vi "Copy of Sievert_auto_RLC-2.vi"() -> ()   [LabVIEW 2011]
uses:
  <vilib>/Utility/error.llb/DialogType.ctl
  <vilib>/DAQmx/write.llb/DAQmx Write (Digital Bool 1Line 1Point).vi
  <vilib>/DAQmx/create/channels.llb/DAQmx Create Channel (DO-Digital Output).vi
  <vilib>/DAQmx/miscellaneous.llb/DAQmx Fill In Error Info.vi
  <vilib>/Analysis/Matrix/Numeric/Conversions/Array To Matrix - RA.vi
  <vilib>/Analysis/Matrix/Numeric/Conversions/Matrix To Array - RM.vi
  <vilib>/Analysis/NI_AALPro.lvlib
  <vilib>/Analysis/Matrix/NI_Matrix.lvlib
  <vilib>/Analysis/NI_AALBase.lvlib
panel:
  out "Boolean 4":bool
  out "tempo carga":dbl[](array[numeric])
  out "PCh1":dbl[](array[numeric])
  out "output array 2":u32[](array[numeric])
  out "MEASURE C [F ]":dbl
  out "Automatico 2":dynamicdata(graph)
  out "termopar K 2":dbl format="%.3g"
  out "termopar K":string
  out "output NTC":dbl
  out "termopar K":dbl format="%.3g"
  out "path RLC_mean":path
  out "estagio 5":i32
  out "FIM":bool=TRUE
  out "limpo":i32
  in  "N fit":i32=5
  in  "ATM wait":u32
  in  "SET":i32
  in  "time subarray":dbl[](array[numeric])
  out "P cinetica mean 2":dbl format="%0.2f"
  out "T cinetica mean 3":dbl format="%0.2f"
  out "Time cinetica":dbl format="%0.2f"
  in  "T subarray 3":dbl[](array[numeric])
  in  "P T  index 2":i32
  in  "P subarray 2":dbl[](array[numeric])
  in  "Numeric":dbl=4.0
  in  "T subarray 2":dbl[](array[numeric])
  out "T cinetica mean 2":dbl format="%0.2f"
  out "P cinetica mean":dbl format="%0.2f"
  in  "P subarray":dbl[](array[numeric])
  in  "P T  index":i32
  out "T string":string
  out "P string":string
  out "path 2_cinetica":path
  out "Polynomial Coefficients 2":dbl[](array[numeric])
  out "Polynomial Coefficients":dbl[](array[numeric])
  in  "Count SET":i32=-1
  out "Set atual":i32
  out "mean pressure":dbl format="%.4p"
  out "Set number":i32
  in  "Tab Control":T1(tab)
  out "T":bool
  out "ZPf2":bool
  out "Pf2":bool
  out "Pit":bool
  out "ZPit":bool
  out "Camara":dbl(slide) scale=0.0..59.5 scale format="%#_3g"
  in  "Save manual":bool
  in  "Open Button":bool
  out "String 2":string
  in  "ATM":bool
  in  "Câmara":bool
  in  "Vácuo":bool
  in  "Entrada Gás":bool
  in  "Manual Ctrl":bool
  in  "stop":bool
  out "P-manual":dynamicdata(graph)
  in  "Clear":bool
  out "path":path
  in  "Nota":string
  in  "Sample name":string
  in  "File name":string
  out "Linear Model Graph":dbl[][](graph)
  out "Linear Model Graph 2":dbl[][](graph)
  in  "N to fit":i32=60
  out "N":i32
  out "Vácuo":bool
  out "Atm":bool
  out "Câmara":bool
  out "String_cinetica":string
  out "Vol Ref":dbl(slide) scale=0.0..60.0 scale format="%#_4f"
  out "Entrada gás":bool
  in  "Guardar\nCinetica":bool
  out "p fit":dbl format="%#_4g"
  out "T fit":dbl format="%#_4g"
  in  "Open Button 2":bool
  out "x >= y?":bool
  in  "seconds":dbl
  out "Elapsed Time (sec)":dbl format="%.1f"
  out "bar/N":dbl format="%#_4p"
  in  "correção NTC":dbl
  out "mean H2 sensor (V)":dbl format="%#_4p"
  out "Boolean 3":bool
  out "String 3":string
  out "T 2":bool
  out "ZPit 2":bool
  out "Pit 2":bool
  out "Pf2 2":bool
  out "ZPf2 2":bool
  out "Camara 2":dbl(slide) scale=0.0..20.0 scale format="%#_3g"
  out "Vácuo 2":bool
  out "Atm 2":bool
  out "Câmara 2":bool
  out "Vol Ref 3":dbl(slide) scale=0.0..25.0 scale format="%#_4f"
  out "Entrada gás 2":bool
  in  "Auto Ctrl":bool
  in  "Play Button":bool
  out "time stamp":timestamp format="%<%.2X>T"
  out "Time (sec)":dbl format="%.1f"
  in  "clear":bool
  out "Automatico":dynamicdata(graph)
  out "Linear P":T2(graph)
  out "Linear T":T2(graph)
  out "Contador":i32
  in  "STOP (bar/s)":dbl format="%#_5p"
  out "P (bar/s)":dbl format="%#_5p"
  out "bar/s":dbl format="%#_4p"
  out "P fit":dbl format="%#_4g"
  out "T fit":dbl format="%#_4g"
  out "x = y?":bool
  out "teste slope":i32
  in  "Set P auto":dbl
  in  "Step P":dbl=2.0
  in  "P_max":dbl=2.0
  in  "P_max camara":dbl=2.0
  out "Carga":bool=TRUE
  out "Descarga":bool
  out "String":string
  in  "P_min descarga":dbl
  in  "Boolean":bool
  in  "Array":dbl[](array[numeric])
  out "Boolean 2":bool
  out "Desc SET":i32
  in  "ZPf2 time":dbl=24.0
  in  "Ciclos":dbl
  out "Efetuados":dbl
  in  "patamar milliseconds to wait":u32=500
  in  "N fit patamar":i32=100
  in  "Step ZPit":dbl
  out "Read ZPit":bool
  in  "Estagio auto":i32
  out "mean H2 sensor":dbl format="%#_4p"
  in  "Ntest":i32=5
  in  "N fit 2":i32=100
  out "String 4":string
  in  "Combo Box":string(combo)
  in  "Refresh Button":bool
  in  "Close RLC 2":bool
  in  "RLC on/off":bool
  out "mean 16":dbl format="%.3p"
  out "mean 15":dbl format="%.3p"
  out "mean 14":dbl format="%.3p"
  out "mean 13":dbl format="%.3p"
  out "mean 12":dbl format="%.3p"
  out "mean 11":dbl format="%.3p"
  out "mean 10":dbl format="%.3p"
  out "mean 9":dbl format="%.3p"
  out "mean 8":dbl format="%.3p"
  out "mean 7":dbl format="%.3p"
  out "mean 6":dbl format="%.3p"
  out "mean 5":dbl format="%.3p"
  out "mean 4":dbl format="%.3p"
  out "mean 3":dbl format="%.3p"
  out "mean 2":dbl format="%.3p"
  out "mean":dbl format="%.3p"
  out "SET 2":dbl format="%#_3g"
  out "C-50-L":bool
  out "MEASURE B":dbl
  out "MEASURE A":dbl
  out "C-50-N":bool
  out "MEASURE B 2":dbl
  out "MEASURE A 2":dbl
  out "C-100-L":bool
  out "MEASURE B 3":dbl
  out "MEASURE A 3":dbl
  out "C-100-N":bool
  out "MEASURE B 4":dbl
  out "MEASURE A 4":dbl
  out "C-1K-L":bool
  out "MEASURE B 5":dbl
  out "MEASURE A 5":dbl
  out "C-1K-N":bool
  out "MEASURE B 6":dbl
  out "MEASURE A 6":dbl
  out "C-10K-L":bool
  out "MEASURE B 7":dbl
  out "MEASURE A 7":dbl
  out "C-10K-N":bool
  out "MEASURE B 8":dbl
  out "MEASURE A 8":dbl
  out "Z-50-L":bool
  out "MEASURE B 9":dbl
  out "MEASURE A 9":dbl
  out "Z-50-N":bool
  out "MEASURE B 10":dbl
  out "MEASURE A 10":dbl
  out "Z-100-L":bool
  out "MEASURE B 11":dbl
  out "MEASURE A 11":dbl
  out "Z-100-N":bool
  out "MEASURE B 12":dbl
  out "MEASURE A 12":dbl
  out "Z-1K-L":bool
  out "MEASURE B 13":dbl
  out "MEASURE A 13":dbl
  out "Z-1K-N":bool
  out "MEASURE B 14":dbl
  out "MEASURE A 14":dbl
  out "Z-10K-L":bool
  out "MEASURE B 15":dbl
  out "MEASURE A 15":dbl
  out "Z-10K-N":bool
  out "MEASURE B 16":dbl
  out "MEASURE A 16":dbl
  out "RLC300 - digimess":string
  in  "Time RLC":u32=5000
  in  "Ligar RLC":bool
  out "path RLC_completo":path
  out "Waveform Chart P 2":dbl[][](graph)
  out "Waveform Chart":dynamicdata(graph)
  in  "graph RLC":bool
  in  "Refresh Button 2":bool
  out "Waveform Chart 2":dynamicdata(graph)
  out "XY Graph 2":cluster{"Value":dbl[], "Value":dbl[]}[](graph)
  in  "t-sivert01(s)":dbl
  out "dP/dt (bar/s)":dbl format="%#_5p"
  in  "read - Sievert 01":bool
  # "P vol ref"
  # "P Câmara"
  # "P vol ref"
  # "P Câmara"
  # "C ( F )"
  # "R ( Ohm )"
  # "Z ( Ohm )"
  # "Phase ( deg)"
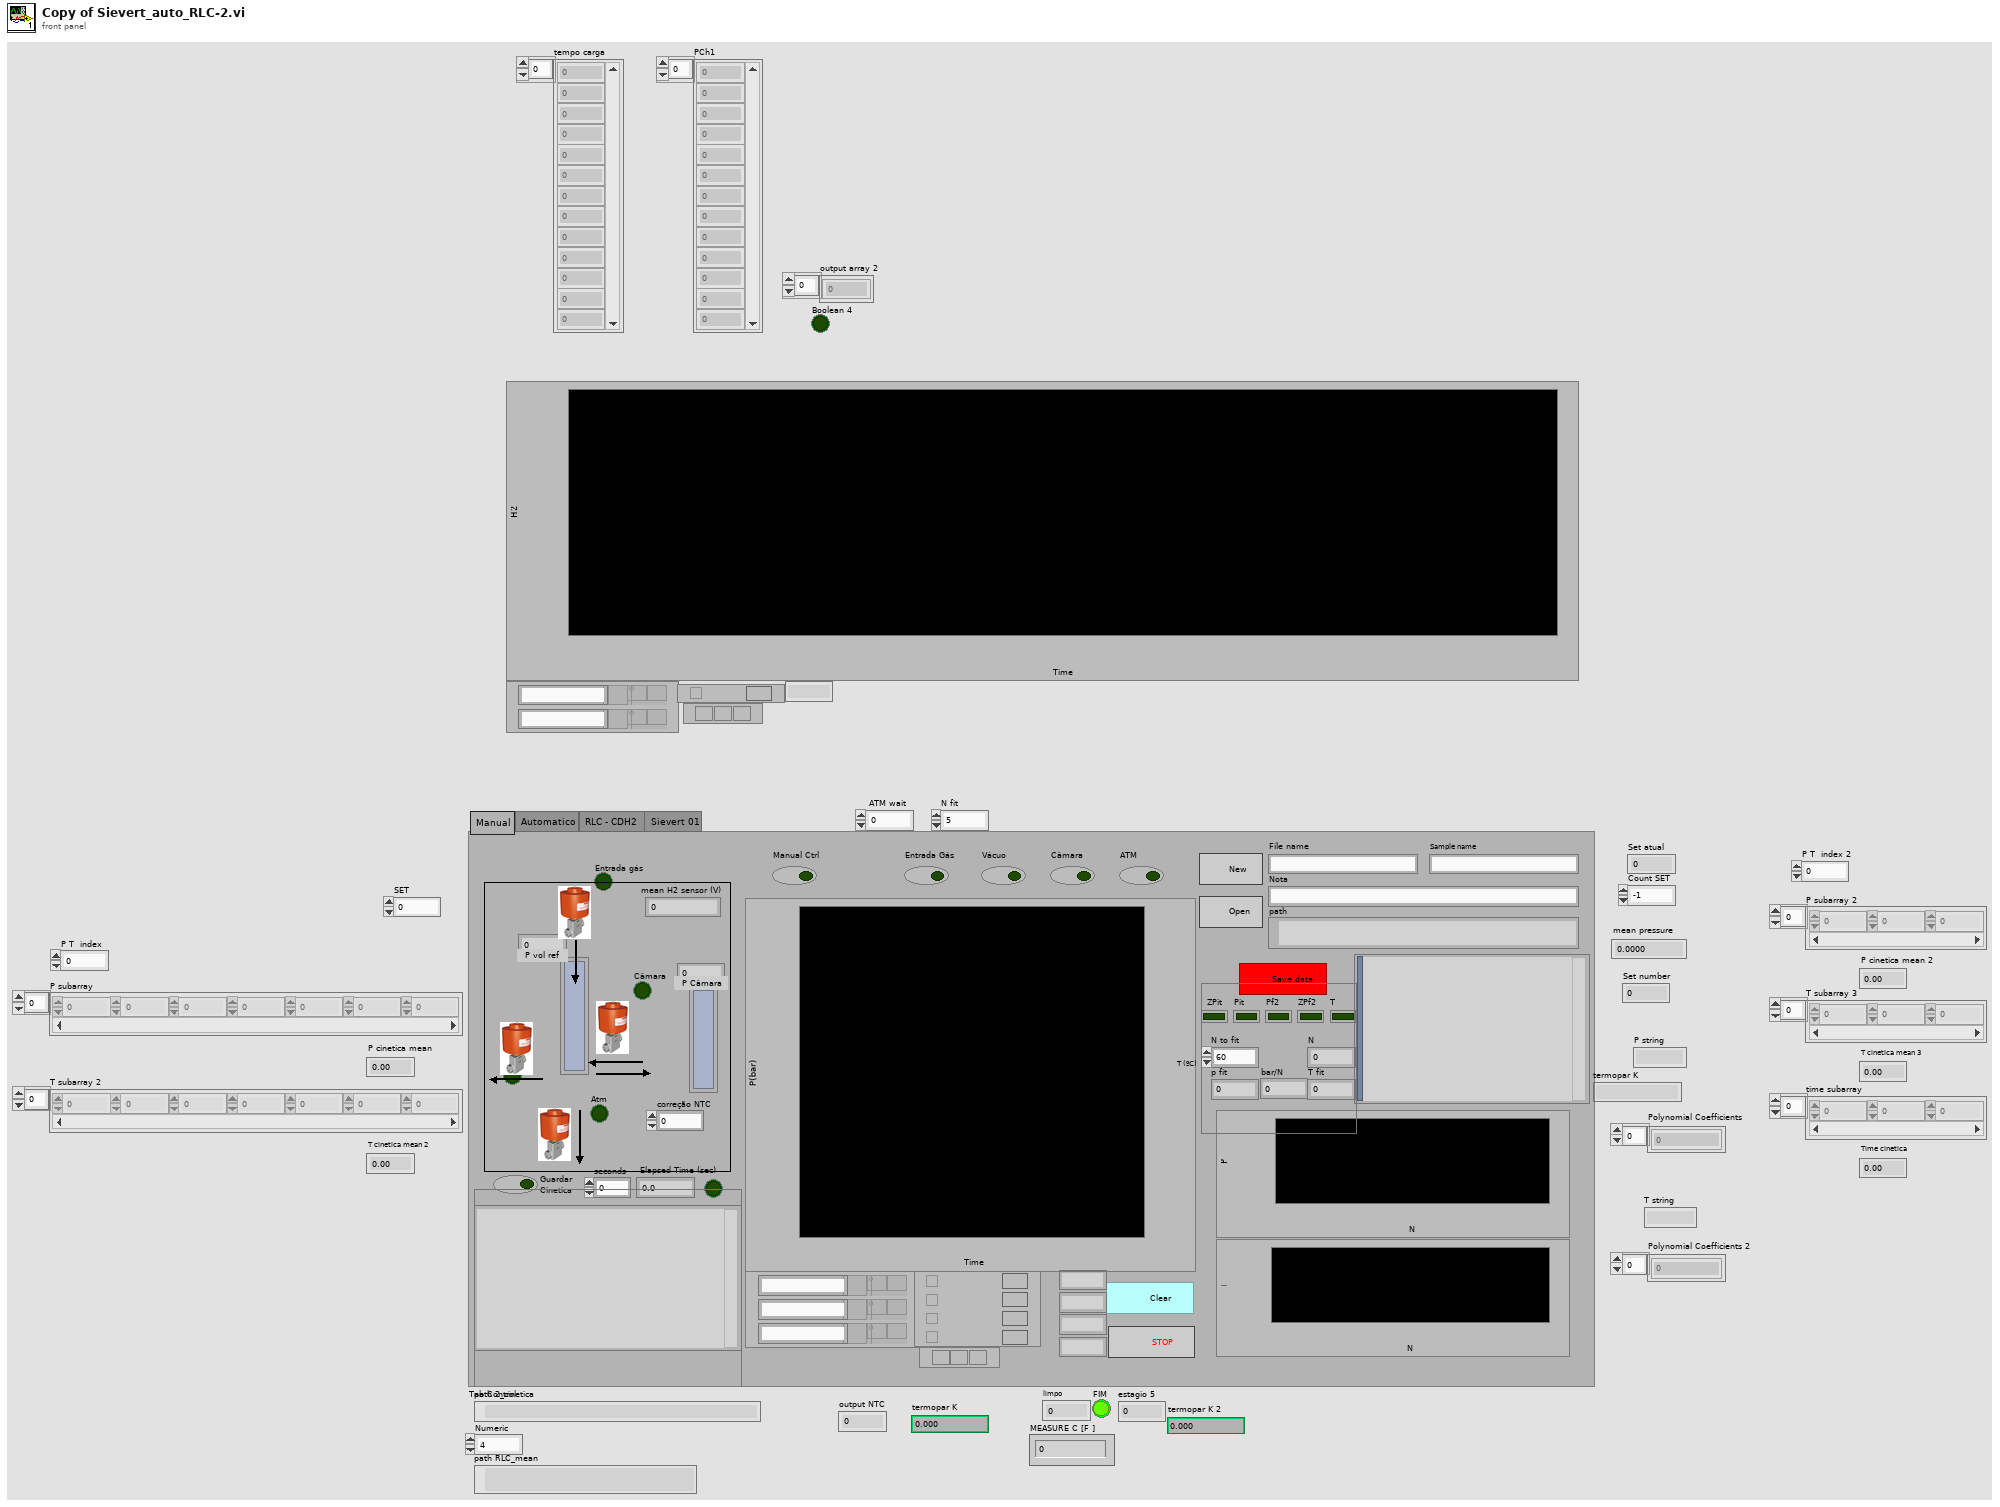
[diagram p1: front panel]
types:
  T1 = enum32{"Manual", "Automatico", "RLC - CDH2", "Sievert 01"}
  T2 = cluster{"Real 2D Array":dbl[], "Best Linear Fit":dbl[]}[]
  T3 = enum16{"open", "replace", "create", "open or create", "replace or create", "replace or create with confirmation"}
  T4 = cluster{"Value":dbl[], "Best Linear Fit":dbl[]}[]
  T5 = typedef "NI_Matrix.lvlib/RealMatrix.ctl" = dbl[][]
  T6 = cluster{"Real 2D Array":dbl[], "Real 2D Array":dbl[]}
  T7 = typedef "DialogType.ctl" = u16
  T8 = cluster{"Real 2D Array":dbl[], "Best Linear Fit":dbl[]}
  T9 = cluster{"Real 2D Array":dbl[], "Best Polynomial Fit":dbl[]}
  T10 = cluster{"Real 2D Array":dbl[], "Best Polynomial Fit":dbl[]}[]
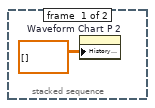
[diagram p5: hidden frame]
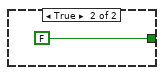
[diagram p10: hidden frame]
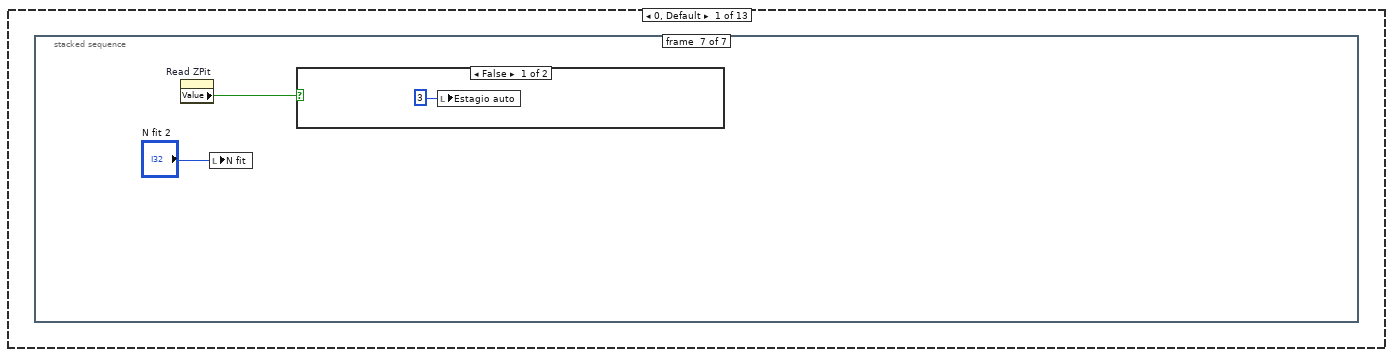
[diagram p15: hidden frame]
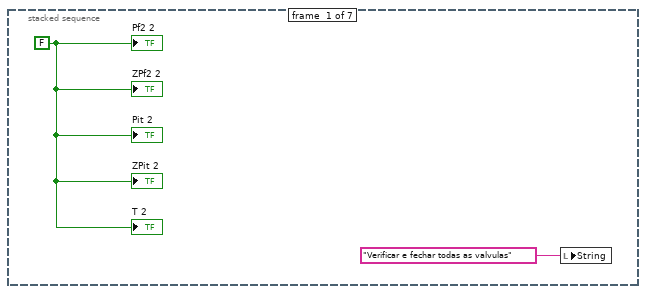
[diagram p16: hidden frame]
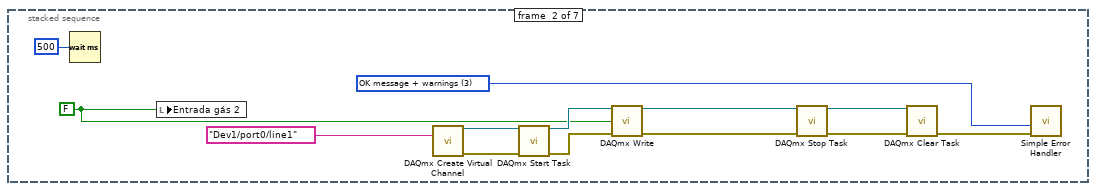
[diagram p17: hidden frame]
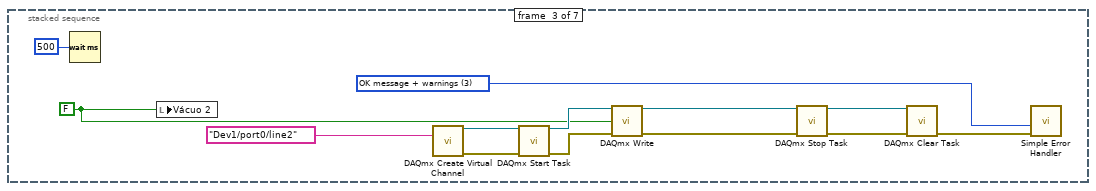
[diagram p18: hidden frame]
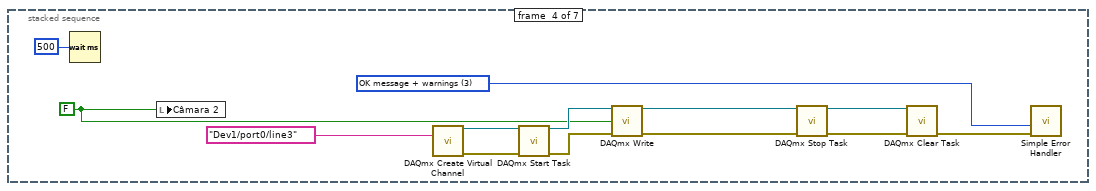
[diagram p19: hidden frame]
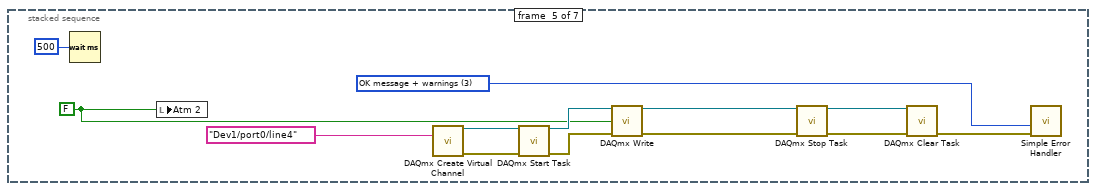
[diagram p20: hidden frame]
diagram:
  (unwired) dbl[] [0.5, 1.0, 2.0, 3.0, 4.0, 5.0, 6.0, 7.0, 8.0, 9.0, 10.0, 11.0, 12.0, 13.0, 14.0, 15.0, 16.0, 17.0, 18.0, 19.0, 20.0, 30.0, 40.0, 50.0, 60.0, 70.0] ("Array")
  n1 = local write "N to fit"(5 ("Numeric")) -> ()
  n2 = local write "correção NTC"(0.5 ("correção NTC")) -> ()
  n3 = local write "Step ZPit"(5.0 ("Step ZPit")) -> ()
  n4 = local write "Time RLC"(u32 5 ("Time RLC")) -> ()
  n5 = local write "Ciclos"(0.0 ("Ciclos")) -> ()
  n6 = local write "Desc SET"(0 ("Desc SET")) -> ()
  n7 = local write "Efetuados"(0.0 ("Efetuados")) -> ()
  n8 = local write "estagio 5"(0 ("estagio 5")) -> ()
  n9 = local write "teste slope"(0 ("teste slope")) -> ()
  n10 = local write "SET"(0 ("SET auto")) -> ()
  n11 = local write "limpo"(0 ("limpo")) -> ()
  n12 = local write "N fit"(5 ("N fit")) -> ()
  n13 = local write "ATM wait"(u32 4 ("ATM wait")) -> ()
  n14 = local write "Estagio auto"(0 ("Estagio auto")) -> ()
  n15 = local write "P T  index"(0 ("index")) -> ()
  n16 = local write "seconds"(2.0 ("seconds")) -> ()
  n17 = local write "Read ZPit"(TRUE ("Read ZPit")) -> ()
  n18 = local write "Descarga"(FALSE ("Descarga")) -> ()
  n19 = local write "Carga"(TRUE ("Carga")) -> ()
  n20 = local write "FIM"(FALSE ("FIM")) -> ()
  n21 = local write "P_max"(50.0 ("P_max")) -> ()
  n22 = local write "P_max camara"(25.0 ("P_max camara")) -> ()
  n23 = local write "Set P auto"(0.5 ("Set P auto")) -> ()
  n24 = local write "P_min descarga"(0.025 ("P_min descarga")) -> ()
  n25 = local write "P subarray"(dbl[] [0.0, 1.0] ("subarray")) -> ()
  n26 = local write "T subarray 2"(dbl[] [0.0, 1.0] ("subarray")) -> ()
  n27 = local write "Combo Box"("rlc_read_cCN.py" ("Combo Box")) -> ()
  n28 = local write "t-sivert01(s)"(10.0 ("t-sivert01(s)")) -> ()
  n29 = while {
    tunnel: path "C:/H2_Painel/painel_auto/RLC_CDH" ("Path") -> [w36]
    stop <- w48 stop-if-true
    n30 = property on="FIM" class="Bool (strict)"() -> ("Value"=w46:bool)  [unwired: 2 in, 2 out]
    n31 = property on="path" class="Path"() -> ("Value"=w43:path)  [unwired: 2 in, 2 out]
    n32 = case shown="True" "Ligar RLC" {
      tunnel: w36 -> [_ w223]
      frame False {
      }
      frame True {
        n33 = call "RLC_open.vi"("Path"=w223) -> ("String 2"=w224:string)  [unwired: 9 in, 1 out]
        n34 = local write "RLC300 - digimess"(w224) -> ()
      }
    }
    n35 = case shown="True" "Auto Ctrl" {
      tunnel: w36 -> [_ w229]
      tunnel: "RLC on/off" -> [_ w228]
      tunnel: [_ w227] -> w39
      frame False {
      }
      frame True {
        n36 = local write "P T  index 2"(0 ("P T  index")) -> ()
        n37 = for {
          N: "N fit" -> [w256]
          tunnel: w229 -> [w247]
          tunnel: w228 -> [w246]
          tunnel: [w245] -> w227
          i -> [w258]
          w262 = 0 ("polynomial order")
          w253 = 0 ("polynomial order")
          n38 = case shown="True" "clear" {
            frame False {
            }
            frame True {
              n39 = property on="Automatico 2" class="WFChart (strict)"("History Data"=dynamicdata[] []) -> ()  [unwired: 2 in, 2 out]
              n40 = property on="Linear P" class="XYGraph (strict)"("Value"=T2 [] ("Linear P")) -> ()  [unwired: 2 in, 2 out]
              n41 = property on="Linear T" class="XYGraph (strict)"("Value"=T2 [] ("Linear T")) -> ()  [unwired: 2 in, 2 out]
              n42 = property on="Automatico" class="WFChart (strict)"("History Data"=dynamicdata[] []) -> ()  [unwired: 2 in, 2 out]
            }
          }
          n43 = property on="path 2_cinetica" class="Path"() -> ("Value"=w250:path)  [unwired: 2 in, 2 out]
          n44 = call "Read P T.vi"("correção NTC"="correção NTC") -> ("Sievert01"=w237:dbl, "mean H2 sensor"=w242:dbl, "termopar K"=w239:dbl, "output NTC"=w240:dbl, "P Set 2 Output 2"=w241:dbl)  [unwired: 3 in, 7 out]
          "termopar K 2" <- w239
          "mean H2 sensor" <- w242
          n45 = Increment(x=w258) -> (x+1=w257:i32)
          n46 = Equal?(x=w257, y=w256) -> (x = y?=w259:bool)
          "x = y?" <- w259
          n47 = Merge Signals(w242) -> (→"Automatico 2":dynamicdata)
          n48 = Multiply(x=w241, y=10.0) -> (x*y=w252:dbl)
          n49 = Multiply(x=w237, y=10.0) -> (x*y=w236:dbl)
          n50 = case shown="True" "read - Sievert 01" {
            tunnel: w236 -> [_ w285]
            frame False {
            }
            frame True {
              n51 = Merge Signals(w285) -> (→"Waveform Chart 2":dynamicdata)
              n52 = flat-sequence {
                tunnel: w285 -> [w302]
                tunnel: [w300] -> w287
                frame #0 {
                  n53 = property on="Boolean 4" class="Bool (strict)"() -> ("Value"=w288:bool)  [unwired: 2 in, 2 out]
                  n54 = case shown="True" w288 {
                    frame False {
                    }
                    frame True {
                      n55 = local write "PCh1"(dbl[] [] ("PCh1")) -> ()
                      n56 = local write "tempo carga"(dbl[] [] ("tempo carga")) -> ()
                      n57 = local write "output array 2"(u32[] [] ("output array 2")) -> ()
                    }
                  }
                }
                frame #1 {
                  n58 = Tick Count (ms)() -> (millisecond timer value=w313:u32)
                  n59 = property on="output array 2" class="Arr (strict)"() -> ("Value"=w314:u32[])  [unwired: 2 in, 2 out]
                  n60 = Build Array(w313) -> (w307:u32[])
                  n61 = Insert Into Array(array=w314, new element=w307) -> (w308:u32[])  [unwired: 1 in]
                  "output array 2" <- w308
                  n62 = Array Max & Min(array=w308) -> (max value=w312:u32, min value=w311:u32)  [unwired: 2 out]
                  n63 = Subtract(x=w312, y=w311) -> (x-y=w309:u32)
                  n64 = Divide(x=w309, y=1000.0) -> (x/y=w299:dbl)
                  n65 = property on="PCh1" class="Arr (strict)"() -> ("Value"=w304:dbl[])  [unwired: 2 in, 2 out]
                  n66 = property on="tempo carga" class="Arr (strict)"() -> ("Value"=w305:dbl[])  [unwired: 2 in, 2 out]
                  n67 = Greater?(x=w299, y="t-sivert01(s)") -> (0:w300:bool)
                  n68 = Build Array(w299) -> (w306:dbl[])
                  n69 = Build Array(w302) -> (w303:dbl[])
                  n70 = Insert Into Array(array=w305, new element=w306) -> (w294:dbl[])  [unwired: 1 in]
                  "tempo carga" <- w294
                  n71 = Insert Into Array(array=w304, new element=w303) -> (w293:dbl[])  [unwired: 1 in]
                  "PCh1" <- w293
                  n72 = call <vilib>:"Linear Fit.vi"("Y"=w293, "X"=w294) -> ("Best Linear Fit"=w292:dbl[], "slope"=→"dP/dt (bar/s)":dbl)  [unwired: 9 in, 3 out]
                  n73 = Bundle("Value"=w294, "Value"=w293) -> (w297:cluster{"Value":dbl[], "Value":dbl[]})  [unwired: 1 in]
                  n74 = Bundle("Value"=w294, "Best Linear Fit"=w292) -> (w296:cluster{"Value":dbl[], "Best Linear Fit":dbl[]})  [unwired: 1 in]
                  n75 = Build Array(w297, w296) -> (→"XY Graph 2":T4)
                }
              }
              "Boolean 4" <- w287
            }
          }
          n76 = local write "Vol Ref 3"(w252) -> ()
          n77 = Merge Signals(w252, w240, w239, w236) -> (→"Automatico":dynamicdata)
          n78 = call "Elapsed Time2"("Reset"=w259) -> ("Elapsed Time (s)"=w273:dbl)  [unwired: 11 in, 7 out]
          "Time (sec)" <- w273
          n79 = stacked-sequence {
            tunnel: w252 -> [w1724 _]
            tunnel: w240 -> [w1710 _]
            tunnel: [w1691 _] -> w271
            tunnel: [w1707 _] -> w270
            tunnel: w273 -> [w1694 _]
            tunnel: [w1692 _] -> w267
            tunnel: [w1690 _] -> w249
            tunnel: [w1689 _] -> w248
            frame #0 {
              w1693 = 2 ("y")
              n80 = property on="P subarray 2" class="Arr (strict)"() -> ("Value"=w1726:dbl[])  [unwired: 2 in, 2 out]
              n81 = property on="T subarray 3" class="Arr (strict)"() -> ("Value"=w1716:dbl[])  [unwired: 2 in, 2 out]
              n82 = property on="time subarray" class="Arr (strict)"() -> ("Value"=w1703:dbl[])  [unwired: 2 in, 2 out]
              n83 = property on="P T  index 2" class="DigNum (strict)"() -> ("Value"=w1695:i32)  [unwired: 2 in, 2 out]
              n84 = Replace Array Subset(array=w1703, new element=w1694, index=w1695) -> (w1696:dbl[])
              n85 = Replace Array Subset(array=w1726, new element=w1724, index=w1695) -> (w1709:dbl[])
              n86 = Replace Array Subset(array=w1716, new element=w1710, index=w1695) -> (w1708:dbl[])
              n87 = call-poly <vilib>:"Array To Matrix.vi"("Real 1D Array"=w1696) -> ("Real Matrix (Column Vector)"=w1706:T5)
              n88 = call-poly <vilib>:"Array To Matrix.vi"("Real 1D Array"=w1709) -> ("Real Matrix (Column Vector)"=w1729:T5)
              n89 = call-poly <vilib>:"Array To Matrix.vi"("Real 1D Array"=w1708) -> ("Real Matrix (Column Vector)"=w1719:T5)
              n90 = Matrix Size(0:w1706) -> (1:w1705:i32, 2:w1704:i32)
              n91 = Matrix Size(0:w1729) -> (1:w1728:i32, 2:w1727:i32)
              n92 = Matrix Size(0:w1719) -> (1:w1718:i32, 2:w1717:i32)
              n93 = Increment(x=w1705) -> (x+1=w1697:i32)
              n94 = Increment(x=w1728) -> (x+1=w1720:i32)
              n95 = Increment(x=w1718) -> (x+1=w1711:i32)
              n96 = Subtract(x=w1697, y=w1693) -> (x-y=w1698:i32)
              n97 = Subtract(x=w1720, y=w1693) -> (x-y=w1721:i32)
              n98 = Subtract(x=w1711, y=w1693) -> (x-y=w1712:i32)
              n99 = Resize Matrix(1:w1704, 2:w1697, 4:w1706) -> (0:w1702:T5)
              n100 = Resize Matrix(1:w1727, 2:w1720, 4:w1729) -> (0:w1725:T5)
              n101 = Resize Matrix(1:w1717, 2:w1711, 4:w1719) -> (0:w1715:T5)
              n102 = call-poly <vilib>:"Matrix To Array.vi"("Real Matrix"=w1702) -> ("Real 2D Array"=w1700:dbl[][])
              n103 = call-poly <vilib>:"Matrix To Array.vi"("Real Matrix"=w1725) -> ("Real 2D Array"=w1723:dbl[][])
              n104 = call-poly <vilib>:"Matrix To Array.vi"("Real Matrix"=w1715) -> ("Real 2D Array"=w1714:dbl[][])
              n105 = Reshape Array(w1700, w1697) -> (w1699:dbl[])
              n106 = Reshape Array(w1723, w1720) -> (w1722:dbl[])
              n107 = Reshape Array(w1714, w1711) -> (w1713:dbl[])
              n108 = local write "time subarray"(w1699) -> ()
              n109 = local write "P subarray 2"(w1722) -> ()
              n110 = local write "T subarray 3"(w1713) -> ()
              n111 = Reshape Array(w1699, w1698) -> (w1692:dbl[])
              n112 = Reshape Array(w1722, w1721) -> (w1691:dbl[])
              n113 = Reshape Array(w1713, w1712) -> (w1707:dbl[])
              n114 = call <vilib>:"Mean.vi"("X"=w1692) -> ("mean"=→"Time cinetica":dbl)  [unwired: 1 out]
              n115 = call <vilib>:"Mean.vi"("X"=w1691) -> ("mean"=w1690:dbl)  [unwired: 1 out]
              "P cinetica mean 2" <- w1690
              n116 = call <vilib>:"Mean.vi"("X"=w1707) -> ("mean"=w1689:dbl)  [unwired: 1 out]
              "T cinetica mean 3" <- w1689
            }
            frame #1 {
              n117 = property on="P T  index 2" class="DigNum (strict)"() -> ("Value"=w1731:i32)  [unwired: 2 in, 2 out]
              n118 = Increment(x=w1731) -> (x+1=w1730:i32)
              n119 = local write "P T  index 2"(w1730) -> ()
            }
          }
          n120 = To Time Stamp(1:w273) -> (0:→"time stamp":timestamp)
          n121 = call <vilib>:"Linear Fit.vi"("Y"=w270, "X"=w267) -> ("Best Linear Fit"=w279:dbl[])  [unwired: 9 in, 4 out]
          n122 = Bundle("Real 2D Array"=w267, "Real 2D Array"=w270) -> (w277:T6)  [unwired: 1 in]
          n123 = Bundle("Real 2D Array"=w267, "Real 2D Array"=w271) -> (w276:T6)  [unwired: 1 in]
          n124 = call <vilib>:"General Polynomial Fit.vi"("Y"=w270, "polynomial order"=w253, "X"=w267) -> ("Best Polynomial Fit"=w268:dbl[], "Polynomial Coefficients"=w263:dbl[])  [unwired: 9 in, 2 out]
          n125 = call <vilib>:"General Polynomial Fit.vi"("Y"=w271, "polynomial order"=w253, "X"=w267) -> ("Best Polynomial Fit"=w269:dbl[], "Polynomial Coefficients"=w264:dbl[])  [unwired: 9 in, 2 out]
          n126 = call <vilib>:"Linear Fit.vi"("Y"=w271, "X"=w267) -> ("Best Linear Fit"=w274:dbl[], "slope"=w254:dbl)  [unwired: 9 in, 3 out]
          "bar/s" <- w254
          n127 = property on="path" class="Path"() -> ("Value"=w251:path)  [unwired: 2 in, 2 out]
          n128 = case shown="True" "Play Button" {
            tunnel: w251 -> [_ w323]
            tunnel: w252 -> [_ w322]
            tunnel: w250 -> [_ w321]
            tunnel: w249 -> [_ w320]
            tunnel: w248 -> [_ w319]
            tunnel: w247 -> [_ w318]
            tunnel: w246 -> [_ w317]
            tunnel: [_ w316] -> w245
            tunnel: w239 -> [_ w315]
            frame False {
            }
            frame True {
              n129 = case shown="7" "Estagio auto" {
                tunnel: w323 -> [_ _ _ w415 _ _ w568 _ w818 _ _ w1530 w1599]
                tunnel: w322 -> [_ w389 _ _ w464 w515 _ _ _ w1448 _ _ _]
                tunnel: w321 -> [_ _ _ _ _ _ _ w610 _ _ _ _ _]
                tunnel: w320 -> [_ _ _ _ _ _ _ w609 _ _ _ _ _]
                tunnel: w319 -> [_ _ _ _ _ _ _ w608 _ _ _ _ _]
                tunnel: w318 -> [_ _ _ _ _ _ _ _ w797 _ _ _ _]
                tunnel: w317 -> [_ _ _ _ _ _ _ _ w814 _ _ _ _]
                tunnel: [_ _ _ _ _ _ _ _ w796 _ _ _ _] -> w316
                tunnel: w315 -> [_ _ _ _ _ _ _ _ _ _ _ w1526 _]
                frame 0, Default {
                  n130 = stacked-sequence {
                    frame #0 {
                      w325 = FALSE ("Pit")
                      n131 = local write "String"("Verificar e fechar todas as valvulas" ("String")) -> ()
                      "ZPf2 2" <- w325
                      "Pf2 2" <- w325
                      "Pit 2" <- w325
                      "ZPit 2" <- w325
                      "T 2" <- w325
                    }
                    frame #1 {
                      w328 = FALSE ("Boolean 4")
                      w333 = T7 3 items=["no dialog", "OK message", "continue or stop message", "OK message + warnings", "continue/stop + warnings"] ("type of dialog (OK msg:1)")
                      n132 = Wait (ms)(milliseconds to wait=u32 500) -> ()  [unwired: 1 out]
                      n133 = local write "Entrada gás 2"(w328) -> ()
                      n134 = call-poly <vilib>:"DAQmx Create Virtual Channel.vi"("lines"=tag "Dev1/port0/line1") -> ("task out"=w331:refnum<k21>, "error out"=w332:errorcluster)  [unwired: 13 in]
                      n135 = call <vilib>:"DAQmx Start Task.vi"("task/channels in"=w331, "error in"=w332) -> ("task out"=w334:refnum<k21>, "error out"=w335:errorcluster)  [unwired: 12 in]
                      n136 = call-poly <vilib>:"DAQmx Write.vi"("task/channels in"=w334, "data"=w328, "error in"=w335) -> ("task out"=w339:refnum<k21>, "error out"=w336:errorcluster)  [unwired: 10 in, 1 out]
                      n137 = call <vilib>:"DAQmx Stop Task.vi"("task/channels in"=w339, "error in"=w336) -> ("task out"=w338:refnum<k21>, "error out"=w337:errorcluster)  [unwired: 12 in]
                      n138 = call <vilib>:"DAQmx Clear Task.vi"("task in"=w338, "error in"=w337) -> ("error out"=w330:errorcluster)  [unwired: 13 in]
                      n139 = call <vilib>:"Simple Error Handler.vi"("type of dialog (OK msg:1)"=w333, "error in (no error)"=w330) -> ()  [unwired: 3 in, 5 out]
                    }
                    frame #2 {
                      w341 = FALSE ("Boolean 4")
                      w346 = T7 3 items=["no dialog", "OK message", "continue or stop message", "OK message + warnings", "continue/stop + warnings"] ("type of dialog (OK msg:1)")
                      n140 = Wait (ms)(milliseconds to wait=u32 500) -> ()  [unwired: 1 out]
                      n141 = local write "Vácuo 2"(w341) -> ()
                      n142 = call-poly <vilib>:"DAQmx Create Virtual Channel.vi"("lines"=tag "Dev1/port0/line2") -> ("task out"=w344:refnum<k21>, "error out"=w345:errorcluster)  [unwired: 13 in]
                      n143 = call <vilib>:"DAQmx Start Task.vi"("task/channels in"=w344, "error in"=w345) -> ("task out"=w347:refnum<k21>, "error out"=w348:errorcluster)  [unwired: 12 in]
                      n144 = call-poly <vilib>:"DAQmx Write.vi"("task/channels in"=w347, "data"=w341, "error in"=w348) -> ("task out"=w352:refnum<k21>, "error out"=w349:errorcluster)  [unwired: 10 in, 1 out]
                      n145 = call <vilib>:"DAQmx Stop Task.vi"("task/channels in"=w352, "error in"=w349) -> ("task out"=w351:refnum<k21>, "error out"=w350:errorcluster)  [unwired: 12 in]
                      n146 = call <vilib>:"DAQmx Clear Task.vi"("task in"=w351, "error in"=w350) -> ("error out"=w343:errorcluster)  [unwired: 13 in]
                      n147 = call <vilib>:"Simple Error Handler.vi"("type of dialog (OK msg:1)"=w346, "error in (no error)"=w343) -> ()  [unwired: 3 in, 5 out]
                    }
                    frame #3 {
                      w354 = FALSE ("Boolean 4")
                      w359 = T7 3 items=["no dialog", "OK message", "continue or stop message", "OK message + warnings", "continue/stop + warnings"] ("type of dialog (OK msg:1)")
                      n148 = Wait (ms)(milliseconds to wait=u32 500) -> ()  [unwired: 1 out]
                      n149 = local write "Câmara 2"(w354) -> ()
                      n150 = call-poly <vilib>:"DAQmx Create Virtual Channel.vi"("lines"=tag "Dev1/port0/line3") -> ("task out"=w357:refnum<k21>, "error out"=w358:errorcluster)  [unwired: 13 in]
                      n151 = call <vilib>:"DAQmx Start Task.vi"("task/channels in"=w357, "error in"=w358) -> ("task out"=w360:refnum<k21>, "error out"=w361:errorcluster)  [unwired: 12 in]
                      n152 = call-poly <vilib>:"DAQmx Write.vi"("task/channels in"=w360, "data"=w354, "error in"=w361) -> ("task out"=w365:refnum<k21>, "error out"=w362:errorcluster)  [unwired: 10 in, 1 out]
                      n153 = call <vilib>:"DAQmx Stop Task.vi"("task/channels in"=w365, "error in"=w362) -> ("task out"=w364:refnum<k21>, "error out"=w363:errorcluster)  [unwired: 12 in]
                      n154 = call <vilib>:"DAQmx Clear Task.vi"("task in"=w364, "error in"=w363) -> ("error out"=w356:errorcluster)  [unwired: 13 in]
                      n155 = call <vilib>:"Simple Error Handler.vi"("type of dialog (OK msg:1)"=w359, "error in (no error)"=w356) -> ()  [unwired: 3 in, 5 out]
                    }
                    frame #4 {
                      w367 = FALSE ("Boolean 4")
                      w372 = T7 3 items=["no dialog", "OK message", "continue or stop message", "OK message + warnings", "continue/stop + warnings"] ("type of dialog (OK msg:1)")
                      n156 = Wait (ms)(milliseconds to wait=u32 500) -> ()  [unwired: 1 out]
                      n157 = local write "Atm 2"(w367) -> ()
                      n158 = call-poly <vilib>:"DAQmx Create Virtual Channel.vi"("lines"=tag "Dev1/port0/line4") -> ("task out"=w370:refnum<k21>, "error out"=w371:errorcluster)  [unwired: 13 in]
                      n159 = call <vilib>:"DAQmx Start Task.vi"("task/channels in"=w370, "error in"=w371) -> ("task out"=w373:refnum<k21>, "error out"=w374:errorcluster)  [unwired: 12 in]
                      n160 = call-poly <vilib>:"DAQmx Write.vi"("task/channels in"=w373, "data"=w367, "error in"=w374) -> ("task out"=w378:refnum<k21>, "error out"=w375:errorcluster)  [unwired: 10 in, 1 out]
                      n161 = call <vilib>:"DAQmx Stop Task.vi"("task/channels in"=w378, "error in"=w375) -> ("task out"=w377:refnum<k21>, "error out"=w376:errorcluster)  [unwired: 12 in]
                      n162 = call <vilib>:"DAQmx Clear Task.vi"("task in"=w377, "error in"=w376) -> ("error out"=w369:errorcluster)  [unwired: 13 in]
                      n163 = call <vilib>:"Simple Error Handler.vi"("type of dialog (OK msg:1)"=w372, "error in (no error)"=w369) -> ()  [unwired: 3 in, 5 out]
                    }
                    frame #5 {
                      n164 = Wait (ms)(milliseconds to wait=u32 500) -> ()  [unwired: 1 out]
                    }
                    frame #6 {
                      n165 = property on="Read ZPit" class="Bool (strict)"() -> ("Value"=w381:bool)  [unwired: 2 in, 2 out]
                      n166 = local write "N fit"("N fit 2") -> ()
                      n167 = case shown="False" w381 {
                        frame False {
                          n168 = local write "Estagio auto"(3 ("Estagio auto")) -> ()
                        }
                        frame True {
                          n169 = local write "Estagio auto"(1 ("Estagio auto")) -> ()
                        }
                      }
                    }
                  }
                }
                frame 1 {
                  n170 = Greater?(x=w389, y=1.0) -> (0:w388:bool)
                  n171 = case shown="True" w388 {
                    tunnel: [FALSE ("Boolean") TRUE ("Boolean")] -> w385
                    frame False {
                      w401 = TRUE ("Boolean")
                      n172 = local write "Vácuo 2"(w401) -> ()
                      n173 = call "Controle_vacuo.vi"("time (s) to wait vacuo"=u32 5, "Boolean"=w401) -> ("Vacuo"=w402:bool)  [unwired: 9 in]
                      n174 = local write "Vácuo 2"(w402) -> ()
                      n175 = local write "String"("Limpar volume referencia" ("String")) -> ()
                    }
                    frame True {
                      n176 = call "Controle_ATM.vi"("seconds to wait"="ATM wait") -> ("String 2"=w406:string, "Atm"=w405:bool)  [unwired: 9 in]
                      n177 = local write "Atm 2"(w405) -> ()
                      n178 = local write "String"(w406) -> ()
                    }
                  }
                  n179 = for {
                    N: 1 -> [_]
                    tunnel: [w391] -> w386
                    tunnel: w385 -> [w391]
                    n180 = Wait (ms)(milliseconds to wait=u32 500 ("x")) -> ()  [unwired: 1 out]
                  }
                  n181 = case shown="True" w386 {
                    frame False {
                      n182 = local write "Estagio auto"(2 ("Estagio auto")) -> ()
                    }
                    frame True {
                      w396 = TRUE ("Boolean")
                      n183 = local write "Estagio auto"(2 ("Estagio auto")) -> ()
                      n184 = local write "Vácuo 2"(w396) -> ()
                      n185 = call "Controle_vacuo.vi"("time (s) to wait vacuo"=u32 5, "Boolean"=w396) -> ("Vacuo"=w397:bool)  [unwired: 9 in]
                      n186 = local write "Vácuo 2"(w397) -> ()
                      n187 = local write "String"("Limpar volume referencia" ("String")) -> ()
                    }
                  }
                }
                frame 2 {
                  n188 = property on="Contador" class="DigNum (strict)"() -> ("Value"=w410:i32)  [unwired: 2 in, 2 out]
                  n189 = local write "String"("Ler ZPit" ("String")) -> ()
                  n190 = Increment(x=w410) -> (x+1=w409:i32)
                  n191 = property on="N fit 2" class="DigNum (strict)"() -> ("Value"=w407:i32)  [unwired: 2 in, 2 out]
                  n192 = Equal?(x=w409, y=w407) -> (x = y?=w408:bool)
                  n193 = case shown="True" w408 {
                    frame False {
                    }
                    frame True {
                      n194 = local write "Estagio auto"(3 ("Estagio auto")) -> ()
                    }
                  }
                }
                frame 3 {
                  w418 = "\t"
                  n195 = property on="SET" class="DigNum (strict)"() -> ("Value"=w414:i32)  [unwired: 2 in, 2 out]
                  n196 = property on="Read ZPit" class="Bool (strict)"() -> ("Value"=w413:bool)  [unwired: 2 in, 2 out]
                  n197 = case shown="False" w413 {
                    tunnel: ["  ==>" w425] -> w419
                    frame False {
                    }
                    frame True {
                      n198 = property on="P fit" class="DigNum (strict)"() -> ("Value"=w424:dbl)  [unwired: 2 in, 2 out]
                      n199 = Number To Fractional String(number=w424, precision (6)=i16 3) -> (F-format string=w425:string)  [unwired: 2 in]
                    }
                  }
                  n200 = Number To Decimal String(number=w414) -> (decimal integer string=w417:string)  [unwired: 1 in]
                  n201 = Concatenate Strings(w417, w418, w419, w418) -> (w416:string)
                  n202 = flat-sequence {
                    tunnel: [w429] -> w421
                    tunnel: [w428] -> w420
                    tunnel: w416 -> [w427]
                    tunnel: w415 -> [w426]
                    tunnel: w421 -> [w445]
                    tunnel: w420 -> [w444]
                    frame #0 {
                      n203 = Open/Create/Replace File(file path (use dialog)=w426, operation (0:open)=T3."open") -> (refnum out=w435:refnum<file>, error out=w436:errorcluster)  [unwired: 2 in, 3 out]
                      n204 = Set File Position(refnum=w435, from (0:start)=enum16{"start", "end", "current"}."end", error in=w436) -> (refnum out=w433:refnum<file>, error out=w432:errorcluster)  [unwired: 1 in]
                      n205 = Write to Text File(file (use dialog)=w433, text=w427, error in=w432) -> (refnum out=w437:refnum<file>, error out=w438:errorcluster)  [unwired: 2 out]
                      n206 = Close File(refnum=w437, error in=w438) -> (path=w429:path, error out=w430:errorcluster)
                      n207 = call <vilib>:"Simple Error Handler.vi"("error in (no error)"=w430) -> ("error out"=w428:errorcluster)  [unwired: 1 in, 7 out]
                    }
                    frame #1 {
                      w439 = 0 ("limpo")
                      n208 = local write "Estagio auto"(4 ("Estagio auto")) -> ()
                      n209 = local write "ZPit 2"(TRUE ("ZPit")) -> ()
                      n210 = Wait (ms)(milliseconds to wait=u32 500) -> ()  [unwired: 1 out]
                      n211 = local write "limpo"(w439) -> ()
                      n212 = Read from Text File(file (use dialog)=w445, count=-1 ("Count  3"), error in=w444) -> (refnum out=w446:refnum<file>, text=w450:string, error out=w447:errorcluster)  [unwired: 1 in, 1 out]
                      n213 = local write "String 3"(w450) -> ()
                      n214 = local write "estagio 5"(w439) -> ()
                      n215 = Close File(refnum=w446, error in=w447) -> (error out=w448:errorcluster)  [unwired: 1 out]
                      n216 = call <vilib>:"Simple Error Handler.vi"("error in (no error)"=w448) -> ()  [unwired: 1 in, 8 out]
                      n217 = local write "String"("abrir valvula entrada gas" ("String")) -> ()
                    }
                    frame #2 {
                      w451 = T7 3 items=["no dialog", "OK message", "continue or stop message", "OK message + warnings", "continue/stop + warnings"] ("type of dialog (OK msg:1)")
                      w457 = TRUE ("Boolean 4")
                      n218 = local write "Entrada gás 2"(w457) -> ()
                      n219 = call-poly <vilib>:"DAQmx Create Virtual Channel.vi"("lines"=tag "Dev1/port0/line1") -> ("task out"=w459:refnum<k21>, "error out"=w460:errorcluster)  [unwired: 13 in]
                      n220 = call <vilib>:"DAQmx Start Task.vi"("task/channels in"=w459, "error in"=w460) -> ("task out"=w461:refnum<k21>, "error out"=w462:errorcluster)  [unwired: 12 in]
                      n221 = call-poly <vilib>:"DAQmx Write.vi"("task/channels in"=w461, "data"=w457, "error in"=w462) -> ("task out"=w454:refnum<k21>, "error out"=w453:errorcluster)  [unwired: 10 in, 1 out]
                      n222 = call <vilib>:"DAQmx Stop Task.vi"("task/channels in"=w454, "error in"=w453) -> ("task out"=w455:refnum<k21>, "error out"=w456:errorcluster)  [unwired: 12 in]
                      n223 = call <vilib>:"DAQmx Clear Task.vi"("task in"=w455, "error in"=w456) -> ("error out"=w452:errorcluster)  [unwired: 13 in]
                      n224 = call <vilib>:"Simple Error Handler.vi"("type of dialog (OK msg:1)"=w451, "error in (no error)"=w452) -> ()  [unwired: 3 in, 5 out]
                    }
                  }
                }
                frame 4 {
                  n225 = Greater Or Equal?(x=w464, y="Set P auto") -> (x >= y?=w465:bool)
                  n226 = case shown="True" w465 {
                    tunnel: "Set P auto" -> [_ w480]
                    frame False {
                      w473 = T7 3 items=["no dialog", "OK message", "continue or stop message", "OK message + warnings", "continue/stop + warnings"] ("type of dialog (OK msg:1)")
                      w479 = TRUE ("data")
                      n227 = local write "Estagio auto"(5 ("Estagio auto")) -> ()
                      n228 = Wait (ms)(milliseconds to wait=u32 500) -> ()  [unwired: 1 out]
                      n229 = local write "Entrada gás 2"(w479) -> ()
                      n230 = call-poly <vilib>:"DAQmx Create Virtual Channel.vi"("lines"=tag "Dev1/port0/line1") -> ("task out"=w470:refnum<k21>, "error out"=w469:errorcluster)  [unwired: 13 in]
                      n231 = call <vilib>:"DAQmx Start Task.vi"("task/channels in"=w470, "error in"=w469) -> ("task out"=w468:refnum<k21>, "error out"=w467:errorcluster)  [unwired: 12 in]
                      n232 = call-poly <vilib>:"DAQmx Write.vi"("task/channels in"=w468, "data"=w479, "error in"=w467) -> ("task out"=w476:refnum<k21>, "error out"=w475:errorcluster)  [unwired: 10 in, 1 out]
                      n233 = call <vilib>:"DAQmx Stop Task.vi"("task/channels in"=w476, "error in"=w475) -> ("task out"=w478:refnum<k21>, "error out"=w477:errorcluster)  [unwired: 12 in]
                      n234 = call <vilib>:"DAQmx Clear Task.vi"("task in"=w478, "error in"=w477) -> ("error out"=w474:errorcluster)  [unwired: 13 in]
                      n235 = call <vilib>:"Simple Error Handler.vi"("type of dialog (OK msg:1)"=w473, "error in (no error)"=w474) -> ()  [unwired: 3 in, 5 out]
                    }
                    frame True {
                      n236 = flat-sequence {
                        tunnel: [w483] -> w481
                        tunnel: w480 -> [w483]
                        tunnel: [w498] -> w482
                        tunnel: w481 -> [w497]
                        tunnel: w482 -> [w512]
                        frame #0 {
                          w489 = T7 3 items=["no dialog", "OK message", "continue or stop message", "OK message + warnings", "continue/stop + warnings"] ("type of dialog (OK msg:1)")
                          w496 = FALSE ("data")
                          n237 = Wait (ms)(milliseconds to wait=u32 500) -> ()  [unwired: 1 out]
                          n238 = local write "Entrada gás 2"(w496) -> ()
                          n239 = call-poly <vilib>:"DAQmx Create Virtual Channel.vi"("lines"=tag "Dev1/port0/line1") -> ("task out"=w487:refnum<k21>, "error out"=w488:errorcluster)  [unwired: 13 in]
                          n240 = call <vilib>:"DAQmx Start Task.vi"("task/channels in"=w487, "error in"=w488) -> ("task out"=w485:refnum<k21>, "error out"=w484:errorcluster)  [unwired: 12 in]
                          n241 = call-poly <vilib>:"DAQmx Write.vi"("task/channels in"=w485, "data"=w496, "error in"=w484) -> ("task out"=w493:refnum<k21>, "error out"=w492:errorcluster)  [unwired: 10 in, 1 out]
                          n242 = call <vilib>:"DAQmx Stop Task.vi"("task/channels in"=w493, "error in"=w492) -> ("task out"=w495:refnum<k21>, "error out"=w494:errorcluster)  [unwired: 12 in]
                          n243 = call <vilib>:"DAQmx Clear Task.vi"("task in"=w495, "error in"=w494) -> ("error out"=w490:errorcluster)  [unwired: 13 in]
                          n244 = call <vilib>:"Simple Error Handler.vi"("type of dialog (OK msg:1)"=w489, "error in (no error)"=w490) -> ()  [unwired: 3 in, 5 out]
                        }
                        frame #1 {
                          n245 = stacked-sequence {
                            tunnel: [_ _ _ w509] -> w498
                            tunnel: w497 -> [_ _ w502 _]
                            frame #0 {
                              n246 = call "Controle_ATM.vi"("seconds to wait"=2.0) -> ("Atm"=w500:bool)  [unwired: 9 in, 1 out]
                              n247 = local write "Atm 2"(w500) -> ()
                            }
                            frame #1 {
                              n248 = Wait (ms)(milliseconds to wait=u32 1000) -> ()  [unwired: 1 out]
                            }
                            frame #2 {
                              n249 = Less Or Equal?(x=w502, y=1.5) -> (x <= y?=w504:bool)
                              n250 = case shown="True" w504 {
                                frame False {
                                n251 = call "Controle_ATM.vi"("seconds to wait"=2.0) -> ()  [unwired: 9 in, 2 out]
                                }
                                frame True {
                                w507 = TRUE ("Vácuo")
                                n252 = local write "Vácuo 2"(w507) -> ()
                                n253 = call "Controle_vacuo.vi"("time (s) to wait vacuo"=3.0, "Boolean"=w507) -> ("Vacuo"=w508:bool)  [unwired: 9 in]
                                n254 = local write "Vácuo 2"(w508) -> ()
                                }
                              }
                            }
                            frame #3 {
                              n255 = property on="limpo" class="DigNum (strict)"() -> ("Value"=w510:i32)  [unwired: 2 in, 2 out]
                              n256 = Wait (ms)(milliseconds to wait=u32 1000) -> ()  [unwired: 1 out]
                              n257 = Increment(x=w510) -> (x+1=w509:i32)
                            }
                          }
                        }
                        frame #2 {
                          "limpo" <- w512
                        }
                      }
                    }
                  }
                }
                frame 5 {
                  n258 = property on="Set P auto" class="DigNum (strict)"() -> ("Value"=w514:dbl)  [unwired: 2 in, 2 out]
                  n259 = Greater Or Equal?(x=w515, y=w514) -> (x >= y?=w513:bool)
                  n260 = case shown="True" w513 {
                    selector: w513 -> [_ w537]
                    frame False {
                      n261 = flat-sequence {
                        tunnel: [w517] -> w516
                        tunnel: w516 -> [w533]
                        frame #0 {
                          w520 = T7 3 items=["no dialog", "OK message", "continue or stop message", "OK message + warnings", "continue/stop + warnings"] ("type of dialog (OK msg:1)")
                          w530 = TRUE ("Boolean 4")
                          n262 = property on="estagio 5" class="DigNum (strict)"() -> ("Value"=w518:i32)  [unwired: 2 in, 2 out]
                          n263 = local write "Entrada gás 2"(w530) -> ()
                          n264 = Increment(x=w518) -> (x+1=w517:i32)
                          n265 = call-poly <vilib>:"DAQmx Create Virtual Channel.vi"("lines"=tag "Dev1/port0/line1") -> ("task out"=w524:refnum<k21>, "error out"=w523:errorcluster)  [unwired: 13 in]
                          n266 = call <vilib>:"DAQmx Start Task.vi"("task/channels in"=w524, "error in"=w523) -> ("task out"=w522:refnum<k21>, "error out"=w521:errorcluster)  [unwired: 12 in]
                          n267 = call-poly <vilib>:"DAQmx Write.vi"("task/channels in"=w522, "data"=w530, "error in"=w521) -> ("task out"=w527:refnum<k21>, "error out"=w526:errorcluster)  [unwired: 10 in, 1 out]
                          n268 = call <vilib>:"DAQmx Stop Task.vi"("task/channels in"=w527, "error in"=w526) -> ("task out"=w528:refnum<k21>, "error out"=w529:errorcluster)  [unwired: 12 in]
                          n269 = call <vilib>:"DAQmx Clear Task.vi"("task in"=w528, "error in"=w529) -> ("error out"=w519:errorcluster)  [unwired: 13 in]
                          n270 = call <vilib>:"Simple Error Handler.vi"("type of dialog (OK msg:1)"=w520, "error in (no error)"=w519) -> ()  [unwired: 3 in, 5 out]
                        }
                        frame #1 {
                          n271 = Less?(x=w533, y=6) -> (x < y?=w531:bool)
                          n272 = case shown="False" w531 {
                            frame False {
                              n273 = local write "Estagio auto"(5 ("Estagio auto")) -> ()
                            }
                            frame True {
                              n274 = local write "Estagio auto"(4 ("Estagio auto")) -> ()
                            }
                          }
                          "estagio 5" <- w533
                        }
                      }
                    }
                    frame True {
                      n275 = flat-sequence {
                        tunnel: w537 -> [w538]
                        tunnel: [w538] -> w536
                        tunnel: w536 -> [w554]
                        frame #0 {
                          w539 = FALSE ("Boolean 4")
                          w544 = T7 3 items=["no dialog", "OK message", "continue or stop message", "OK message + warnings", "continue/stop + warnings"] ("type of dialog (OK msg:1)")
                          n276 = local write "Entrada gás 2"(w539) -> ()
                          n277 = call-poly <vilib>:"DAQmx Create Virtual Channel.vi"("lines"=tag "Dev1/port0/line1") -> ("task out"=w542:refnum<k21>, "error out"=w543:errorcluster)  [unwired: 13 in]
                          n278 = call <vilib>:"DAQmx Start Task.vi"("task/channels in"=w542, "error in"=w543) -> ("task out"=w545:refnum<k21>, "error out"=w546:errorcluster)  [unwired: 12 in]
                          n279 = call-poly <vilib>:"DAQmx Write.vi"("task/channels in"=w545, "data"=w539, "error in"=w546) -> ("task out"=w550:refnum<k21>, "error out"=w547:errorcluster)  [unwired: 10 in, 1 out]
                          n280 = call <vilib>:"DAQmx Stop Task.vi"("task/channels in"=w550, "error in"=w547) -> ("task out"=w549:refnum<k21>, "error out"=w548:errorcluster)  [unwired: 12 in]
                          n281 = call <vilib>:"DAQmx Clear Task.vi"("task in"=w549, "error in"=w548) -> ("error out"=w541:errorcluster)  [unwired: 13 in]
                          n282 = call <vilib>:"Simple Error Handler.vi"("type of dialog (OK msg:1)"=w544, "error in (no error)"=w541) -> ()  [unwired: 3 in, 5 out]
                        }
                        frame #1 {
                          n283 = property on="estagio 5" class="DigNum (strict)"() -> ("Value"=w552:i32)  [unwired: 2 in, 2 out]
                          n284 = Greater?(x=w552, y=5) -> (0:w555:bool)
                          n285 = And(x=w554, y=w555) -> (x .and. y?=w553:bool)
                          n286 = case shown="True" w553 {
                            frame False {
                              n287 = local write "Estagio auto"(4 ("Estagio auto")) -> ()
                              n288 = Wait (ms)(milliseconds to wait=u32 500) -> ()  [unwired: 1 out]
                            }
                            frame True {
                              n289 = property on="Contador" class="DigNum (strict)"() -> ("Value"=w559:i32)  [unwired: 2 in, 2 out]
                              n290 = local write "String"("Ler Pit" ("String")) -> ()
                              n291 = Increment(x=w559) -> (x+1=w561:i32)
                              n292 = property on="N fit 2" class="DigNum (strict)"() -> ("Value"=w558:i32)  [unwired: 2 in, 2 out]
                              n293 = Equal?(x=w561, y=w558) -> (x = y?=w560:bool)
                              n294 = case shown="True" w560 {
                                frame False {
                                }
                                frame True {
                                n295 = local write "Estagio auto"(6 ("Estagio auto")) -> ()
                                }
                              }
                            }
                          }
                        }
                      }
                    }
                  }
                }
                frame 6 {
                  n296 = property on="Contador" class="DigNum (strict)"() -> ("Value"=w565:i32)  [unwired: 2 in, 2 out]
                  n297 = Increment(x=w565) -> (x+1=w567:i32)
                  n298 = property on="N fit 2" class="DigNum (strict)"() -> ("Value"=w564:i32)  [unwired: 2 in, 2 out]
                  n299 = Equal?(x=w567, y=w564) -> (x = y?=w566:bool)
                  n300 = case shown="True" w566 {
                    tunnel: w568 -> [_ w569]
                    frame False {
                    }
                    frame True {
                      n301 = property on="P fit" class="DigNum (strict)"() -> ("Value"=w570:dbl)  [unwired: 2 in, 2 out]
                      n302 = Number To Fractional String(number=w570, precision (6)=i16 3) -> (F-format string=w574:string)  [unwired: 2 in]
                      n303 = Concatenate Strings(w574, "\t") -> (w572:string)
                      n304 = flat-sequence {
                        tunnel: [w580] -> w576
                        tunnel: [w579] -> w575
                        tunnel: w572 -> [w578]
                        tunnel: w569 -> [w577]
                        tunnel: w576 -> [w596]
                        tunnel: w575 -> [w595]
                        frame #0 {
                          n305 = Open/Create/Replace File(file path (use dialog)=w577, operation (0:open)=T3."open") -> (refnum out=w586:refnum<file>, error out=w587:errorcluster)  [unwired: 2 in, 3 out]
                          n306 = Set File Position(refnum=w586, from (0:start)=enum16{"start", "end", "current"}."end", error in=w587) -> (refnum out=w584:refnum<file>, error out=w583:errorcluster)  [unwired: 1 in]
                          n307 = Write to Text File(file (use dialog)=w584, text=w578, error in=w583) -> (refnum out=w588:refnum<file>, error out=w589:errorcluster)  [unwired: 2 out]
                          n308 = Close File(refnum=w588, error in=w589) -> (path=w580:path, error out=w581:errorcluster)
                          n309 = call <vilib>:"Simple Error Handler.vi"("error in (no error)"=w581) -> ("error out"=w579:errorcluster)  [unwired: 1 in, 7 out]
                        }
                        frame #1 {
                          n310 = local write "Estagio auto"(7 ("Estagio auto")) -> ()
                          n311 = local write "teste slope"(0 ("teste slope")) -> ()
                          n312 = local write "Pit 2"(TRUE ("ZPit")) -> ()
                          n313 = Wait (ms)(milliseconds to wait=u32 500) -> ()  [unwired: 1 out]
                          n314 = Read from Text File(file (use dialog)=w596, count=-1 ("Count  3"), error in=w595) -> (refnum out=w597:refnum<file>, text=w601:string, error out=w598:errorcluster)  [unwired: 1 in, 1 out]
                          n315 = local write "String 3"(w601) -> ()
                          n316 = Close File(refnum=w597, error in=w598) -> (error out=w599:errorcluster)  [unwired: 1 out]
                          n317 = call <vilib>:"Simple Error Handler.vi"("error in (no error)"=w599) -> ()  [unwired: 1 in, 8 out]
                          n318 = local write "String"("abrir valvula entrada camara" ("String")) -> ()
                        }
                      }
                    }
                  }
                }
                frame 7 {
                  n319 = flat-sequence {
                    tunnel: w608 -> [w612]
                    tunnel: w609 -> [w613]
                    tunnel: w610 -> [w614]
                    tunnel: [w614] -> w607
                    tunnel: [w613] -> w605
                    tunnel: [w612] -> w603
                    tunnel: w607 -> [w617]
                    tunnel: [w617] -> w606
                    tunnel: w605 -> [w615]
                    tunnel: [w615] -> w604
                    tunnel: w603 -> [w616]
                    tunnel: [w616] -> w602
                    tunnel: w606 -> [_]
                    tunnel: w604 -> [_]
                    tunnel: w602 -> [_]
                    frame #0 {
                      n320 = local write "N fit"("N fit patamar") -> ()
                    }
                    frame #1 {
                      n321 = flat-sequence {
                        tunnel: w617 -> [w631]
                        tunnel: w615 -> [w630]
                        tunnel: w616 -> [w629]
                        frame #0 {
                          w624 = i16 6 ("precision (6)")
                          w620 = "\t"
                          w648 = i16 4 ("precision (6)")
                          n322 = call "Advanced Serial.vi"() -> ("V-P01(mV)"=w623:dbl, "P01 (Bar)"=w628:dbl, "P02 (Bar)"=w625:dbl, "V-P02(mV)"=w622:dbl)  [unwired: 7 in, 5 out]
                          n323 = Number To Fractional String(number=w625, precision (6)=w624) -> (F-format string=w626:string)  [unwired: 2 in]
                          n324 = Number To Fractional String(number=w628, precision (6)=w624) -> (F-format string=w627:string)  [unwired: 2 in]
                          n325 = Number To Fractional String(number=w630, precision (6)=w648) -> (F-format string=w643:string)  [unwired: 2 in]
                          n326 = Number To Fractional String(number=w629, precision (6)=w648) -> (F-format string=w642:string)  [unwired: 2 in]
                          n327 = Open/Create/Replace File(file path (use dialog)=w631, operation (0:open)=T3."open") -> (refnum out=w639:refnum<file>, error out=w632:errorcluster)  [unwired: 2 in, 3 out]
                          n328 = Get Date/Time String(date format (0)=enum16{"short", "long", "abbreviated"}."short", want seconds? (F)=TRUE) -> (date string=w645:string, time string=w644:string)  [unwired: 1 in]
                          n329 = Number To Fractional String(number=w622, precision (6)=w624) -> (F-format string=w619:string)  [unwired: 2 in]
                          n330 = Number To Fractional String(number=w623, precision (6)=w624) -> (F-format string=w621:string)  [unwired: 2 in]
                          n331 = Set File Position(refnum=w639, from (0:start)=enum16{"start", "end", "current"}."end", error in=w632) -> (refnum out=w637:refnum<file>, error out=w636:errorcluster)  [unwired: 1 in]
                          n332 = Concatenate Strings(w645, w620, w644, w620, w643, w620, w642, w620, w620, w627, w620, w626, w620, w621, w620, w619, "\r\n") -> (w633:string)
                          n333 = Write to Text File(file (use dialog)=w637, text=w633, error in=w636) -> (refnum out=w640:refnum<file>, error out=w641:errorcluster)  [unwired: 2 out]
                          n334 = Close File(refnum=w640, error in=w641) -> (error out=w634:errorcluster)  [unwired: 1 out]
                          n335 = call <vilib>:"Simple Error Handler.vi"("error in (no error)"=w634) -> ()  [unwired: 1 in, 8 out]
                        }
                      }
                    }
                    frame #2 {
                      n336 = property on="Contador" class="DigNum (strict)"() -> ("Value"=w657:i32)  [unwired: 2 in, 2 out]
                      n337 = Increment(x=w657) -> (x+1=w656:i32)
                      n338 = property on="N fit patamar" class="DigNum (strict)"() -> ("Value"=w649:i32)  [unwired: 2 in, 2 out]
                      n339 = Equal?(x=w656, y=w649) -> (x = y?=w658:bool)
                      n340 = case shown="True" w658 {
                        tunnel: [FALSE w663] -> w655
                        tunnel: [_ w662] -> w654
                        frame False {
                        }
                        frame True {
                          n341 = property on="P (bar/s)" class="DigNum (strict)"() -> ("Value"=w665:dbl)  [unwired: 2 in, 2 out]
                          n342 = Absolute Value(x=w665) -> (abs(x)=w664:dbl)
                          n343 = Less Or Equal?(x=w664, y="STOP (bar/s)") -> (x <= y?=w663:bool)
                          n344 = case shown="True" w663 {
                            tunnel: [_ w667] -> w662
                            frame False {
                            }
                            frame True {
                              n345 = property on="teste slope" class="DigNum (strict)"() -> ("Value"=w668:i32)  [unwired: 2 in, 2 out]
                              n346 = local write "Estagio auto"(7 ("Estagio auto")) -> ()
                              n347 = Increment(x=w668) -> (x+1=w667:i32)
                              "teste slope" <- w667
                            }
                          }
                        }
                      }
                      n348 = Greater Or Equal?(x=w654, y="Ntest") -> (x >= y?=w652:bool)
                      n349 = And(x=w658, y=w652) -> (x .and. y?=w651:bool)
                      n350 = case shown="True" w651 {
                        tunnel: [TRUE ("Boolean") FALSE ("Boolean")] -> w650
                        frame False {
                        }
                        frame True {
                        }
                      }
                      n351 = case shown="True" w651 {
                        frame False {
                        }
                        frame True {
                          n352 = flat-sequence {
                            frame #0 {
                              n353 = property on="N fit 2" class="DigNum (strict)"() -> ("Value"=w787:i32)  [unwired: 2 in, 2 out]
                              n354 = Wait (ms)(milliseconds to wait=u32 500) -> ()  [unwired: 1 out]
                              n355 = local write "N fit"(w787) -> ()
                            }
                            frame #1 {
                              n356 = local write "Estagio auto"(8 ("Estagio auto")) -> ()
                            }
                          }
                        }
                      }
                      n357 = case shown="True" w655 {
                        tunnel: w650 -> [_ w728]
                        frame False {
                          w682 = T7 3 items=["no dialog", "OK message", "continue or stop message", "OK message + warnings", "continue/stop + warnings"] ("type of dialog (OK msg:1)")
                          w670 = TRUE ("Boolean")
                          n358 = call-poly <vilib>:"DAQmx Create Virtual Channel.vi"("lines"=tag "Dev1/port0/line3") -> ("task out"=w672:refnum<k21>, "error out"=w673:errorcluster)  [unwired: 13 in]
                          n359 = Wait (ms)(milliseconds to wait="patamar milliseconds to wait") -> ()  [unwired: 1 out]
                          n360 = local write "Câmara 2"(w670) -> ()
                          n361 = call <vilib>:"DAQmx Start Task.vi"("task/channels in"=w672, "error in"=w673) -> ("task out"=w674:refnum<k21>, "error out"=w675:errorcluster)  [unwired: 12 in]
                          n362 = call-poly <vilib>:"DAQmx Write.vi"("task/channels in"=w674, "data"=w670, "error in"=w675) -> ("task out"=w679:refnum<k21>, "error out"=w680:errorcluster)  [unwired: 10 in, 1 out]
                          n363 = case shown="True" w670 {
                            frame False {
                            }
                            frame True {
                              n364 = property on="Vol Ref 3" class="Slide (strict)"() -> ("Value"=w725:dbl)  [unwired: 2 in, 2 out]
                              n365 = local write "Camara 2"(w725) -> ()
                            }
                          }
                          n366 = call <vilib>:"DAQmx Stop Task.vi"("task/channels in"=w679, "error in"=w680) -> ("task out"=w677:refnum<k21>, "error out"=w676:errorcluster)  [unwired: 12 in]
                          n367 = call <vilib>:"DAQmx Clear Task.vi"("task in"=w677, "error in"=w676) -> ("error out"=w681:errorcluster)  [unwired: 13 in]
                          n368 = call <vilib>:"Simple Error Handler.vi"("type of dialog (OK msg:1)"=w682, "error in (no error)"=w681) -> ()  [unwired: 3 in, 5 out]
                          n369 = case shown="True" w670 {
                            tunnel: [w687 w704] -> _
                            frame False {
                              n370 = flat-sequence {
                                tunnel: [w688] -> w686
                                tunnel: w686 -> [w693]
                                tunnel: [w693] -> w685
                                tunnel: w685 -> [w695]
                                tunnel: [w695] -> w684
                                tunnel: w684 -> [w699]
                                tunnel: [w699] -> w683
                                tunnel: [w700] -> w687
                                tunnel: w683 -> [w700]
                                frame #0 {
                                w688 = 0.0 ("number")
                                n371 = call "data2byte.vi"("argument"=w688, "new function"=4.0) -> ("protocol"=w689:string)  [unwired: 8 in, 1 out]
                                n372 = call "Advanced Serial.vi"("string to write"=w689, "Write"=TRUE ("write")) -> ()  [unwired: 5 in, 9 out]
                                }
                                frame #1 {
                                n373 = Wait Until Next ms Multiple(millisecond multiple=u32 20) -> ()  [unwired: 1 out]
                                }
                                frame #2 {
                                n374 = call "data2byte.vi"("argument"=w695, "new function"=1.0) -> ("protocol"=w697:string)  [unwired: 8 in, 1 out]
                                n375 = call "Advanced Serial.vi"("string to write"=w697, "Write"=TRUE ("write")) -> ()  [unwired: 5 in, 9 out]
                                }
                                frame #3 {
                                n376 = Wait Until Next ms Multiple(millisecond multiple=u32 20) -> ()  [unwired: 1 out]
                                }
                                frame #4 {
                                n377 = call "data2byte.vi"("argument"=w700, "new function"=2.0) -> ("protocol"=w702:string)  [unwired: 8 in, 1 out]
                                n378 = call "Advanced Serial.vi"("string to write"=w702, "Write"=TRUE ("write")) -> ()  [unwired: 5 in, 9 out]
                                }
                              }
                            }
                            frame True {
                              n379 = flat-sequence {
                                tunnel: [w709] -> w708
                                tunnel: w708 -> [w714]
                                tunnel: [w714] -> w707
                                tunnel: w707 -> [w716]
                                tunnel: [w716] -> w706
                                tunnel: w706 -> [w720]
                                tunnel: [w720] -> w705
                                tunnel: w705 -> [w721]
                                tunnel: [w721] -> w704
                                frame #0 {
                                w709 = 1.0 ("number")
                                n380 = call "data2byte.vi"("argument"=w709, "new function"=4.0) -> ("protocol"=w710:string)  [unwired: 8 in, 1 out]
                                n381 = call "Advanced Serial.vi"("string to write"=w710, "Write"=TRUE ("write")) -> ()  [unwired: 5 in, 9 out]
                                }
                                frame #1 {
                                n382 = Wait Until Next ms Multiple(millisecond multiple=u32 20) -> ()  [unwired: 1 out]
                                }
                                frame #2 {
                                n383 = call "data2byte.vi"("argument"=w716, "new function"=1.0) -> ("protocol"=w718:string)  [unwired: 8 in, 1 out]
                                n384 = call "Advanced Serial.vi"("string to write"=w718, "Write"=TRUE ("write")) -> ()  [unwired: 5 in, 9 out]
                                }
                                frame #3 {
                                n385 = Wait Until Next ms Multiple(millisecond multiple=u32 20) -> ()  [unwired: 1 out]
                                }
                                frame #4 {
                                n386 = call "data2byte.vi"("argument"=w721, "new function"=2.0) -> ("protocol"=w723:string)  [unwired: 8 in, 1 out]
                                n387 = call "Advanced Serial.vi"("string to write"=w723, "Write"=TRUE ("write")) -> ()  [unwired: 5 in, 9 out]
                                }
                              }
                            }
                          }
                        }
                        frame True {
                          n388 = flat-sequence {
                            tunnel: w728 -> [w729]
                            tunnel: [w729] -> w726
                            tunnel: [w773] -> w727
                            tunnel: w726 -> [w773]
                            tunnel: w727 -> [w774]
                            frame #0 {
                              n389 = case shown="True" w729 {
                                tunnel: [w734 w751] -> _
                                frame False {
                                n390 = flat-sequence {
                                tunnel: [w735] -> w733
                                tunnel: w733 -> [w740]
                                tunnel: [w740] -> w732
                                tunnel: w732 -> [w742]
                                tunnel: [w742] -> w731
                                tunnel: w731 -> [w746]
                                tunnel: [w746] -> w730
                                tunnel: [w747] -> w734
                                tunnel: w730 -> [w747]
                                frame #0 {
                                w735 = 0.0 ("number")
                                n391 = call "data2byte.vi"("argument"=w735, "new function"=4.0) -> ("protocol"=w736:string)  [unwired: 8 in, 1 out]
                                n392 = call "Advanced Serial.vi"("string to write"=w736, "Write"=TRUE ("write")) -> ()  [unwired: 5 in, 9 out]
                                }
                                frame #1 {
                                n393 = Wait Until Next ms Multiple(millisecond multiple=u32 20) -> ()  [unwired: 1 out]
                                }
                                frame #2 {
                                n394 = call "data2byte.vi"("argument"=w742, "new function"=1.0) -> ("protocol"=w744:string)  [unwired: 8 in, 1 out]
                                n395 = call "Advanced Serial.vi"("string to write"=w744, "Write"=TRUE ("write")) -> ()  [unwired: 5 in, 9 out]
                                }
                                frame #3 {
                                n396 = Wait Until Next ms Multiple(millisecond multiple=u32 20) -> ()  [unwired: 1 out]
                                }
                                frame #4 {
                                n397 = call "data2byte.vi"("argument"=w747, "new function"=2.0) -> ("protocol"=w749:string)  [unwired: 8 in, 1 out]
                                n398 = call "Advanced Serial.vi"("string to write"=w749, "Write"=TRUE ("write")) -> ()  [unwired: 5 in, 9 out]
                                }
                                }
                                }
                                frame True {
                                n399 = flat-sequence {
                                tunnel: [w756] -> w755
                                tunnel: w755 -> [w761]
                                tunnel: [w761] -> w754
                                tunnel: w754 -> [w763]
                                tunnel: [w763] -> w753
                                tunnel: w753 -> [w767]
                                tunnel: [w767] -> w752
                                tunnel: w752 -> [w768]
                                tunnel: [w768] -> w751
                                frame #0 {
                                w756 = 1.0 ("number")
                                n400 = call "data2byte.vi"("argument"=w756, "new function"=4.0) -> ("protocol"=w757:string)  [unwired: 8 in, 1 out]
                                n401 = call "Advanced Serial.vi"("string to write"=w757, "Write"=TRUE ("write")) -> ()  [unwired: 5 in, 9 out]
                                }
                                frame #1 {
                                n402 = Wait Until Next ms Multiple(millisecond multiple=u32 20) -> ()  [unwired: 1 out]
                                }
                                frame #2 {
                                n403 = call "data2byte.vi"("argument"=w763, "new function"=1.0) -> ("protocol"=w765:string)  [unwired: 8 in, 1 out]
                                n404 = call "Advanced Serial.vi"("string to write"=w765, "Write"=TRUE ("write")) -> ()  [unwired: 5 in, 9 out]
                                }
                                frame #3 {
                                n405 = Wait Until Next ms Multiple(millisecond multiple=u32 20) -> ()  [unwired: 1 out]
                                }
                                frame #4 {
                                n406 = call "data2byte.vi"("argument"=w768, "new function"=2.0) -> ("protocol"=w770:string)  [unwired: 8 in, 1 out]
                                n407 = call "Advanced Serial.vi"("string to write"=w770, "Write"=TRUE ("write")) -> ()  [unwired: 5 in, 9 out]
                                }
                                }
                                }
                              }
                            }
                            frame #1 {
                              n408 = Wait Until Next ms Multiple(millisecond multiple=u32 20) -> ()  [unwired: 1 out]
                            }
                            frame #2 {
                              w776 = T7 3 items=["no dialog", "OK message", "continue or stop message", "OK message + warnings", "continue/stop + warnings"] ("type of dialog (OK msg:1)")
                              n409 = local write "Câmara 2"(w774) -> ()
                              n410 = call-poly <vilib>:"DAQmx Create Virtual Channel.vi"("lines"=tag "Dev1/port0/line3") -> ("task out"=w785:refnum<k21>, "error out"=w784:errorcluster)  [unwired: 13 in]
                              n411 = call <vilib>:"DAQmx Start Task.vi"("task/channels in"=w785, "error in"=w784) -> ("task out"=w783:refnum<k21>, "error out"=w782:errorcluster)  [unwired: 12 in]
                              n412 = call-poly <vilib>:"DAQmx Write.vi"("task/channels in"=w783, "data"=w774, "error in"=w782) -> ("task out"=w778:refnum<k21>, "error out"=w777:errorcluster)  [unwired: 10 in, 1 out]
                              n413 = call <vilib>:"DAQmx Stop Task.vi"("task/channels in"=w778, "error in"=w777) -> ("task out"=w780:refnum<k21>, "error out"=w781:errorcluster)  [unwired: 12 in]
                              n414 = call <vilib>:"DAQmx Clear Task.vi"("task in"=w780, "error in"=w781) -> ("error out"=w775:errorcluster)  [unwired: 13 in]
                              n415 = call <vilib>:"Simple Error Handler.vi"("type of dialog (OK msg:1)"=w776, "error in (no error)"=w775) -> ()  [unwired: 3 in, 5 out]
                            }
                            frame #3 {
                              n416 = Wait (ms)(milliseconds to wait=u32 2000) -> ()  [unwired: 1 out]
                            }
                          }
                        }
                      }
                    }
                  }
                }
                frame 8 {
                  n417 = property on="Contador" class="DigNum (strict)"() -> ("Value"=w816:i32)  [unwired: 2 in, 2 out]
                  n418 = Increment(x=w816) -> (x+1=w817:i32)
                  n419 = property on="N fit 2" class="DigNum (strict)"() -> ("Value"=w790:i32)  [unwired: 2 in, 2 out]
                  n420 = Equal?(x=w817, y=w790) -> (x = y?=w815:bool)
                  n421 = case shown="False" w814 {
                    tunnel: [FALSE ("Save manual") w1411] -> w794
                    tunnel: w815 -> [_ w1411]
                    frame False {
                    }
                    frame True {
                    }
                  }
                  n422 = case shown="True" w815 {
                    tunnel: w818 -> [_ w1412]
                    frame False {
                    }
                    frame True {
                      n423 = property on="P fit" class="DigNum (strict)"() -> ("Value"=w1413:dbl)  [unwired: 2 in, 2 out]
                      n424 = Number To Fractional String(number=w1413, precision (6)=i16 3) -> (F-format string=w1417:string)  [unwired: 2 in]
                      n425 = Concatenate Strings(w1417, "\t") -> (w1415:string)
                      n426 = flat-sequence {
                        tunnel: [w1424] -> w1419
                        tunnel: [w1423] -> w1418
                        tunnel: w1415 -> [w1422]
                        tunnel: w1412 -> [w1421]
                        tunnel: w1419 -> [w1439]
                        tunnel: w1418 -> [w1438]
                        frame #0 {
                          n427 = Wait (ms)(milliseconds to wait=u32 500) -> ()  [unwired: 1 out]
                          n428 = Open/Create/Replace File(file path (use dialog)=w1421, operation (0:open)=T3."open") -> (refnum out=w1430:refnum<file>, error out=w1431:errorcluster)  [unwired: 2 in, 3 out]
                          n429 = Set File Position(refnum=w1430, from (0:start)=enum16{"start", "end", "current"}."end", error in=w1431) -> (refnum out=w1428:refnum<file>, error out=w1427:errorcluster)  [unwired: 1 in]
                          n430 = Write to Text File(file (use dialog)=w1428, text=w1422, error in=w1427) -> (refnum out=w1432:refnum<file>, error out=w1433:errorcluster)  [unwired: 2 out]
                          n431 = Close File(refnum=w1432, error in=w1433) -> (path=w1424:path, error out=w1425:errorcluster)
                          n432 = call <vilib>:"Simple Error Handler.vi"("error in (no error)"=w1425) -> ("error out"=w1423:errorcluster)  [unwired: 1 in, 7 out]
                        }
                        frame #1 {
                          n433 = local write "Estagio auto"(9 ("Estagio auto")) -> ()
                          n434 = local write "Pf2 2"(TRUE ("ZPit")) -> ()
                          n435 = Wait (ms)(milliseconds to wait=u32 500) -> ()  [unwired: 1 out]
                          n436 = Read from Text File(file (use dialog)=w1439, count=-1 ("Count  3"), error in=w1438) -> (refnum out=w1440:refnum<file>, text=w1444:string, error out=w1441:errorcluster)  [unwired: 1 in, 1 out]
                          n437 = local write "String 3"(w1444) -> ()
                          n438 = Close File(refnum=w1440, error in=w1441) -> (error out=w1442:errorcluster)  [unwired: 1 out]
                          n439 = local write "String"("abrir valvula vacuo" ("String")) -> ()
                          n440 = call <vilib>:"Simple Error Handler.vi"("error in (no error)"=w1442) -> ()  [unwired: 1 in, 8 out]
                        }
                      }
                    }
                  }
                  n441 = flat-sequence {
                    tunnel: w794 -> [w820]
                    tunnel: w797 -> [w821]
                    tunnel: [w821] -> w792
                    tunnel: [w820] -> w791
                    tunnel: [w823] -> w813
                    tunnel: [w825] -> w812
                    tunnel: [w826] -> w811
                    tunnel: [w827] -> w810
                    tunnel: [w828] -> w809
                    tunnel: [w829] -> w808
                    tunnel: [w830] -> w807
                    tunnel: [w831] -> w806
                    tunnel: [w832] -> w805
                    tunnel: [w833] -> w804
                    tunnel: [w834] -> w803
                    tunnel: [w835] -> w802
                    tunnel: [w836] -> w801
                    tunnel: [w837] -> w800
                    tunnel: [w838] -> w799
                    tunnel: [w824] -> w798
                    tunnel: [w822] -> w795
                    tunnel: w792 -> [w840]
                    tunnel: w791 -> [w839]
                    tunnel: w813 -> [w1361]
                    tunnel: w812 -> [w1360]
                    tunnel: w811 -> [w1359]
                    tunnel: w810 -> [w1358]
                    tunnel: w809 -> [w1357]
                    tunnel: w808 -> [w1356]
                    tunnel: w807 -> [w1355]
                    tunnel: w806 -> [w1354]
                    tunnel: w805 -> [w1353]
                    tunnel: w804 -> [w1352]
                    tunnel: w803 -> [w1351]
                    tunnel: w802 -> [w1350]
                    tunnel: w801 -> [w1349]
                    tunnel: w800 -> [w1348]
                    tunnel: w799 -> [w1347]
                    tunnel: w798 -> [w1346]
                    tunnel: [w1344] -> w796
                    tunnel: w795 -> [w1344]
                    tunnel: [TRUE ("graph RLC")] -> w793
                    frame #0 {
                      n442 = local write "graph RLC"(FALSE) -> ()
                    }
                    frame #1 {
                      n443 = case shown="False" w839 {
                        tunnel: [FALSE w877] -> w822
                        tunnel: w840 -> [_ w859]
                        tunnel: [_ w857] -> w823
                        tunnel: [_ w856] -> w824
                        tunnel: [_ w855] -> w825
                        tunnel: [_ w854] -> w826
                        tunnel: [_ w853] -> w827
                        tunnel: [_ w852] -> w828
                        tunnel: [_ w851] -> w829
                        tunnel: [_ w850] -> w830
                        tunnel: [_ w849] -> w831
                        tunnel: [_ w848] -> w832
                        tunnel: [_ w847] -> w833
                        tunnel: [_ w846] -> w834
                        tunnel: [_ w845] -> w835
                        tunnel: [_ w844] -> w836
                        tunnel: [_ w843] -> w837
                        tunnel: [_ w842] -> w838
                        frame False {
                        }
                        frame True {
                          n444 = property on="path RLC_completo" class="Path"() -> ("Value"=w858:path)  [unwired: 2 in, 2 out]
                          n445 = for {
                            N: 5 -> [_]
                            tunnel: TRUE -> [w900]
                            tunnel: FALSE -> [w899]
                            tunnel: [w898] -> w877
                            tunnel: [w897] -> w875 mode=indexing
                            tunnel: [w896] -> w874 mode=indexing
                            tunnel: [w895] -> w873 mode=indexing
                            tunnel: [w894] -> w872 mode=indexing
                            tunnel: [w893] -> w871 mode=indexing
                            tunnel: [w892] -> w870 mode=indexing
                            tunnel: [w891] -> w869 mode=indexing
                            tunnel: [w890] -> w868 mode=indexing
                            tunnel: [w889] -> w867 mode=indexing
                            tunnel: [w888] -> w866 mode=indexing
                            tunnel: [w887] -> w865 mode=indexing
                            tunnel: [w886] -> w864 mode=indexing
                            tunnel: [w885] -> w863 mode=indexing
                            tunnel: [w884] -> w862 mode=indexing
                            tunnel: [w883] -> w861 mode=indexing
                            tunnel: [w882] -> w860 mode=indexing
                            tunnel: w859 -> [w881]
                            tunnel: w858 -> [w880]
                            n446 = stacked-sequence {
                              tunnel: w900 -> [_ w948 w974 w1001 w1026 w1053 w1078 w1105 w1131 w1156 w1182 w1208 w1234 w1260 w1286 w1312 w1339 _]
                              tunnel: w899 -> [w922 _ _ _ _ _ _ _ _ _ _ _ _ _ _ _ _ w1343]
                              tunnel: [_ _ _ _ _ _ _ _ _ _ _ _ _ _ _ _ _ TRUE] -> w898
                              tunnel: [_ w928 _ _ _ _ _ _ _ _ _ _ _ _ _ _ _ _] -> w897
                              tunnel: [_ _ w954 _ _ _ _ _ _ _ _ _ _ _ _ _ _ _] -> w896
                              tunnel: [_ _ _ w980 _ _ _ _ _ _ _ _ _ _ _ _ _ _] -> w895
                              tunnel: [_ _ _ _ w1006 _ _ _ _ _ _ _ _ _ _ _ _ _] -> w894
                              tunnel: [_ _ _ _ _ w1032 _ _ _ _ _ _ _ _ _ _ _ _] -> w893
                              tunnel: [_ _ _ _ _ _ w1058 _ _ _ _ _ _ _ _ _ _ _] -> w892
                              tunnel: [_ _ _ _ _ _ _ w1084 _ _ _ _ _ _ _ _ _ _] -> w891
                              tunnel: [_ _ _ _ _ _ _ _ w1110 _ _ _ _ _ _ _ _ _] -> w890
                              tunnel: [_ _ _ _ _ _ _ _ _ w1136 _ _ _ _ _ _ _ _] -> w889
                              tunnel: [_ _ _ _ _ _ _ _ _ _ w1162 _ _ _ _ _ _ _] -> w888
                              tunnel: [_ _ _ _ _ _ _ _ _ _ _ w1188 _ _ _ _ _ _] -> w887
                              tunnel: [_ _ _ _ _ _ _ _ _ _ _ _ w1214 _ _ _ _ _] -> w886
                              tunnel: [_ _ _ _ _ _ _ _ _ _ _ _ _ w1240 _ _ _ _] -> w885
                              tunnel: [_ _ _ _ _ _ _ _ _ _ _ _ _ _ w1266 _ _ _] -> w884
                              tunnel: [_ _ _ _ _ _ _ _ _ _ _ _ _ _ _ w1292 _ _] -> w883
                              tunnel: [_ _ _ _ _ _ _ _ _ _ _ _ _ _ _ _ w1318 _] -> w882
                              tunnel: w881 -> [_ w927 w953 w979 w1005 w1031 w1057 w1083 w1109 w1135 w1161 w1187 w1213 w1239 w1265 w1291 w1317 _]
                              tunnel: w880 -> [w901 w923 w951 w977 w1003 w1029 w1055 w1081 w1107 w1133 w1159 w1185 w1211 w1237 w1263 w1289 w1315 _]
                              frame #0 {
                                w902 = "\t"
                                n447 = local write "C-50-L"(w922) -> ()
                                n448 = local write "C-50-N"(w922) -> ()
                                n449 = local write "Z-50-L"(w922) -> ()
                                n450 = local write "C-1K-N"(w922) -> ()
                                n451 = local write "C-1K-L"(w922) -> ()
                                n452 = local write "Z-50-N"(w922) -> ()
                                n453 = local write "Z-1K-N"(w922) -> ()
                                n454 = local write "Z-1K-L"(w922) -> ()
                                n455 = local write "C-10K-L"(w922) -> ()
                                n456 = local write "C-100-N"(w922) -> ()
                                n457 = local write "C-10K-N"(w922) -> ()
                                n458 = local write "Z-100-L"(w922) -> ()
                                n459 = local write "Z-10K-L"(w922) -> ()
                                n460 = local write "Z-100-N"(w922) -> ()
                                n461 = local write "Z-10K-N"(w922) -> ()
                                n462 = local write "C-100-L"(w922) -> ()
                                n463 = Open/Create/Replace File(file path (use dialog)=w901, operation (0:open)=T3."open") -> (refnum out=w916:refnum<file>, error out=w915:errorcluster)  [unwired: 2 in, 3 out]
                                n464 = Get Date/Time String(date format (0)=enum16{"short", "long", "abbreviated"}."short", want seconds? (F)=TRUE) -> (date string=w908:string, time string=w907:string)  [unwired: 1 in]
                                n465 = feedback #1() -> (w906:dbl)  [unwired: 1 in]
                                "SET 2" <- w906
                                n466 = Set File Position(refnum=w916, from (0:start)=enum16{"start", "end", "current"}."end", error in=w915) -> (refnum out=w918:refnum<file>, error out=w919:errorcluster)  [unwired: 1 in]
                                n467 = Number To Fractional String(number=w906, precision (6)=i16 2) -> (F-format string=w905:string)  [unwired: 2 in]
                                n468 = Add(x=w906, y=0.2) -> (x+y=w912:dbl)
                                n469 = feedback-in #1(w912) -> ()
                                n470 = Concatenate Strings(w905, w902, w908, w902, w907, w902) -> (w904:string)
                                n471 = Write to Text File(file (use dialog)=w918, text=w904, error in=w919) -> (refnum out=w914:refnum<file>, error out=w913:errorcluster)  [unwired: 1 in, 1 out]
                                n472 = Close File(refnum=w914, error in=w913) -> (error out=w921:errorcluster)  [unwired: 1 out]
                                n473 = call <vilib>:"Simple Error Handler.vi"("error in (no error)"=w921) -> ()  [unwired: 1 in, 8 out]
                              }
                              frame #1 {
                                w929 = "\t"
                                w947 = i16 4 ("width (-)")
                                n474 = Open/Create/Replace File(file path (use dialog)=w923, operation (0:open)=T3."open") -> (refnum out=w938:refnum<file>, error out=w937:errorcluster)  [unwired: 2 in, 3 out]
                                n475 = Multiply(x="Time RLC", y=u32 1000) -> (x*y=w926:u32)
                                n476 = Wait (ms)(milliseconds to wait=w926) -> ()  [unwired: 1 out]
                                n477 = Set File Position(refnum=w938, from (0:start)=enum16{"start", "end", "current"}."end", error in=w937) -> (refnum out=w940:refnum<file>, error out=w941:errorcluster)  [unwired: 1 in]
                                n478 = call "RLC_read.vi"("Path"=w927, "String"="cmd /c rlc_read_cAL.py") -> ("MEASURE A"=w928:dbl, "MEASURE V [V]"=w945:dbl, "concatenated string"=w949:string, "MEASURE B"=w946:dbl, "MEASURE I [A]"=w944:dbl)  [unwired: 1 out]
                                "MEASURE A" <- w928
                                "MEASURE B" <- w946
                                n479 = Number To Engineering String(2:w947, 4:w944) -> (0:w930:string)  [unwired: 2 in]
                                n480 = local write "RLC300 - digimess"(w949) -> ()
                                n481 = Number To Engineering String(2:w947, 4:w945) -> (0:w931:string)  [unwired: 2 in]
                                n482 = Number To Engineering String(2:w947, 4:w928) -> (0:w933:string)  [unwired: 2 in]
                                n483 = Number To Engineering String(2:w947, 4:w946) -> (0:w932:string)  [unwired: 2 in]
                                n484 = Concatenate Strings(w933, w929, w932, w929, w931, w929, w930, w929) -> (w934:string)
                                n485 = Write to Text File(file (use dialog)=w940, text=w934, error in=w941) -> (refnum out=w936:refnum<file>, error out=w935:errorcluster)  [unwired: 1 in, 1 out]
                                n486 = Close File(refnum=w936, error in=w935) -> (error out=w943:errorcluster)  [unwired: 1 out]
                                n487 = call <vilib>:"Simple Error Handler.vi"("error in (no error)"=w943) -> ()  [unwired: 1 in, 8 out]
                                "C-50-L" <- w948
                              }
                              frame #2 {
                                w958 = "\t"
                                w973 = i16 4 ("width (-)")
                                n488 = property on="Time RLC" class="DigNum (strict)"() -> ("Value"=w952:u32)  [unwired: 2 in, 2 out]
                                n489 = Wait (ms)(milliseconds to wait=w952) -> ()  [unwired: 1 out]
                                n490 = Open/Create/Replace File(file path (use dialog)=w951, operation (0:open)=T3."open") -> (refnum out=w967:refnum<file>, error out=w966:errorcluster)  [unwired: 2 in, 3 out]
                                n491 = Set File Position(refnum=w967, from (0:start)=enum16{"start", "end", "current"}."end", error in=w966) -> (refnum out=w969:refnum<file>, error out=w970:errorcluster)  [unwired: 1 in]
                                n492 = call "RLC_read.vi"("Path"=w953, "String"="cmd /c rlc_read_cAN.py") -> ("MEASURE A"=w954:dbl, "MEASURE V [V]"=w956:dbl, "concatenated string"=w976:string, "MEASURE B"=w957:dbl, "MEASURE I [A]"=w955:dbl)  [unwired: 1 out]
                                "MEASURE A 2" <- w954
                                "MEASURE B 2" <- w957
                                n493 = Number To Engineering String(2:w973, 4:w955) -> (0:w959:string)  [unwired: 2 in]
                                n494 = local write "RLC300 - digimess"(w976) -> ()
                                n495 = Number To Engineering String(2:w973, 4:w956) -> (0:w960:string)  [unwired: 2 in]
                                n496 = Number To Engineering String(2:w973, 4:w954) -> (0:w962:string)  [unwired: 2 in]
                                n497 = Number To Engineering String(2:w973, 4:w957) -> (0:w961:string)  [unwired: 2 in]
                                n498 = Concatenate Strings(w962, w958, w961, w958, w960, w958, w959, w958) -> (w963:string)
                                n499 = Write to Text File(file (use dialog)=w969, text=w963, error in=w970) -> (refnum out=w965:refnum<file>, error out=w964:errorcluster)  [unwired: 1 in, 1 out]
                                n500 = Close File(refnum=w965, error in=w964) -> (error out=w972:errorcluster)  [unwired: 1 out]
                                n501 = call <vilib>:"Simple Error Handler.vi"("error in (no error)"=w972) -> ()  [unwired: 1 in, 8 out]
                                "C-50-N" <- w974
                              }
                              frame #3 {
                                w984 = "\t"
                                w999 = i16 4 ("width (-)")
                                n502 = property on="Time RLC" class="DigNum (strict)"() -> ("Value"=w978:u32)  [unwired: 2 in, 2 out]
                                n503 = Wait (ms)(milliseconds to wait=w978) -> ()  [unwired: 1 out]
                                n504 = Open/Create/Replace File(file path (use dialog)=w977, operation (0:open)=T3."open") -> (refnum out=w993:refnum<file>, error out=w992:errorcluster)  [unwired: 2 in, 3 out]
                                n505 = Set File Position(refnum=w993, from (0:start)=enum16{"start", "end", "current"}."end", error in=w992) -> (refnum out=w995:refnum<file>, error out=w996:errorcluster)  [unwired: 1 in]
                                n506 = call "RLC_read.vi"("Path"=w979, "String"="cmd /c rlc_read_cBL.py") -> ("MEASURE A"=w980:dbl, "MEASURE V [V]"=w982:dbl, "concatenated string"=w1002:string, "MEASURE B"=w983:dbl, "MEASURE I [A]"=w981:dbl)  [unwired: 1 out]
                                "MEASURE A 3" <- w980
                                "MEASURE B 3" <- w983
                                n507 = Number To Engineering String(2:w999, 4:w981) -> (0:w985:string)  [unwired: 2 in]
                                n508 = local write "RLC300 - digimess"(w1002) -> ()
                                n509 = Number To Engineering String(2:w999, 4:w982) -> (0:w986:string)  [unwired: 2 in]
                                n510 = Number To Engineering String(2:w999, 4:w980) -> (0:w988:string)  [unwired: 2 in]
                                n511 = Number To Engineering String(2:w999, 4:w983) -> (0:w987:string)  [unwired: 2 in]
                                n512 = Concatenate Strings(w988, w984, w987, w984, w986, w984, w985, w984) -> (w989:string)
                                n513 = Write to Text File(file (use dialog)=w995, text=w989, error in=w996) -> (refnum out=w991:refnum<file>, error out=w990:errorcluster)  [unwired: 1 in, 1 out]
                                n514 = Close File(refnum=w991, error in=w990) -> (error out=w998:errorcluster)  [unwired: 1 out]
                                n515 = call <vilib>:"Simple Error Handler.vi"("error in (no error)"=w998) -> ()  [unwired: 1 in, 8 out]
                                "C-100-L" <- w1001
                              }
                              frame #4 {
                                w1010 = "\t"
                                w1025 = i16 4 ("width (-)")
                                n516 = property on="Time RLC" class="DigNum (strict)"() -> ("Value"=w1004:u32)  [unwired: 2 in, 2 out]
                                n517 = Wait (ms)(milliseconds to wait=w1004) -> ()  [unwired: 1 out]
                                n518 = Open/Create/Replace File(file path (use dialog)=w1003, operation (0:open)=T3."open") -> (refnum out=w1019:refnum<file>, error out=w1018:errorcluster)  [unwired: 2 in, 3 out]
                                n519 = Set File Position(refnum=w1019, from (0:start)=enum16{"start", "end", "current"}."end", error in=w1018) -> (refnum out=w1021:refnum<file>, error out=w1022:errorcluster)  [unwired: 1 in]
                                n520 = call "RLC_read.vi"("Path"=w1005, "String"="cmd /c rlc_read_cBN.py") -> ("MEASURE A"=w1006:dbl, "MEASURE V [V]"=w1008:dbl, "concatenated string"=w1028:string, "MEASURE B"=w1009:dbl, "MEASURE I [A]"=w1007:dbl)  [unwired: 1 out]
                                "MEASURE A 4" <- w1006
                                "MEASURE B 4" <- w1009
                                n521 = Number To Engineering String(2:w1025, 4:w1007) -> (0:w1011:string)  [unwired: 2 in]
                                n522 = local write "RLC300 - digimess"(w1028) -> ()
                                n523 = Number To Engineering String(2:w1025, 4:w1008) -> (0:w1012:string)  [unwired: 2 in]
                                n524 = Number To Engineering String(2:w1025, 4:w1006) -> (0:w1014:string)  [unwired: 2 in]
                                n525 = Number To Engineering String(2:w1025, 4:w1009) -> (0:w1013:string)  [unwired: 2 in]
                                n526 = Concatenate Strings(w1014, w1010, w1013, w1010, w1012, w1010, w1011, w1010) -> (w1015:string)
                                n527 = Write to Text File(file (use dialog)=w1021, text=w1015, error in=w1022) -> (refnum out=w1017:refnum<file>, error out=w1016:errorcluster)  [unwired: 1 in, 1 out]
                                n528 = Close File(refnum=w1017, error in=w1016) -> (error out=w1024:errorcluster)  [unwired: 1 out]
                                n529 = call <vilib>:"Simple Error Handler.vi"("error in (no error)"=w1024) -> ()  [unwired: 1 in, 8 out]
                                "C-100-N" <- w1026
                              }
                              frame #5 {
                                w1051 = "\t"
                                w1036 = i16 4 ("width (-)")
                                n530 = property on="Time RLC" class="DigNum (strict)"() -> ("Value"=w1030:u32)  [unwired: 2 in, 2 out]
                                n531 = Wait (ms)(milliseconds to wait=w1030) -> ()  [unwired: 1 out]
                                n532 = Open/Create/Replace File(file path (use dialog)=w1029, operation (0:open)=T3."open") -> (refnum out=w1042:refnum<file>, error out=w1043:errorcluster)  [unwired: 2 in, 3 out]
                                n533 = Set File Position(refnum=w1042, from (0:start)=enum16{"start", "end", "current"}."end", error in=w1043) -> (refnum out=w1040:refnum<file>, error out=w1039:errorcluster)  [unwired: 1 in]
                                n534 = call "RLC_read.vi"("Path"=w1031, "String"="cmd /c rlc_read_cCL.py") -> ("MEASURE A"=w1032:dbl, "MEASURE V [V]"=w1034:dbl, "concatenated string"=w1054:string, "MEASURE B"=w1035:dbl, "MEASURE I [A]"=w1033:dbl)  [unwired: 1 out]
                                "MEASURE A 5" <- w1032
                                "MEASURE B 5" <- w1035
                                n535 = Number To Engineering String(2:w1036, 4:w1033) -> (0:w1050:string)  [unwired: 2 in]
                                n536 = local write "RLC300 - digimess"(w1054) -> ()
                                n537 = Number To Engineering String(2:w1036, 4:w1034) -> (0:w1049:string)  [unwired: 2 in]
                                n538 = Number To Engineering String(2:w1036, 4:w1032) -> (0:w1047:string)  [unwired: 2 in]
                                n539 = Number To Engineering String(2:w1036, 4:w1035) -> (0:w1048:string)  [unwired: 2 in]
                                n540 = Concatenate Strings(w1047, w1051, w1048, w1051, w1049, w1051, w1050, w1051) -> (w1046:string)
                                n541 = Write to Text File(file (use dialog)=w1040, text=w1046, error in=w1039) -> (refnum out=w1044:refnum<file>, error out=w1045:errorcluster)  [unwired: 1 in, 1 out]
                                n542 = Close File(refnum=w1044, error in=w1045) -> (error out=w1037:errorcluster)  [unwired: 1 out]
                                n543 = call <vilib>:"Simple Error Handler.vi"("error in (no error)"=w1037) -> ()  [unwired: 1 in, 8 out]
                                "C-1K-L" <- w1053
                              }
                              frame #6 {
                                w1077 = "\t"
                                w1062 = i16 4 ("width (-)")
                                n544 = property on="Time RLC" class="DigNum (strict)"() -> ("Value"=w1056:u32)  [unwired: 2 in, 2 out]
                                n545 = Wait (ms)(milliseconds to wait=w1056) -> ()  [unwired: 1 out]
                                n546 = Open/Create/Replace File(file path (use dialog)=w1055, operation (0:open)=T3."open") -> (refnum out=w1068:refnum<file>, error out=w1069:errorcluster)  [unwired: 2 in, 3 out]
                                n547 = Set File Position(refnum=w1068, from (0:start)=enum16{"start", "end", "current"}."end", error in=w1069) -> (refnum out=w1066:refnum<file>, error out=w1065:errorcluster)  [unwired: 1 in]
                                n548 = call "RLC_read.vi"("Path"=w1057, "String"="cmd /c rlc_read_cCN.py") -> ("MEASURE A"=w1058:dbl, "MEASURE V [V]"=w1060:dbl, "concatenated string"=w1080:string, "MEASURE B"=w1061:dbl, "MEASURE I [A]"=w1059:dbl)  [unwired: 1 out]
                                "MEASURE A 6" <- w1058
                                "MEASURE B 6" <- w1061
                                n549 = Number To Engineering String(2:w1062, 4:w1059) -> (0:w1076:string)  [unwired: 2 in]
                                n550 = local write "RLC300 - digimess"(w1080) -> ()
                                n551 = Number To Engineering String(2:w1062, 4:w1060) -> (0:w1075:string)  [unwired: 2 in]
                                n552 = Number To Engineering String(2:w1062, 4:w1058) -> (0:w1073:string)  [unwired: 2 in]
                                n553 = Number To Engineering String(2:w1062, 4:w1061) -> (0:w1074:string)  [unwired: 2 in]
                                n554 = Concatenate Strings(w1073, w1077, w1074, w1077, w1075, w1077, w1076, w1077) -> (w1072:string)
                                n555 = Write to Text File(file (use dialog)=w1066, text=w1072, error in=w1065) -> (refnum out=w1070:refnum<file>, error out=w1071:errorcluster)  [unwired: 1 in, 1 out]
                                n556 = Close File(refnum=w1070, error in=w1071) -> (error out=w1063:errorcluster)  [unwired: 1 out]
                                n557 = call <vilib>:"Simple Error Handler.vi"("error in (no error)"=w1063) -> ()  [unwired: 1 in, 8 out]
                                "C-1K-N" <- w1078
                              }
                              frame #7 {
                                w1088 = "\t"
                                w1103 = i16 4 ("width (-)")
                                n558 = property on="Time RLC" class="DigNum (strict)"() -> ("Value"=w1082:u32)  [unwired: 2 in, 2 out]
                                n559 = Wait (ms)(milliseconds to wait=w1082) -> ()  [unwired: 1 out]
                                n560 = Open/Create/Replace File(file path (use dialog)=w1081, operation (0:open)=T3."open") -> (refnum out=w1097:refnum<file>, error out=w1096:errorcluster)  [unwired: 2 in, 3 out]
                                n561 = Set File Position(refnum=w1097, from (0:start)=enum16{"start", "end", "current"}."end", error in=w1096) -> (refnum out=w1099:refnum<file>, error out=w1100:errorcluster)  [unwired: 1 in]
                                n562 = call "RLC_read.vi"("Path"=w1083, "String"="cmd /c rlc_read_cDL.py") -> ("MEASURE A"=w1084:dbl, "MEASURE V [V]"=w1086:dbl, "concatenated string"=w1106:string, "MEASURE B"=w1087:dbl, "MEASURE I [A]"=w1085:dbl)  [unwired: 1 out]
                                "MEASURE A 7" <- w1084
                                "MEASURE B 7" <- w1087
                                n563 = Number To Engineering String(2:w1103, 4:w1085) -> (0:w1089:string)  [unwired: 2 in]
                                n564 = local write "RLC300 - digimess"(w1106) -> ()
                                n565 = Number To Engineering String(2:w1103, 4:w1086) -> (0:w1090:string)  [unwired: 2 in]
                                n566 = Number To Engineering String(2:w1103, 4:w1084) -> (0:w1092:string)  [unwired: 2 in]
                                n567 = Number To Engineering String(2:w1103, 4:w1087) -> (0:w1091:string)  [unwired: 2 in]
                                n568 = Concatenate Strings(w1092, w1088, w1091, w1088, w1090, w1088, w1089, w1088) -> (w1093:string)
                                n569 = Write to Text File(file (use dialog)=w1099, text=w1093, error in=w1100) -> (refnum out=w1095:refnum<file>, error out=w1094:errorcluster)  [unwired: 1 in, 1 out]
                                n570 = Close File(refnum=w1095, error in=w1094) -> (error out=w1102:errorcluster)  [unwired: 1 out]
                                n571 = call <vilib>:"Simple Error Handler.vi"("error in (no error)"=w1102) -> ()  [unwired: 1 in, 8 out]
                                "C-10K-L" <- w1105
                              }
                              frame #8 {
                                w1114 = "\t"
                                w1129 = i16 4 ("width (-)")
                                n572 = property on="Time RLC" class="DigNum (strict)"() -> ("Value"=w1108:u32)  [unwired: 2 in, 2 out]
                                n573 = Wait (ms)(milliseconds to wait=w1108) -> ()  [unwired: 1 out]
                                n574 = Open/Create/Replace File(file path (use dialog)=w1107, operation (0:open)=T3."open") -> (refnum out=w1123:refnum<file>, error out=w1122:errorcluster)  [unwired: 2 in, 3 out]
                                n575 = Set File Position(refnum=w1123, from (0:start)=enum16{"start", "end", "current"}."end", error in=w1122) -> (refnum out=w1125:refnum<file>, error out=w1126:errorcluster)  [unwired: 1 in]
                                n576 = call "RLC_read.vi"("Path"=w1109, "String"="cmd /c rlc_read_cDN.py") -> ("MEASURE A"=w1110:dbl, "MEASURE V [V]"=w1112:dbl, "concatenated string"=w1132:string, "MEASURE B"=w1113:dbl, "MEASURE I [A]"=w1111:dbl)  [unwired: 1 out]
                                "MEASURE A 8" <- w1110
                                "MEASURE B 8" <- w1113
                                n577 = Number To Engineering String(2:w1129, 4:w1111) -> (0:w1115:string)  [unwired: 2 in]
                                n578 = local write "RLC300 - digimess"(w1132) -> ()
                                n579 = Number To Engineering String(2:w1129, 4:w1112) -> (0:w1116:string)  [unwired: 2 in]
                                n580 = Number To Engineering String(2:w1129, 4:w1110) -> (0:w1118:string)  [unwired: 2 in]
                                n581 = Number To Engineering String(2:w1129, 4:w1113) -> (0:w1117:string)  [unwired: 2 in]
                                n582 = Concatenate Strings(w1118, w1114, w1117, w1114, w1116, w1114, w1115, w1114) -> (w1119:string)
                                n583 = Write to Text File(file (use dialog)=w1125, text=w1119, error in=w1126) -> (refnum out=w1121:refnum<file>, error out=w1120:errorcluster)  [unwired: 1 in, 1 out]
                                n584 = Close File(refnum=w1121, error in=w1120) -> (error out=w1128:errorcluster)  [unwired: 1 out]
                                n585 = call <vilib>:"Simple Error Handler.vi"("error in (no error)"=w1128) -> ()  [unwired: 1 in, 8 out]
                                "C-10K-N" <- w1131
                              }
                              frame #9 {
                                w1140 = "\t"
                                w1155 = i16 4 ("width (-)")
                                n586 = property on="Time RLC" class="DigNum (strict)"() -> ("Value"=w1134:u32)  [unwired: 2 in, 2 out]
                                n587 = Wait (ms)(milliseconds to wait=w1134) -> ()  [unwired: 1 out]
                                n588 = Open/Create/Replace File(file path (use dialog)=w1133, operation (0:open)=T3."open") -> (refnum out=w1149:refnum<file>, error out=w1148:errorcluster)  [unwired: 2 in, 3 out]
                                n589 = Set File Position(refnum=w1149, from (0:start)=enum16{"start", "end", "current"}."end", error in=w1148) -> (refnum out=w1151:refnum<file>, error out=w1152:errorcluster)  [unwired: 1 in]
                                n590 = call "RLC_read.vi"("Path"=w1135, "String"="cmd /c rlc_read_ZAL.py") -> ("MEASURE A"=w1136:dbl, "MEASURE V [V]"=w1138:dbl, "concatenated string"=w1157:string, "MEASURE B"=w1139:dbl, "MEASURE I [A]"=w1137:dbl)  [unwired: 1 out]
                                "MEASURE A 9" <- w1136
                                "MEASURE B 9" <- w1139
                                n591 = Number To Engineering String(2:w1155, 4:w1137) -> (0:w1141:string)  [unwired: 2 in]
                                n592 = local write "RLC300 - digimess"(w1157) -> ()
                                n593 = Number To Engineering String(2:w1155, 4:w1138) -> (0:w1142:string)  [unwired: 2 in]
                                n594 = Number To Engineering String(2:w1155, 4:w1136) -> (0:w1144:string)  [unwired: 2 in]
                                n595 = Number To Engineering String(2:w1155, 4:w1139) -> (0:w1143:string)  [unwired: 2 in]
                                n596 = Concatenate Strings(w1144, w1140, w1143, w1140, w1142, w1140, w1141, w1140) -> (w1145:string)
                                n597 = Write to Text File(file (use dialog)=w1151, text=w1145, error in=w1152) -> (refnum out=w1147:refnum<file>, error out=w1146:errorcluster)  [unwired: 1 in, 1 out]
                                n598 = Close File(refnum=w1147, error in=w1146) -> (error out=w1154:errorcluster)  [unwired: 1 out]
                                n599 = call <vilib>:"Simple Error Handler.vi"("error in (no error)"=w1154) -> ()  [unwired: 1 in, 8 out]
                                "Z-50-L" <- w1156
                              }
                              frame #10 {
                                w1166 = "\t"
                                w1181 = i16 4 ("width (-)")
                                n600 = property on="Time RLC" class="DigNum (strict)"() -> ("Value"=w1160:u32)  [unwired: 2 in, 2 out]
                                n601 = Wait (ms)(milliseconds to wait=w1160) -> ()  [unwired: 1 out]
                                n602 = Open/Create/Replace File(file path (use dialog)=w1159, operation (0:open)=T3."open") -> (refnum out=w1175:refnum<file>, error out=w1174:errorcluster)  [unwired: 2 in, 3 out]
                                n603 = Set File Position(refnum=w1175, from (0:start)=enum16{"start", "end", "current"}."end", error in=w1174) -> (refnum out=w1177:refnum<file>, error out=w1178:errorcluster)  [unwired: 1 in]
                                n604 = call "RLC_read.vi"("Path"=w1161, "String"="cmd /c rlc_read_ZAN.py") -> ("MEASURE A"=w1162:dbl, "MEASURE V [V]"=w1164:dbl, "concatenated string"=w1183:string, "MEASURE B"=w1165:dbl, "MEASURE I [A]"=w1163:dbl)  [unwired: 1 out]
                                "MEASURE A 10" <- w1162
                                "MEASURE B 10" <- w1165
                                n605 = Number To Engineering String(2:w1181, 4:w1163) -> (0:w1167:string)  [unwired: 2 in]
                                n606 = local write "RLC300 - digimess"(w1183) -> ()
                                n607 = Number To Engineering String(2:w1181, 4:w1164) -> (0:w1168:string)  [unwired: 2 in]
                                n608 = Number To Engineering String(2:w1181, 4:w1162) -> (0:w1170:string)  [unwired: 2 in]
                                n609 = Number To Engineering String(2:w1181, 4:w1165) -> (0:w1169:string)  [unwired: 2 in]
                                n610 = Concatenate Strings(w1170, w1166, w1169, w1166, w1168, w1166, w1167, w1166) -> (w1171:string)
                                n611 = Write to Text File(file (use dialog)=w1177, text=w1171, error in=w1178) -> (refnum out=w1173:refnum<file>, error out=w1172:errorcluster)  [unwired: 1 in, 1 out]
                                n612 = Close File(refnum=w1173, error in=w1172) -> (error out=w1180:errorcluster)  [unwired: 1 out]
                                n613 = call <vilib>:"Simple Error Handler.vi"("error in (no error)"=w1180) -> ()  [unwired: 1 in, 8 out]
                                "Z-50-N" <- w1182
                              }
                              frame #11 {
                                w1192 = "\t"
                                w1207 = i16 4 ("width (-)")
                                n614 = property on="Time RLC" class="DigNum (strict)"() -> ("Value"=w1186:u32)  [unwired: 2 in, 2 out]
                                n615 = Wait (ms)(milliseconds to wait=w1186) -> ()  [unwired: 1 out]
                                n616 = Open/Create/Replace File(file path (use dialog)=w1185, operation (0:open)=T3."open") -> (refnum out=w1201:refnum<file>, error out=w1200:errorcluster)  [unwired: 2 in, 3 out]
                                n617 = Set File Position(refnum=w1201, from (0:start)=enum16{"start", "end", "current"}."end", error in=w1200) -> (refnum out=w1203:refnum<file>, error out=w1204:errorcluster)  [unwired: 1 in]
                                n618 = call "RLC_read.vi"("Path"=w1187, "String"="cmd /c rlc_read_ZBL.py") -> ("MEASURE A"=w1188:dbl, "MEASURE V [V]"=w1190:dbl, "concatenated string"=w1209:string, "MEASURE B"=w1191:dbl, "MEASURE I [A]"=w1189:dbl)  [unwired: 1 out]
                                "MEASURE A 11" <- w1188
                                "MEASURE B 11" <- w1191
                                n619 = Number To Engineering String(2:w1207, 4:w1189) -> (0:w1193:string)  [unwired: 2 in]
                                n620 = local write "RLC300 - digimess"(w1209) -> ()
                                n621 = Number To Engineering String(2:w1207, 4:w1190) -> (0:w1194:string)  [unwired: 2 in]
                                n622 = Number To Engineering String(2:w1207, 4:w1188) -> (0:w1196:string)  [unwired: 2 in]
                                n623 = Number To Engineering String(2:w1207, 4:w1191) -> (0:w1195:string)  [unwired: 2 in]
                                n624 = Concatenate Strings(w1196, w1192, w1195, w1192, w1194, w1192, w1193, w1192) -> (w1197:string)
                                n625 = Write to Text File(file (use dialog)=w1203, text=w1197, error in=w1204) -> (refnum out=w1199:refnum<file>, error out=w1198:errorcluster)  [unwired: 1 in, 1 out]
                                n626 = Close File(refnum=w1199, error in=w1198) -> (error out=w1206:errorcluster)  [unwired: 1 out]
                                n627 = call <vilib>:"Simple Error Handler.vi"("error in (no error)"=w1206) -> ()  [unwired: 1 in, 8 out]
                                "Z-100-L" <- w1208
                              }
                              frame #12 {
                                w1218 = "\t"
                                w1233 = i16 4 ("width (-)")
                                n628 = property on="Time RLC" class="DigNum (strict)"() -> ("Value"=w1212:u32)  [unwired: 2 in, 2 out]
                                n629 = Wait (ms)(milliseconds to wait=w1212) -> ()  [unwired: 1 out]
                                n630 = Open/Create/Replace File(file path (use dialog)=w1211, operation (0:open)=T3."open") -> (refnum out=w1227:refnum<file>, error out=w1226:errorcluster)  [unwired: 2 in, 3 out]
                                n631 = Set File Position(refnum=w1227, from (0:start)=enum16{"start", "end", "current"}."end", error in=w1226) -> (refnum out=w1229:refnum<file>, error out=w1230:errorcluster)  [unwired: 1 in]
                                n632 = call "RLC_read.vi"("Path"=w1213, "String"="cmd /c rlc_read_ZBN.py") -> ("MEASURE A"=w1214:dbl, "MEASURE V [V]"=w1216:dbl, "concatenated string"=w1235:string, "MEASURE B"=w1217:dbl, "MEASURE I [A]"=w1215:dbl)  [unwired: 1 out]
                                "MEASURE A 12" <- w1214
                                "MEASURE B 12" <- w1217
                                n633 = Number To Engineering String(2:w1233, 4:w1215) -> (0:w1219:string)  [unwired: 2 in]
                                n634 = local write "RLC300 - digimess"(w1235) -> ()
                                n635 = Number To Engineering String(2:w1233, 4:w1216) -> (0:w1220:string)  [unwired: 2 in]
                                n636 = Number To Engineering String(2:w1233, 4:w1214) -> (0:w1222:string)  [unwired: 2 in]
                                n637 = Number To Engineering String(2:w1233, 4:w1217) -> (0:w1221:string)  [unwired: 2 in]
                                n638 = Concatenate Strings(w1222, w1218, w1221, w1218, w1220, w1218, w1219, w1218) -> (w1223:string)
                                n639 = Write to Text File(file (use dialog)=w1229, text=w1223, error in=w1230) -> (refnum out=w1225:refnum<file>, error out=w1224:errorcluster)  [unwired: 1 in, 1 out]
                                n640 = Close File(refnum=w1225, error in=w1224) -> (error out=w1232:errorcluster)  [unwired: 1 out]
                                n641 = call <vilib>:"Simple Error Handler.vi"("error in (no error)"=w1232) -> ()  [unwired: 1 in, 8 out]
                                "Z-100-N" <- w1234
                              }
                              frame #13 {
                                w1244 = "\t"
                                w1259 = i16 4 ("width (-)")
                                n642 = property on="Time RLC" class="DigNum (strict)"() -> ("Value"=w1238:u32)  [unwired: 2 in, 2 out]
                                n643 = Wait (ms)(milliseconds to wait=w1238) -> ()  [unwired: 1 out]
                                n644 = Open/Create/Replace File(file path (use dialog)=w1237, operation (0:open)=T3."open") -> (refnum out=w1253:refnum<file>, error out=w1252:errorcluster)  [unwired: 2 in, 3 out]
                                n645 = Set File Position(refnum=w1253, from (0:start)=enum16{"start", "end", "current"}."end", error in=w1252) -> (refnum out=w1255:refnum<file>, error out=w1256:errorcluster)  [unwired: 1 in]
                                n646 = call "RLC_read.vi"("Path"=w1239, "String"="cmd /c rlc_read_ZCL.py") -> ("MEASURE A"=w1240:dbl, "MEASURE V [V]"=w1242:dbl, "concatenated string"=w1261:string, "MEASURE B"=w1243:dbl, "MEASURE I [A]"=w1241:dbl)  [unwired: 1 out]
                                "MEASURE A 13" <- w1240
                                "MEASURE B 13" <- w1243
                                n647 = Number To Engineering String(2:w1259, 4:w1241) -> (0:w1245:string)  [unwired: 2 in]
                                n648 = local write "RLC300 - digimess"(w1261) -> ()
                                n649 = Number To Engineering String(2:w1259, 4:w1242) -> (0:w1246:string)  [unwired: 2 in]
                                n650 = Number To Engineering String(2:w1259, 4:w1240) -> (0:w1248:string)  [unwired: 2 in]
                                n651 = Number To Engineering String(2:w1259, 4:w1243) -> (0:w1247:string)  [unwired: 2 in]
                                n652 = Concatenate Strings(w1248, w1244, w1247, w1244, w1246, w1244, w1245, w1244) -> (w1249:string)
                                n653 = Write to Text File(file (use dialog)=w1255, text=w1249, error in=w1256) -> (refnum out=w1251:refnum<file>, error out=w1250:errorcluster)  [unwired: 1 in, 1 out]
                                n654 = Close File(refnum=w1251, error in=w1250) -> (error out=w1258:errorcluster)  [unwired: 1 out]
                                n655 = call <vilib>:"Simple Error Handler.vi"("error in (no error)"=w1258) -> ()  [unwired: 1 in, 8 out]
                                "Z-1K-L" <- w1260
                              }
                              frame #14 {
                                w1270 = "\t"
                                w1285 = i16 4 ("width (-)")
                                n656 = property on="Time RLC" class="DigNum (strict)"() -> ("Value"=w1264:u32)  [unwired: 2 in, 2 out]
                                n657 = Wait (ms)(milliseconds to wait=w1264) -> ()  [unwired: 1 out]
                                n658 = Open/Create/Replace File(file path (use dialog)=w1263, operation (0:open)=T3."open") -> (refnum out=w1279:refnum<file>, error out=w1278:errorcluster)  [unwired: 2 in, 3 out]
                                n659 = Set File Position(refnum=w1279, from (0:start)=enum16{"start", "end", "current"}."end", error in=w1278) -> (refnum out=w1281:refnum<file>, error out=w1282:errorcluster)  [unwired: 1 in]
                                n660 = call "RLC_read.vi"("Path"=w1265, "String"="cmd /c rlc_read_ZCN.py") -> ("MEASURE A"=w1266:dbl, "MEASURE V [V]"=w1268:dbl, "concatenated string"=w1287:string, "MEASURE B"=w1269:dbl, "MEASURE I [A]"=w1267:dbl)  [unwired: 1 out]
                                "MEASURE A 14" <- w1266
                                "MEASURE B 14" <- w1269
                                n661 = Number To Engineering String(2:w1285, 4:w1267) -> (0:w1271:string)  [unwired: 2 in]
                                n662 = local write "RLC300 - digimess"(w1287) -> ()
                                n663 = Number To Engineering String(2:w1285, 4:w1268) -> (0:w1272:string)  [unwired: 2 in]
                                n664 = Number To Engineering String(2:w1285, 4:w1266) -> (0:w1274:string)  [unwired: 2 in]
                                n665 = Number To Engineering String(2:w1285, 4:w1269) -> (0:w1273:string)  [unwired: 2 in]
                                n666 = Concatenate Strings(w1274, w1270, w1273, w1270, w1272, w1270, w1271, w1270) -> (w1275:string)
                                n667 = Write to Text File(file (use dialog)=w1281, text=w1275, error in=w1282) -> (refnum out=w1277:refnum<file>, error out=w1276:errorcluster)  [unwired: 1 in, 1 out]
                                n668 = Close File(refnum=w1277, error in=w1276) -> (error out=w1284:errorcluster)  [unwired: 1 out]
                                n669 = call <vilib>:"Simple Error Handler.vi"("error in (no error)"=w1284) -> ()  [unwired: 1 in, 8 out]
                                "Z-1K-N" <- w1286
                              }
                              frame #15 {
                                w1296 = "\t"
                                w1311 = i16 4 ("width (-)")
                                n670 = property on="Time RLC" class="DigNum (strict)"() -> ("Value"=w1290:u32)  [unwired: 2 in, 2 out]
                                n671 = Wait (ms)(milliseconds to wait=w1290) -> ()  [unwired: 1 out]
                                n672 = Open/Create/Replace File(file path (use dialog)=w1289, operation (0:open)=T3."open") -> (refnum out=w1305:refnum<file>, error out=w1304:errorcluster)  [unwired: 2 in, 3 out]
                                n673 = Set File Position(refnum=w1305, from (0:start)=enum16{"start", "end", "current"}."end", error in=w1304) -> (refnum out=w1307:refnum<file>, error out=w1308:errorcluster)  [unwired: 1 in]
                                n674 = call "RLC_read.vi"("Path"=w1291, "String"="cmd /c rlc_read_ZDL.py") -> ("MEASURE A"=w1292:dbl, "MEASURE V [V]"=w1294:dbl, "concatenated string"=w1313:string, "MEASURE B"=w1295:dbl, "MEASURE I [A]"=w1293:dbl)  [unwired: 1 out]
                                "MEASURE A 15" <- w1292
                                "MEASURE B 15" <- w1295
                                n675 = Number To Engineering String(2:w1311, 4:w1293) -> (0:w1297:string)  [unwired: 2 in]
                                n676 = local write "RLC300 - digimess"(w1313) -> ()
                                n677 = Number To Engineering String(2:w1311, 4:w1294) -> (0:w1298:string)  [unwired: 2 in]
                                n678 = Number To Engineering String(2:w1311, 4:w1292) -> (0:w1300:string)  [unwired: 2 in]
                                n679 = Number To Engineering String(2:w1311, 4:w1295) -> (0:w1299:string)  [unwired: 2 in]
                                n680 = Concatenate Strings(w1300, w1296, w1299, w1296, w1298, w1296, w1297, w1296) -> (w1301:string)
                                n681 = Write to Text File(file (use dialog)=w1307, text=w1301, error in=w1308) -> (refnum out=w1303:refnum<file>, error out=w1302:errorcluster)  [unwired: 1 in, 1 out]
                                n682 = Close File(refnum=w1303, error in=w1302) -> (error out=w1310:errorcluster)  [unwired: 1 out]
                                n683 = call <vilib>:"Simple Error Handler.vi"("error in (no error)"=w1310) -> ()  [unwired: 1 in, 8 out]
                                "Z-10K-L" <- w1312
                              }
                              frame #16 {
                                w1323 = "\t"
                                w1338 = i16 4 ("width (-)")
                                n684 = property on="Time RLC" class="DigNum (strict)"() -> ("Value"=w1316:u32)  [unwired: 2 in, 2 out]
                                n685 = Wait (ms)(milliseconds to wait=w1316) -> ()  [unwired: 1 out]
                                n686 = Open/Create/Replace File(file path (use dialog)=w1315, operation (0:open)=T3."open") -> (refnum out=w1332:refnum<file>, error out=w1331:errorcluster)  [unwired: 2 in, 3 out]
                                n687 = Set File Position(refnum=w1332, from (0:start)=enum16{"start", "end", "current"}."end", error in=w1331) -> (refnum out=w1334:refnum<file>, error out=w1335:errorcluster)  [unwired: 1 in]
                                n688 = call "RLC_read.vi"("Path"=w1317, "String"="cmd /c rlc_read_ZDN.py") -> ("MEASURE A"=w1318:dbl, "MEASURE V [V]"=w1321:dbl, "concatenated string"=w1340:string, "MEASURE B"=w1322:dbl, "MEASURE I [A]"=w1320:dbl)  [unwired: 1 out]
                                "MEASURE A 16" <- w1318
                                "MEASURE B 16" <- w1322
                                n689 = Number To Engineering String(2:w1338, 4:w1320) -> (0:w1324:string)  [unwired: 2 in]
                                n690 = local write "RLC300 - digimess"(w1340) -> ()
                                n691 = Number To Engineering String(2:w1338, 4:w1321) -> (0:w1325:string)  [unwired: 2 in]
                                n692 = Number To Engineering String(2:w1338, 4:w1318) -> (0:w1327:string)  [unwired: 2 in]
                                n693 = Number To Engineering String(2:w1338, 4:w1322) -> (0:w1326:string)  [unwired: 2 in]
                                n694 = Concatenate Strings(w1327, w1323, w1326, w1323, w1325, w1323, w1324, w1323, "\r\n") -> (w1328:string)
                                n695 = Write to Text File(file (use dialog)=w1334, text=w1328, error in=w1335) -> (refnum out=w1330:refnum<file>, error out=w1329:errorcluster)  [unwired: 1 in, 1 out]
                                n696 = Close File(refnum=w1330, error in=w1329) -> (error out=w1337:errorcluster)  [unwired: 1 out]
                                n697 = call <vilib>:"Simple Error Handler.vi"("error in (no error)"=w1337) -> ()  [unwired: 1 in, 8 out]
                                "Z-10K-N" <- w1339
                              }
                              frame #17 {
                                n698 = local write "Z-50-L"(w1343) -> ()
                                n699 = local write "Z-1K-L"(w1343) -> ()
                                n700 = local write "Z-1K-N"(w1343) -> ()
                                n701 = local write "C-50-N"(w1343) -> ()
                                n702 = local write "C-50-L"(w1343) -> ()
                                n703 = local write "Z-50-N"(w1343) -> ()
                                n704 = local write "C-1K-N"(w1343) -> ()
                                n705 = local write "C-1K-L"(w1343) -> ()
                                n706 = local write "Z-100-L"(w1343) -> ()
                                n707 = local write "Z-100-N"(w1343) -> ()
                                n708 = local write "Z-10K-L"(w1343) -> ()
                                n709 = local write "Z-10K-N"(w1343) -> ()
                                n710 = local write "C-10K-N"(w1343) -> ()
                                n711 = local write "C-10K-L"(w1343) -> ()
                                n712 = local write "C-100-N"(w1343) -> ()
                                n713 = local write "C-100-L"(w1343) -> ()
                              }
                            }
                          }
                          n714 = call <vilib>:"Mean.vi"("X"=w874) -> ("mean"=w856:dbl)  [unwired: 1 out]
                          "mean 2" <- w856
                          n715 = call <vilib>:"Mean.vi"("X"=w873) -> ("mean"=w855:dbl)  [unwired: 1 out]
                          "mean 3" <- w855
                          n716 = call <vilib>:"Mean.vi"("X"=w872) -> ("mean"=w854:dbl)  [unwired: 1 out]
                          "mean 4" <- w854
                          n717 = call <vilib>:"Mean.vi"("X"=w871) -> ("mean"=w853:dbl)  [unwired: 1 out]
                          "mean 5" <- w853
                          n718 = call <vilib>:"Mean.vi"("X"=w870) -> ("mean"=w852:dbl)  [unwired: 1 out]
                          "mean 6" <- w852
                          n719 = call <vilib>:"Mean.vi"("X"=w869) -> ("mean"=w851:dbl)  [unwired: 1 out]
                          "mean 7" <- w851
                          n720 = call <vilib>:"Mean.vi"("X"=w868) -> ("mean"=w850:dbl)  [unwired: 1 out]
                          "mean 8" <- w850
                          n721 = call <vilib>:"Mean.vi"("X"=w867) -> ("mean"=w849:dbl)  [unwired: 1 out]
                          "mean 9" <- w849
                          n722 = call <vilib>:"Mean.vi"("X"=w866) -> ("mean"=w848:dbl)  [unwired: 1 out]
                          "mean 10" <- w848
                          n723 = call <vilib>:"Mean.vi"("X"=w865) -> ("mean"=w847:dbl)  [unwired: 1 out]
                          "mean 11" <- w847
                          n724 = call <vilib>:"Mean.vi"("X"=w864) -> ("mean"=w846:dbl)  [unwired: 1 out]
                          "mean 12" <- w846
                          n725 = call <vilib>:"Mean.vi"("X"=w863) -> ("mean"=w845:dbl)  [unwired: 1 out]
                          "mean 13" <- w845
                          n726 = call <vilib>:"Mean.vi"("X"=w862) -> ("mean"=w844:dbl)  [unwired: 1 out]
                          "mean 14" <- w844
                          n727 = call <vilib>:"Mean.vi"("X"=w861) -> ("mean"=w843:dbl)  [unwired: 1 out]
                          "mean 15" <- w843
                          n728 = call <vilib>:"Mean.vi"("X"=w875) -> ("mean"=w857:dbl)  [unwired: 1 out]
                          "mean" <- w857
                          n729 = call <vilib>:"Mean.vi"("X"=w860) -> ("mean"=w842:dbl)  [unwired: 1 out]
                          "mean 16" <- w842
                        }
                      }
                    }
                    frame #2 {
                      n730 = case shown="True" w1344 {
                        tunnel: w1361 -> [_ w1377]
                        tunnel: w1360 -> [_ w1376]
                        tunnel: w1359 -> [_ w1375]
                        tunnel: w1358 -> [_ w1374]
                        tunnel: w1357 -> [_ w1373]
                        tunnel: w1356 -> [_ w1372]
                        tunnel: w1355 -> [_ w1371]
                        tunnel: w1354 -> [_ w1370]
                        tunnel: w1353 -> [_ w1369]
                        tunnel: w1352 -> [_ w1368]
                        tunnel: w1351 -> [_ w1367]
                        tunnel: w1350 -> [_ w1366]
                        tunnel: w1349 -> [_ w1365]
                        tunnel: w1348 -> [_ w1364]
                        tunnel: w1347 -> [_ w1363]
                        tunnel: w1346 -> [_ w1362]
                        frame False {
                        }
                        frame True {
                          w1391 = "\t"
                          w1408 = i16 4 ("precision (6)")
                          n731 = property on="SET" class="DigNum (strict)"() -> ("Value"=w1409:i32)  [unwired: 2 in, 2 out]
                          n732 = Number To Engineering String(2:w1408, 4:w1362) -> (0:w1405:string)  [unwired: 2 in]
                          n733 = Number To Engineering String(2:w1408, 4:w1376) -> (0:w1404:string)  [unwired: 2 in]
                          n734 = Number To Engineering String(2:w1408, 4:w1375) -> (0:w1403:string)  [unwired: 2 in]
                          n735 = Number To Engineering String(2:w1408, 4:w1374) -> (0:w1402:string)  [unwired: 2 in]
                          n736 = Number To Engineering String(2:w1408, 4:w1373) -> (0:w1401:string)  [unwired: 2 in]
                          n737 = Number To Engineering String(2:w1408, 4:w1372) -> (0:w1400:string)  [unwired: 2 in]
                          n738 = Number To Engineering String(2:w1408, 4:w1371) -> (0:w1399:string)  [unwired: 2 in]
                          n739 = Number To Engineering String(2:w1408, 4:w1370) -> (0:w1398:string)  [unwired: 2 in]
                          n740 = Number To Engineering String(2:w1408, 4:w1369) -> (0:w1397:string)  [unwired: 2 in]
                          n741 = Number To Engineering String(2:w1408, 4:w1368) -> (0:w1396:string)  [unwired: 2 in]
                          n742 = Number To Engineering String(2:w1408, 4:w1367) -> (0:w1395:string)  [unwired: 2 in]
                          n743 = Number To Engineering String(2:w1408, 4:w1366) -> (0:w1394:string)  [unwired: 2 in]
                          n744 = Number To Engineering String(2:w1408, 4:w1365) -> (0:w1393:string)  [unwired: 2 in]
                          n745 = Number To Engineering String(2:w1408, 4:w1364) -> (0:w1392:string)  [unwired: 2 in]
                          n746 = Number To Engineering String(2:w1408, 4:w1377) -> (0:w1406:string)  [unwired: 2 in]
                          n747 = Number To Engineering String(2:w1408, 4:w1363) -> (0:w1390:string)  [unwired: 2 in]
                          n748 = Number To Decimal String(number=w1409) -> (decimal integer string=w1407:string)  [unwired: 1 in]
                          n749 = property on="path RLC_mean" class="Path"() -> ("Value"=w1378:path)  [unwired: 2 in, 2 out]
                          n750 = Open/Create/Replace File(file path (use dialog)=w1378, operation (0:open)=T3."open") -> (refnum out=w1383:refnum<file>, error out=w1382:errorcluster)  [unwired: 2 in, 3 out]
                          n751 = Concatenate Strings(w1407, w1391, w1406, w1391, w1405, w1391, w1404, w1391, w1403, w1391, w1402, w1391, w1401, w1391, w1400, w1391, w1399, w1391, w1398, w1391, w1397, w1391, w1396, w1391, w1395, w1391, w1394, w1391, w1393, w1391, w1392, w1391, w1390, "\r\n") -> (w1379:string)
                          n752 = Set File Position(refnum=w1383, from (0:start)=enum16{"start", "end", "current"}."end", error in=w1382) -> (refnum out=w1385:refnum<file>, error out=w1386:errorcluster)  [unwired: 1 in]
                          n753 = Write to Text File(file (use dialog)=w1385, text=w1379, error in=w1386) -> (refnum out=w1381:refnum<file>, error out=w1380:errorcluster)  [unwired: 1 in, 1 out]
                          n754 = Close File(refnum=w1381, error in=w1380) -> (error out=w1388:errorcluster)  [unwired: 1 out]
                          n755 = call <vilib>:"Simple Error Handler.vi"("error in (no error)"=w1388) -> ()  [unwired: 1 in, 8 out]
                        }
                      }
                    }
                  }
                  n756 = local write "graph RLC"(w793) -> ()
                }
                frame 9 {
                  n757 = flat-sequence {
                    tunnel: w1448 -> [w1459]
                    tunnel: [w1459] -> w1447
                    tunnel: [w1453] -> w1446
                    tunnel: [w1452] -> w1445
                    tunnel: w1447 -> [w1484]
                    tunnel: w1446 -> [_]
                    tunnel: w1445 -> [w1481]
                    frame #0 {
                      n758 = property on="SET" class="DigNum (strict)"() -> ("Value"=w1457:i32)  [unwired: 2 in, 2 out]
                      n759 = Increment(x=w1457) -> (x+1=w1452:i32)
                      n760 = property on="P_max camara" class="DigNum (strict)"() -> ("Value"=w1450:dbl)  [unwired: 2 in, 2 out]
                      n761 = local write "SET"(w1452) -> ()
                      n762 = property on="Camara 2" class="Slide (strict)"() -> ("Value"=w1451:dbl)  [unwired: 2 in, 2 out]
                      n763 = case shown="False" "Boolean" {
                        selector: "Boolean" -> [w1465 w1470]
                        tunnel: [w1467 w1474] -> w1454
                        tunnel: w1452 -> [w1468 _]
                        frame False {
                          n764 = local write "Boolean 2"(w1465) -> ()
                          n765 = Index Array(array="Array", index=w1468) -> (element=w1467:dbl)
                          n766 = Not(x=w1465) -> (.not. x?=→"Boolean 3":bool)
                        }
                        frame True {
                          n767 = property on="Set P auto" class="DigNum (strict)"() -> ("Value"=w1472:dbl)  [unwired: 2 in, 2 out]
                          n768 = Add(x="Step P", y=w1472) -> (x+y=w1474:dbl)
                          n769 = Not(x=w1470) -> (.not. x?=w1471:bool)
                          n770 = local write "Boolean 3"(w1471) -> ()
                          "Boolean 2" <- w1470
                        }
                      }
                      n771 = Greater?(x=w1451, y=w1450) -> (0:w1449:bool)
                      n772 = case shown="True" w1449 {
                        frame False {
                        }
                        frame True {
                          n773 = property on="Desc SET" class="DigNum (strict)"() -> ("Value"=w1461:i32)  [unwired: 2 in, 2 out]
                          n774 = local write "Descarga"(TRUE ("Descarga")) -> ()
                          n775 = Increment(x=w1461) -> (x+1=w1460:i32)
                          n776 = local write "Desc SET"(w1460) -> ()
                        }
                      }
                      n777 = Greater?(x=w1454, y="P_max") -> (0:w1456:bool)
                      n778 = case shown="True" w1456 {
                        tunnel: [w1463 w1464] -> w1453
                        tunnel: "P_max" -> [_ w1464]
                        tunnel: w1454 -> [w1463 _]
                        frame False {
                        }
                        frame True {
                        }
                      }
                      n779 = local write "Set P auto"(w1453) -> ()
                    }
                    frame #1 {
                      n780 = property on="Desc SET" class="DigNum (strict)"() -> ("Value"=w1476:i32)  [unwired: 2 in, 2 out]
                      n781 = Quotient & Remainder(x=w1481, y="Step ZPit") -> (x-y*floor(x/y)=w1482:dbl)  [unwired: 1 out]
                      n782 = Greater Than 0?(x=w1476) -> (x > 0?=w1478:bool)
                      n783 = Equal To 0?(x=w1482) -> (x = 0?=w1480:bool)
                      "Read ZPit" <- w1480
                      n784 = property on="Descarga" class="Bool (strict)"() -> ("Value"=w1475:bool)  [unwired: 2 in, 2 out]
                      n785 = And(x=w1478, y=w1475) -> (x .and. y?=w1477:bool)
                      n786 = case shown="True" w1477 {
                        tunnel: w1480 -> [w1485 _]
                        tunnel: [w1485 w1486] -> w1479
                        frame False {
                        }
                        frame True {
                          w1486 = TRUE
                          n787 = local write "Read ZPit"(w1486) -> ()
                        }
                      }
                      n788 = case shown="True" w1479 {
                        tunnel: w1484 -> [_ w1488]
                        frame False {
                          n789 = local write "Estagio auto"(11 ("Estagio auto")) -> ()
                        }
                        frame True {
                          n790 = Greater?(x=w1488, y=1.0) -> (0:w1493:bool)
                          n791 = case shown="True" w1493 {
                            tunnel: [FALSE ("Boolean") TRUE ("Boolean")] -> w1491
                            frame False {
                              w1513 = TRUE ("Boolean")
                              n792 = local write "Vácuo 2"(w1513) -> ()
                              n793 = Multiply(x="ZPf2 time", y=0.0741) -> (x*y=w1508:dbl)
                              n794 = local write "String"("Limpar volume referencia" ("String")) -> ()
                              n795 = Add(x=w1508, y=1.9801) -> (x+y=w1506:dbl)
                              n796 = call "Controle_vacuo.vi"("time (s) to wait vacuo"=w1506, "Boolean"=w1513) -> ("Vacuo"=w1514:bool)  [unwired: 9 in]
                              n797 = local write "Vácuo 2"(w1514) -> ()
                            }
                            frame True {
                              n798 = property on="ATM wait" class="DigNum (strict)"() -> ("Value"=w1515:u32)  [unwired: 2 in, 2 out]
                              n799 = call "Controle_ATM.vi"("seconds to wait"=w1515) -> ("String 2"=w1518:string, "Atm"=w1517:bool)  [unwired: 9 in]
                              n800 = local write "Atm 2"(w1517) -> ()
                              n801 = local write "String"(w1518) -> ()
                            }
                          }
                          n802 = for {
                            N: 1 -> [_]
                            tunnel: [w1495] -> w1490
                            tunnel: w1491 -> [w1495]
                            n803 = Wait (ms)(milliseconds to wait=u32 500 ("x")) -> ()  [unwired: 1 out]
                          }
                          n804 = case shown="True" w1490 {
                            frame False {
                              n805 = local write "Estagio auto"(10 ("Estagio auto")) -> ()
                            }
                            frame True {
                              w1504 = TRUE ("Boolean")
                              n806 = property on="ZPf2 time" class="DigNum (strict)"() -> ("Value"=w1498:dbl)  [unwired: 2 in, 2 out]
                              n807 = local write "Estagio auto"(10 ("Estagio auto")) -> ()
                              n808 = Multiply(x=w1498, y=0.0741) -> (x*y=w1500:dbl)
                              n809 = local write "Vácuo 2"(w1504) -> ()
                              n810 = local write "String"("Limpar volume referencia" ("String")) -> ()
                              n811 = Add(x=w1500, y=1.9801) -> (x+y=w1497:dbl)
                              n812 = call "Controle_vacuo.vi"("time (s) to wait vacuo"=w1497, "Boolean"=w1504) -> ("Vacuo"=w1505:bool)  [unwired: 9 in]
                              n813 = local write "Vácuo 2"(w1505) -> ()
                            }
                          }
                        }
                      }
                    }
                  }
                }
                frame 10 {
                  n814 = property on="Contador" class="DigNum (strict)"() -> ("Value"=w1520:i32)  [unwired: 2 in, 2 out]
                  n815 = Increment(x=w1520) -> (x+1=w1522:i32)
                  n816 = property on="N fit 2" class="DigNum (strict)"() -> ("Value"=w1519:i32)  [unwired: 2 in, 2 out]
                  n817 = local write "String"("Ler ZPf2 e T" ("String")) -> ()
                  n818 = Equal?(x=w1522, y=w1519) -> (x = y?=w1521:bool)
                  n819 = case shown="True" w1521 {
                    frame False {
                    }
                    frame True {
                      n820 = local write "Estagio auto"(11 ("Estagio auto")) -> ()
                    }
                  }
                }
                frame 11 {
                  n821 = property on="Contador" class="DigNum (strict)"() -> ("Value"=w1528:i32)  [unwired: 2 in, 2 out]
                  n822 = Increment(x=w1528) -> (x+1=w1529:i32)
                  n823 = property on="N fit 2" class="DigNum (strict)"() -> ("Value"=w1525:i32)  [unwired: 2 in, 2 out]
                  n824 = Equal?(x=w1529, y=w1525) -> (x = y?=w1527:bool)
                  n825 = case shown="True" w1527 {
                    tunnel: w1530 -> [_ w1541]
                    tunnel: w1526 -> [_ w1531]
                    frame False {
                    }
                    frame True {
                      w1532 = i16 3 ("precision (6)")
                      w1535 = "\t"
                      n826 = property on="Read ZPit" class="Bool (strict)"() -> ("Value"=w1536:bool)  [unwired: 2 in, 2 out]
                      n827 = property on="T fit" class="DigNum (strict)"() -> ("Value"=w1537:dbl)  [unwired: 2 in, 2 out]
                      n828 = case shown="False" w1536 {
                        tunnel: ["  ==>" w1547] -> w1540
                        tunnel: w1532 -> [_ w1546]
                        frame False {
                        }
                        frame True {
                          n829 = property on="P fit" class="DigNum (strict)"() -> ("Value"=w1545:dbl)  [unwired: 2 in, 2 out]
                          n830 = Number To Fractional String(number=w1545, precision (6)=w1546) -> (F-format string=w1547:string)  [unwired: 2 in]
                        }
                      }
                      n831 = Number To Fractional String(number=w1537, precision (6)=w1532) -> (F-format string=w1539:string)  [unwired: 2 in]
                      n832 = Number To Fractional String(number=w1531, precision (6)=w1532) -> (F-format string=w1534:string)  [unwired: 2 in]
                      n833 = Concatenate Strings(w1540, w1535, w1539, w1535, w1534, "\r\n") -> (w1538:string)
                      n834 = flat-sequence {
                        tunnel: [w1551] -> w1543
                        tunnel: [w1550] -> w1542
                        tunnel: w1538 -> [w1549]
                        tunnel: w1541 -> [w1548]
                        tunnel: w1543 -> [w1565]
                        tunnel: w1542 -> [w1564]
                        frame #0 {
                          n835 = Open/Create/Replace File(file path (use dialog)=w1548, operation (0:open)=T3."open") -> (refnum out=w1557:refnum<file>, error out=w1558:errorcluster)  [unwired: 2 in, 3 out]
                          n836 = Set File Position(refnum=w1557, from (0:start)=enum16{"start", "end", "current"}."end", error in=w1558) -> (refnum out=w1555:refnum<file>, error out=w1554:errorcluster)  [unwired: 1 in]
                          n837 = Write to Text File(file (use dialog)=w1555, text=w1549, error in=w1554) -> (refnum out=w1559:refnum<file>, error out=w1560:errorcluster)  [unwired: 2 out]
                          n838 = Close File(refnum=w1559, error in=w1560) -> (path=w1551:path, error out=w1552:errorcluster)
                          n839 = call <vilib>:"Simple Error Handler.vi"("error in (no error)"=w1552) -> ("error out"=w1550:errorcluster)  [unwired: 1 in, 7 out]
                        }
                        frame #1 {
                          w1561 = TRUE ("ZPit")
                          n840 = Wait (ms)(milliseconds to wait=u32 500) -> ()  [unwired: 1 out]
                          n841 = local write "T 2"(w1561) -> ()
                          n842 = local write "ZPf2 2"(w1561) -> ()
                          n843 = Read from Text File(file (use dialog)=w1565, count=-1 ("Count  3"), error in=w1564) -> (refnum out=w1566:refnum<file>, text=w1570:string, error out=w1567:errorcluster)  [unwired: 1 in, 1 out]
                          n844 = local write "String 3"(w1570) -> ()
                          n845 = Close File(refnum=w1566, error in=w1567) -> (error out=w1568:errorcluster)  [unwired: 1 out]
                          n846 = local write "String"("abrir valvula entrada gas" ("String")) -> ()
                          n847 = call <vilib>:"Simple Error Handler.vi"("error in (no error)"=w1568) -> ()  [unwired: 1 in, 8 out]
                        }
                        frame #2 {
                          n848 = property on="Desc SET" class="DigNum (strict)"() -> ("Value"=w1572:i32)  [unwired: 2 in, 2 out]
                          n849 = Greater Than 0?(x=w1572) -> (x > 0?=w1571:bool)
                          n850 = property on="Camara 2" class="Slide (strict)"() -> ("Value"=w1579:dbl)  [unwired: 2 in, 2 out]
                          n851 = Greater?(x=w1579, y="P_max camara") -> (0:w1577:bool)
                          n852 = property on="Carga" class="Bool (strict)"() -> ("Value"=w1576:bool)  [unwired: 2 in, 2 out]
                          n853 = And(x=w1577, y=w1576) -> (x .and. y?=w1574:bool)
                          n854 = case shown="False" w1571 {
                            tunnel: w1574 -> [w1580 _]
                            tunnel: [w1580 TRUE] -> w1573
                            frame False {
                            }
                            frame True {
                            }
                          }
                          n855 = case shown="True" w1573 {
                            tunnel: [5 ("N fit") w1586] -> w1575
                            frame False {
                              n856 = local write "Estagio auto"(0 ("Estagio auto")) -> ()
                              "Carga" <- TRUE
                              "Descarga" <- FALSE
                            }
                            frame True {
                              n857 = local write "teste slope"(0 ("teste slope")) -> ()
                              n858 = local write "Carga"(FALSE ("Carga")) -> ()
                              n859 = local write "Descarga"(TRUE ("Descarga")) -> ()
                              n860 = local write "Estagio auto"(12 ("Estagio auto")) -> ()
                              n861 = property on="N fit 2" class="DigNum (strict)"() -> ("Value"=w1586:i32)  [unwired: 2 in, 2 out]
                            }
                          }
                          n862 = local write "N fit"(w1575) -> ()
                        }
                      }
                    }
                  }
                }
                frame 12 {
                  w1596 = "\t"
                  n863 = property on="SET" class="DigNum (strict)"() -> ("Value"=w1600:i32)  [unwired: 2 in, 2 out]
                  n864 = Number To Decimal String(number=w1600) -> (decimal integer string=w1603:string)  [unwired: 1 in]
                  n865 = Number To Fractional String(number=0.0, precision (6)=i16 3) -> (F-format string=w1597:string)  [unwired: 2 in]
                  n866 = Concatenate Strings(w1603, w1596, w1597, w1596, w1597, w1596) -> (w1602:string)
                  n867 = flat-sequence {
                    tunnel: w1599 -> [w1608]
                    tunnel: w1602 -> [w1609]
                    tunnel: [w1609] -> w1595
                    tunnel: [w1608] -> w1594
                    tunnel: [w1613] -> w1605
                    tunnel: [w1612] -> w1604
                    tunnel: w1595 -> [w1611]
                    tunnel: w1594 -> [w1610]
                    tunnel: [w1610] -> w1593
                    tunnel: w1605 -> [w1629]
                    tunnel: w1604 -> [w1628]
                    tunnel: w1593 -> [w1623]
                    tunnel: [w1623] -> w1592
                    tunnel: w1592 -> [w1637]
                    tunnel: [w1636] -> w1591
                    tunnel: w1591 -> [w1674]
                    frame #0 {
                      w1607 = FALSE ("ZPit 2")
                      n868 = Wait (ms)(milliseconds to wait=u32 1000) -> ()  [unwired: 1 out]
                      n869 = local write "ZPit 2"(w1607) -> ()
                      n870 = local write "Pit 2"(w1607) -> ()
                      n871 = local write "Pf2 2"(w1607) -> ()
                      n872 = local write "ZPf2 2"(w1607) -> ()
                      n873 = local write "T 2"(w1607) -> ()
                    }
                    frame #1 {
                      n874 = Open/Create/Replace File(file path (use dialog)=w1610, operation (0:open)=T3."open") -> (refnum out=w1619:refnum<file>, error out=w1620:errorcluster)  [unwired: 2 in, 3 out]
                      n875 = Set File Position(refnum=w1619, from (0:start)=enum16{"start", "end", "current"}."end", error in=w1620) -> (refnum out=w1617:refnum<file>, error out=w1616:errorcluster)  [unwired: 1 in]
                      n876 = Write to Text File(file (use dialog)=w1617, text=w1611, error in=w1616) -> (refnum out=w1621:refnum<file>, error out=w1622:errorcluster)  [unwired: 2 out]
                      n877 = Close File(refnum=w1621, error in=w1622) -> (path=w1613:path, error out=w1614:errorcluster)
                      n878 = call <vilib>:"Simple Error Handler.vi"("error in (no error)"=w1614) -> ("error out"=w1612:errorcluster)  [unwired: 1 in, 7 out]
                    }
                    frame #2 {
                      w1624 = TRUE ("ZPit")
                      n879 = local write "Estagio auto"(7 ("Estagio auto")) -> ()
                      n880 = Wait (ms)(milliseconds to wait=u32 500) -> ()  [unwired: 1 out]
                      n881 = local write "ZPit 2"(w1624) -> ()
                      n882 = local write "Pit 2"(w1624) -> ()
                      n883 = Read from Text File(file (use dialog)=w1629, count=-1 ("Count  3"), error in=w1628) -> (refnum out=w1630:refnum<file>, text=w1634:string, error out=w1631:errorcluster)  [unwired: 1 in, 1 out]
                      n884 = local write "String 3"(w1634) -> ()
                      n885 = Close File(refnum=w1630, error in=w1631) -> (error out=w1632:errorcluster)  [unwired: 1 out]
                      n886 = call <vilib>:"Simple Error Handler.vi"("error in (no error)"=w1632) -> ()  [unwired: 1 in, 8 out]
                      n887 = local write "String"("abrir valvula camara" ("String")) -> ()
                    }
                    frame #3 {
                      n888 = property on="Camara 2" class="Slide (strict)"() -> ("Value"=w1640:dbl)  [unwired: 2 in, 2 out]
                      n889 = Less?(x=w1640, y="P_min descarga") -> (x < y?=w1635:bool)
                      n890 = property on="Efetuados" class="DigNum (strict)"() -> ("Value"=w1638:dbl)  [unwired: 2 in, 2 out]
                      n891 = case shown="True" w1635 {
                        tunnel: w1638 -> [_ w1669]
                        tunnel: w1637 -> [_ w1658]
                        tunnel: [TRUE ("data") FALSE ("data")] -> w1636
                        tunnel: w1635 -> [_ w1647]
                        frame False {
                          n892 = property on="Desc SET" class="DigNum (strict)"() -> ("Value"=w1642:i32)  [unwired: 2 in, 2 out]
                          n893 = Increment(x=w1642) -> (x+1=→"Desc SET":i32)
                        }
                        frame True {
                          w1656 = "\r\n"
                          n894 = Increment(x=w1669) -> (x+1=w1644:dbl)
                          "Efetuados" <- w1644
                          n895 = local write "Estagio auto"(0 ("Estagio auto")) -> ()
                          n896 = local write "SET"(0 ("SET")) -> ()
                          n897 = local write "Desc SET"(0 ("Desc SET")) -> ()
                          n898 = local write "Descarga"(FALSE ("Descarga")) -> ()
                          n899 = local write "Carga"(TRUE ("Carga")) -> ()
                          n900 = local write "Set P auto"(0.5 ("Set P auto")) -> ()
                          n901 = Open/Create/Replace File(file path (use dialog)=w1658, operation (0:open)=T3."open") -> (refnum out=w1664:refnum<file>, error out=w1665:errorcluster)  [unwired: 2 in, 3 out]
                          n902 = Less Or Equal?(x="Ciclos", y=w1644) -> (x <= y?=w1645:bool)
                          n903 = And(x=w1647, y=w1645) -> (x .and. y?=w1648:bool)
                          n904 = Set File Position(refnum=w1664, from (0:start)=enum16{"start", "end", "current"}."end", error in=w1665) -> (refnum out=w1662:refnum<file>, error out=w1661:errorcluster)  [unwired: 1 in]
                          n905 = case shown="False" w1648 {
                            frame False {
                              n906 = local write "FIM"(FALSE ("FIM")) -> ()
                            }
                            frame True {
                              w1673 = 1 ("N fit")
                              n907 = local write "Auto Ctrl"(FALSE ("Auto Ctrl")) -> ()
                              n908 = local write "N fit"(w1673) -> ()
                              n909 = local write "N to fit"(w1673) -> ()
                              "FIM" <- TRUE ("stop")
                            }
                          }
                          n910 = Concatenate Strings(w1656, ">>>>>>>>>>>>>>" ("string"), w1656, w1656) -> (w1655:string)
                          n911 = Write to Text File(file (use dialog)=w1662, text=w1655, error in=w1661) -> (refnum out=w1666:refnum<file>, error out=w1667:errorcluster)  [unwired: 2 out]
                          n912 = Close File(refnum=w1666, error in=w1667) -> (error out=w1659:errorcluster)  [unwired: 1 out]
                          n913 = call <vilib>:"Simple Error Handler.vi"("error in (no error)"=w1659) -> ()  [unwired: 1 in, 8 out]
                        }
                      }
                    }
                    frame #4 {
                      w1676 = T7 3 items=["no dialog", "OK message", "continue or stop message", "OK message + warnings", "continue/stop + warnings"] ("type of dialog (OK msg:1)")
                      n914 = local write "Câmara 2"(w1674) -> ()
                      n915 = call-poly <vilib>:"DAQmx Create Virtual Channel.vi"("lines"=tag "Dev1/port0/line3") -> ("task out"=w1685:refnum<k21>, "error out"=w1684:errorcluster)  [unwired: 13 in]
                      n916 = call <vilib>:"DAQmx Start Task.vi"("task/channels in"=w1685, "error in"=w1684) -> ("task out"=w1683:refnum<k21>, "error out"=w1682:errorcluster)  [unwired: 12 in]
                      n917 = call-poly <vilib>:"DAQmx Write.vi"("task/channels in"=w1683, "data"=w1674, "error in"=w1682) -> ("task out"=w1678:refnum<k21>, "error out"=w1677:errorcluster)  [unwired: 10 in, 1 out]
                      n918 = call <vilib>:"DAQmx Stop Task.vi"("task/channels in"=w1678, "error in"=w1677) -> ("task out"=w1680:refnum<k21>, "error out"=w1681:errorcluster)  [unwired: 12 in]
                      n919 = call <vilib>:"DAQmx Clear Task.vi"("task in"=w1680, "error in"=w1681) -> ("error out"=w1675:errorcluster)  [unwired: 13 in]
                      n920 = call <vilib>:"Simple Error Handler.vi"("type of dialog (OK msg:1)"=w1676, "error in (no error)"=w1675) -> ()  [unwired: 3 in, 5 out]
                    }
                  }
                }
              }
            }
          }
          n921 = Index Array(array=w264, index=w262) -> (element=w261:dbl)
          n922 = Index Array(array=w263, index=w262) -> (element=w260:dbl)
          n923 = Bundle("Real 2D Array"=w267, "Best Linear Fit"=w279) -> (w278:T8)  [unwired: 1 in]
          n924 = Bundle("Real 2D Array"=w267, "Best Polynomial Fit"=w268) -> (w265:T9)  [unwired: 1 in]
          n925 = Bundle("Real 2D Array"=w267, "Best Polynomial Fit"=w269) -> (w266:T9)  [unwired: 1 in]
          n926 = case shown="True" w259 {
            tunnel: w261 -> [_ w1688]
            tunnel: w260 -> [_ w1687]
            tunnel: w254 -> [_ w1686]
            frame False {
            }
            frame True {
              "P fit" <- w1688
              "T fit" <- w1687
              "P (bar/s)" <- w1686
            }
          }
          n927 = Build Array(w277, w278, w265) -> (→"Linear T":T10)
          n928 = Bundle("Real 2D Array"=w267, "Best Linear Fit"=w274) -> (w275:T8)  [unwired: 1 in]
          n929 = Build Array(w276, w275, w266) -> (→"Linear P":T10)
          "Contador" <- w258
        }
        n930 = local write "P subarray 2"(dbl[] [0.0, 1.0] ("subarray")) -> ()
        n931 = local write "T subarray 3"(dbl[] [0.0, 1.0] ("subarray")) -> ()
        n932 = local write "time subarray"(dbl[] [0.0, 1.0] ("subarray")) -> ()
      }
    }
    n933 = case shown="False" "Auto Ctrl" {
      tunnel: [TRUE ("Auto Ctrl") FALSE ("Auto Ctrl")] -> w49
      frame False {
      }
      frame True {
      }
    }
    n934 = Exclusive Or(1:w46, 2:"stop") -> (0:w48:bool)
    n935 = case shown="True" "Ligar RLC" {
      tunnel: w43 -> [_ w168]
      frame False {
      }
      frame True {
        w176 = "\t"
        w197 = "\t"
        w180 = "\r"
        w173 = "\r\n"
        w213 = "\r"
        w203 = "\t"
        n936 = Strip Path(path=w168) -> (stripped path=w169:path, name=w172:string)
        n937 = Get Date/Time String(date format (0)=enum16{"short", "long", "abbreviated"}."short", want seconds? (F)=TRUE) -> (date string=w220:string, time string=w219:string)  [unwired: 1 in]
        n938 = Concatenate Strings("SET" ("Nota 4"), w176, "DATE" ("Nota 4"), w176, "TIME" ("Nota 4"), w176, w197, "P (BAR)" ("Nota 4"), w197, "T (ºC)" ("Nota 4"), w197, "C-50-L" ("Nota 4"), w197, "C-50-N" ("Nota 4"), w197, "C-100-L" ("Nota 4"), w197, "C-100-N" ("Nota 4"), w197, "C-1K-L" ("Nota 4"), w197, "C-1K-N" ("Nota 4"), w197, "C-10K-L" ("Nota 4"), w197, "C-10K-N" ("Nota 4"), w197, "Z-50-L" ("Nota 4"), w197, "Z-50-N" ("Nota 4"), w197, "Z-100-L" ("Nota 4"), w197, "Z-100-N" ("Nota 4"), w197, "Z-1K-L" ("Nota 4"), w197, "Z-1K-N" ("Nota 4"), w197, "Z-10K-L" ("Nota 4"), w197, "Z-10K-N" ("Nota 4")) -> (w181:string)
        n939 = Concatenate Strings(w220, w203, w219) -> (w215:string)
        n940 = Concatenate Strings(w172, "_RLC_CDH completo" ("string")) -> (w170:string)
        n941 = Concatenate Strings("Sievert RLC - CDH:" ("string"), w203, w173, w173) -> (w201:string)
        n942 = Concatenate Strings("Data Table" ("string"), w180, "==========" ("string"), w180, w181, w180) -> (w214:string)
        n943 = File Dialog(6:".txt" ("pattern label"), 9:w170, 11:w169) -> (0:w211:errorcluster, 3:w212:path)  [unwired: 2 in, 4 out]
        n944 = Open/Create/Replace File(file path (use dialog)=w212, error in=w211, operation (0:open)=T3."replace or create with confirmation", access (0:read/write)=enum16{"read/write", "read-only", "write-only"}."read/write") -> (refnum out=w208:refnum<file>, error out=w207:errorcluster)  [unwired: 3 out]
        n945 = Concatenate Strings(w215, w213, w213, w201, w213, w213, "Nota 01: MEDIDAS COM RLC 300 - MULTILEITURA" ("Nota 4"), w213, w213, w214) -> (w218:string)
        n946 = Write to Text File(file (use dialog)=w208, text=w218, error in=w207) -> (refnum out=w206:refnum<file>, error out=w204:errorcluster)  [unwired: 1 in, 1 out]
        n947 = Close File(refnum=w206, error in=w204) -> (path=w200:path)  [unwired: 1 out]
        n948 = local write "path RLC_completo"(w200) -> ()
      }
    }
    n949 = case shown="True" "Ligar RLC" {
      tunnel: w43 -> [_ w111]
      frame False {
      }
      frame True {
        w120 = "\t"
        w141 = "\t"
        w124 = "\r"
        w117 = "\r\n"
        w156 = "\r"
        w146 = "\t"
        n950 = Strip Path(path=w111) -> (stripped path=w113:path, name=w116:string)
        n951 = Get Date/Time String(date format (0)=enum16{"short", "long", "abbreviated"}."short", want seconds? (F)=TRUE) -> (date string=w163:string, time string=w162:string)  [unwired: 1 in]
        n952 = Concatenate Strings("SET" ("Nota 4"), w120, "DATE" ("Nota 4"), w120, "TIME" ("Nota 4"), w120, w141, "P (BAR)" ("Nota 4"), w141, "T (ºC)" ("Nota 4"), w141, "C-50-L" ("Nota 4"), w141, "C-50-N" ("Nota 4"), w141, "C-100-L" ("Nota 4"), w141, "C-100-N" ("Nota 4"), w141, "C-1K-L" ("Nota 4"), w141, "C-1K-N" ("Nota 4"), w141, "C-10K-L" ("Nota 4"), w141, "C-10K-N" ("Nota 4"), w141, "Z-50-L" ("Nota 4"), w141, "Z-50-N" ("Nota 4"), w141, "Z-100-L" ("Nota 4"), w141, "Z-100-N" ("Nota 4"), w141, "Z-1K-L" ("Nota 4"), w141, "Z-1K-N" ("Nota 4"), w141, "Z-10K-L" ("Nota 4"), w141, "Z-10K-N" ("Nota 4")) -> (w125:string)
        n953 = Concatenate Strings(w163, w146, w162) -> (w158:string)
        n954 = Concatenate Strings(w116, "_RLC_CDH mean" ("string")) -> (w114:string)
        n955 = Concatenate Strings("Sievert RLC - CDH:" ("string"), w146, w117, w117) -> (w144:string)
        n956 = Concatenate Strings("Data Table" ("string"), w124, "==========" ("string"), w124, w125, w124) -> (w157:string)
        n957 = File Dialog(6:".txt" ("pattern label"), 9:w114, 11:w113) -> (0:w154:errorcluster, 3:w155:path)  [unwired: 2 in, 4 out]
        n958 = Open/Create/Replace File(file path (use dialog)=w155, error in=w154, operation (0:open)=T3."replace or create with confirmation", access (0:read/write)=enum16{"read/write", "read-only", "write-only"}."read/write") -> (refnum out=w151:refnum<file>, error out=w150:errorcluster)  [unwired: 3 out]
        n959 = Concatenate Strings(w158, w156, w156, w144, w156, w156, "Nota 01: MEDIDAS COM RLC 300 - MULTILEITURA" ("Nota 4"), w156, w156, w157) -> (w161:string)
        n960 = Write to Text File(file (use dialog)=w151, text=w161, error in=w150) -> (refnum out=w149:refnum<file>, error out=w147:errorcluster)  [unwired: 1 in, 1 out]
        n961 = Close File(refnum=w149, error in=w147) -> (path=w112:path)  [unwired: 1 out]
        n962 = local write "path RLC_mean"(w112) -> ()
      }
    }
    n963 = case shown="True" "RLC on/off" {
      tunnel: w36 -> [_ w54]
      frame False {
      }
      frame True {
        n964 = call "RLC READ DINAMICO.vi"("Boolean"="graph RLC", "Path"=w54, "String"="Combo Box") -> ("MEASURE R [Ohm ]"=w58:dbl, "MEASURE C [F ]"=w57:dbl)  [unwired: 7 in]
        "MEASURE C [F ]" <- w57
        n965 = Merge Signals(w57, w58) -> (→"Waveform Chart":dynamicdata)
        "String 4" <- "Combo Box"
      }
    }
    n966 = case shown="True" "Manual Ctrl" {
      tunnel: w36 -> [_ w1770]
      tunnel: "RLC on/off" -> [_ w1769]
      tunnel: [FALSE w1772] -> w38
      frame False {
      }
      frame True {
        w1784 = 0 ("polynomial order")
        n967 = for {
          N: "N to fit" -> [_]
          tunnel: [w2457] -> w1759 mode=indexing
          tunnel: [w2462] -> w1777 mode=indexing
          tunnel: [w2462] -> w1763 mode=indexing
          tunnel: [w2450] -> w1768 mode=indexing
          i -> [w2462]
          n968 = case shown="False" "Clear" {
            frame False {
            }
            frame True {
              n969 = property on="P-manual" class="WFChart (strict)"("History Data"=dynamicdata[] []) -> ()  [unwired: 2 in, 2 out]
            }
          }
          n970 = case shown="True" "Câmara" {
            frame False {
            }
            frame True {
              n971 = property on="Vol Ref" class="Slide (strict)"() -> ("Value"=w2509:dbl)  [unwired: 2 in, 2 out]
              n972 = local write "Camara"(w2509) -> ()
            }
          }
          n973 = case shown="True" "Guardar\nCinetica" {
            frame False {
            }
            frame True {
              n974 = feedback #2() -> (w2464:bool)  [unwired: 1 in]
              "x >= y?" <- w2464
              n975 = call "Elapsed Time"("Reset"=w2464) -> ("Elapsed Time (s)"=w2466:dbl)  [unwired: 11 in, 7 out]
              "Elapsed Time (sec)" <- w2466
              n976 = case shown="True" w2464 {
                frame False {
                }
                frame True {
                  n977 = flat-sequence {
                    tunnel: [w2481] -> w2469
                    tunnel: [w2480] -> w2468
                    tunnel: w2469 -> [w2499]
                    tunnel: w2468 -> [w2498]
                    frame #0 {
                      w2475 = "\t"
                      w2470 = i16 6 ("precision (6)")
                      n978 = call "Advanced Serial.vi"() -> ("V-P01(mV)"=w2473:dbl, "V-P02(mV)"=w2471:dbl)  [unwired: 7 in, 7 out]
                      n979 = property on="P cinetica mean" class="DigNum (strict)"() -> ("Value"=w2478:dbl)  [unwired: 2 in, 2 out]
                      n980 = property on="T cinetica mean 2" class="DigNum (strict)"() -> ("Value"=w2477:dbl)  [unwired: 2 in, 2 out]
                      n981 = Number To Fractional String(number=w2478, precision (6)=w2470) -> (F-format string=w2493:string)  [unwired: 2 in]
                      n982 = Number To Fractional String(number=w2477, precision (6)=w2470) -> (F-format string=w2492:string)  [unwired: 2 in]
                      n983 = Number To Fractional String(number=w2473, precision (6)=w2470) -> (F-format string=w2476:string)  [unwired: 2 in]
                      n984 = Number To Fractional String(number=w2471, precision (6)=w2470) -> (F-format string=w2472:string)  [unwired: 2 in]
                      n985 = property on="path 2_cinetica" class="Path"() -> ("Value"=w2479:path)  [unwired: 2 in, 2 out]
                      n986 = Get Date/Time String(date format (0)=enum16{"short", "long", "abbreviated"}."short", want seconds? (F)=TRUE) -> (date string=w2495:string, time string=w2494:string)  [unwired: 1 in]
                      n987 = Open/Create/Replace File(file path (use dialog)=w2479, operation (0:open)=T3."open") -> (refnum out=w2488:refnum<file>, error out=w2489:errorcluster)  [unwired: 2 in, 3 out]
                      n988 = Concatenate Strings(w2495, w2475, w2494, w2475, w2493, w2475, w2492, w2475, w2476, w2475, w2472, "\r\n") -> (w2482:string)
                      n989 = Set File Position(refnum=w2488, from (0:start)=enum16{"start", "end", "current"}."end", error in=w2489) -> (refnum out=w2486:refnum<file>, error out=w2485:errorcluster)  [unwired: 1 in]
                      n990 = Write to Text File(file (use dialog)=w2486, text=w2482, error in=w2485) -> (refnum out=w2490:refnum<file>, error out=w2491:errorcluster)  [unwired: 2 out]
                      n991 = Close File(refnum=w2490, error in=w2491) -> (path=w2481:path, error out=w2483:errorcluster)
                      n992 = call <vilib>:"Simple Error Handler.vi"("error in (no error)"=w2483) -> ("error out"=w2480:errorcluster)  [unwired: 1 in, 7 out]
                    }
                    frame #1 {
                      n993 = Read from Text File(file (use dialog)=w2499, count=-1 ("Count  3"), error in=w2498) -> (refnum out=w2500:refnum<file>, text=w2504:string, error out=w2501:errorcluster)  [unwired: 1 in, 1 out]
                      n994 = local write "String_cinetica"(w2504) -> ()
                      n995 = Close File(refnum=w2500, error in=w2501) -> (error out=w2502:errorcluster)  [unwired: 1 out]
                      n996 = call <vilib>:"Simple Error Handler.vi"("error in (no error)"=w2502) -> ()  [unwired: 1 in, 8 out]
                    }
                    frame #2 {
                      n997 = local write "P T  index"(0 ("P T  index")) -> ()
                      n998 = local write "T subarray 2"(dbl[] [0.0, 1.0] ("subarray")) -> ()
                      n999 = local write "P subarray"(dbl[] [0.0, 1.0] ("subarray")) -> ()
                    }
                  }
                }
              }
              n1000 = Greater Or Equal?(x=w2466, y="seconds") -> (x >= y?=w2467:bool)
              n1001 = feedback-in #2(w2467) -> ()
            }
          }
          n1002 = property on="correção NTC" class="DigNum (strict)"() -> ("Value"=w2453:dbl)  [unwired: 2 in, 2 out]
          n1003 = call "Read P T.vi"("correção NTC"=w2453) -> ("Sievert01"=w2446:dbl, "mean H2 sensor"=→"mean H2 sensor (V)":dbl, "termopar K"=w2451:dbl, "output NTC"=w2450:dbl, "P Set 2 Output 2"=w2449:dbl)  [unwired: 3 in, 7 out]
          "termopar K" <- w2451
          "output NTC" <- w2450
          n1004 = stacked-sequence {
            tunnel: "Entrada Gás" -> [w2540 _ _ _]
            tunnel: "Vácuo" -> [_ w2552 _ _]
            tunnel: "Câmara" -> [_ _ w2564 _]
            tunnel: "ATM" -> [_ _ _ w2576]
            frame #0 {
              w2545 = T7 3 items=["no dialog", "OK message", "continue or stop message", "OK message + warnings", "continue/stop + warnings"] ("type of dialog (OK msg:1)")
              n1005 = property on="Entrada gás" class="Bool (strict)"("Value"=w2540) -> ()  [unwired: 2 in, 2 out]
              n1006 = call-poly <vilib>:"DAQmx Create Virtual Channel.vi"("lines"=tag "Dev1/port0/line1") -> ("task out"=w2543:refnum<k21>, "error out"=w2544:errorcluster)  [unwired: 13 in]
              n1007 = call <vilib>:"DAQmx Start Task.vi"("task/channels in"=w2543, "error in"=w2544) -> ("task out"=w2546:refnum<k21>, "error out"=w2547:errorcluster)  [unwired: 12 in]
              n1008 = call-poly <vilib>:"DAQmx Write.vi"("task/channels in"=w2546, "data"=w2540, "error in"=w2547) -> ("task out"=w2551:refnum<k21>, "error out"=w2548:errorcluster)  [unwired: 10 in, 1 out]
              n1009 = call <vilib>:"DAQmx Stop Task.vi"("task/channels in"=w2551, "error in"=w2548) -> ("task out"=w2550:refnum<k21>, "error out"=w2549:errorcluster)  [unwired: 12 in]
              n1010 = call <vilib>:"DAQmx Clear Task.vi"("task in"=w2550, "error in"=w2549) -> ("error out"=w2542:errorcluster)  [unwired: 13 in]
              n1011 = call <vilib>:"Simple Error Handler.vi"("type of dialog (OK msg:1)"=w2545, "error in (no error)"=w2542) -> ()  [unwired: 3 in, 5 out]
            }
            frame #1 {
              w2557 = T7 3 items=["no dialog", "OK message", "continue or stop message", "OK message + warnings", "continue/stop + warnings"] ("type of dialog (OK msg:1)")
              n1012 = property on="Vácuo" class="Bool (strict)"("Value"=w2552) -> ()  [unwired: 2 in, 2 out]
              n1013 = call-poly <vilib>:"DAQmx Create Virtual Channel.vi"("lines"=tag "Dev1/port0/line2") -> ("task out"=w2555:refnum<k21>, "error out"=w2556:errorcluster)  [unwired: 13 in]
              n1014 = call <vilib>:"DAQmx Start Task.vi"("task/channels in"=w2555, "error in"=w2556) -> ("task out"=w2558:refnum<k21>, "error out"=w2559:errorcluster)  [unwired: 12 in]
              n1015 = call-poly <vilib>:"DAQmx Write.vi"("task/channels in"=w2558, "data"=w2552, "error in"=w2559) -> ("task out"=w2563:refnum<k21>, "error out"=w2560:errorcluster)  [unwired: 10 in, 1 out]
              n1016 = call <vilib>:"DAQmx Stop Task.vi"("task/channels in"=w2563, "error in"=w2560) -> ("task out"=w2562:refnum<k21>, "error out"=w2561:errorcluster)  [unwired: 12 in]
              n1017 = call <vilib>:"DAQmx Clear Task.vi"("task in"=w2562, "error in"=w2561) -> ("error out"=w2554:errorcluster)  [unwired: 13 in]
              n1018 = call <vilib>:"Simple Error Handler.vi"("type of dialog (OK msg:1)"=w2557, "error in (no error)"=w2554) -> ()  [unwired: 3 in, 5 out]
            }
            frame #2 {
              w2569 = T7 3 items=["no dialog", "OK message", "continue or stop message", "OK message + warnings", "continue/stop + warnings"] ("type of dialog (OK msg:1)")
              n1019 = property on="Câmara" class="Bool (strict)"("Value"=w2564) -> ()  [unwired: 2 in, 2 out]
              n1020 = call-poly <vilib>:"DAQmx Create Virtual Channel.vi"("lines"=tag "Dev1/port0/line3") -> ("task out"=w2567:refnum<k21>, "error out"=w2568:errorcluster)  [unwired: 13 in]
              n1021 = call <vilib>:"DAQmx Start Task.vi"("task/channels in"=w2567, "error in"=w2568) -> ("task out"=w2570:refnum<k21>, "error out"=w2571:errorcluster)  [unwired: 12 in]
              n1022 = call-poly <vilib>:"DAQmx Write.vi"("task/channels in"=w2570, "data"=w2564, "error in"=w2571) -> ("task out"=w2575:refnum<k21>, "error out"=w2572:errorcluster)  [unwired: 10 in, 1 out]
              n1023 = call <vilib>:"DAQmx Stop Task.vi"("task/channels in"=w2575, "error in"=w2572) -> ("task out"=w2574:refnum<k21>, "error out"=w2573:errorcluster)  [unwired: 12 in]
              n1024 = call <vilib>:"DAQmx Clear Task.vi"("task in"=w2574, "error in"=w2573) -> ("error out"=w2566:errorcluster)  [unwired: 13 in]
              n1025 = call <vilib>:"Simple Error Handler.vi"("type of dialog (OK msg:1)"=w2569, "error in (no error)"=w2566) -> ()  [unwired: 3 in, 5 out]
            }
            frame #3 {
              w2581 = T7 3 items=["no dialog", "OK message", "continue or stop message", "OK message + warnings", "continue/stop + warnings"] ("type of dialog (OK msg:1)")
              n1026 = property on="Atm" class="Bool (strict)"("Value"=w2576) -> ()  [unwired: 2 in, 2 out]
              n1027 = call-poly <vilib>:"DAQmx Create Virtual Channel.vi"("lines"=tag "Dev1/port0/line4") -> ("task out"=w2579:refnum<k21>, "error out"=w2580:errorcluster)  [unwired: 13 in]
              n1028 = call <vilib>:"DAQmx Start Task.vi"("task/channels in"=w2579, "error in"=w2580) -> ("task out"=w2582:refnum<k21>, "error out"=w2583:errorcluster)  [unwired: 12 in]
              n1029 = call-poly <vilib>:"DAQmx Write.vi"("task/channels in"=w2582, "data"=w2576, "error in"=w2583) -> ("task out"=w2587:refnum<k21>, "error out"=w2584:errorcluster)  [unwired: 10 in, 1 out]
              n1030 = call <vilib>:"DAQmx Stop Task.vi"("task/channels in"=w2587, "error in"=w2584) -> ("task out"=w2586:refnum<k21>, "error out"=w2585:errorcluster)  [unwired: 12 in]
              n1031 = call <vilib>:"DAQmx Clear Task.vi"("task in"=w2586, "error in"=w2585) -> ("error out"=w2578:errorcluster)  [unwired: 13 in]
              n1032 = call <vilib>:"Simple Error Handler.vi"("type of dialog (OK msg:1)"=w2581, "error in (no error)"=w2578) -> ()  [unwired: 3 in, 5 out]
            }
          }
          n1033 = Multiply(x=w2449, y=10.0) -> (x*y=w2457:dbl)
          n1034 = local write "Vol Ref"(w2457) -> ()
          n1035 = Multiply(x=w2446, y=10.0) -> (x*y=w2447:dbl)
          n1036 = stacked-sequence {
            tunnel: w2457 -> [w2532 _]
            tunnel: w2450 -> [w2511 _]
            frame #0 {
              w2510 = 2 ("y")
              n1037 = property on="P subarray" class="Arr (strict)"() -> ("Value"=w2534:dbl[])  [unwired: 2 in, 2 out]
              n1038 = property on="P T  index" class="DigNum (strict)"() -> ("Value"=w2512:i32)  [unwired: 2 in, 2 out]
              n1039 = Replace Array Subset(array=w2534, new element=w2532, index=w2512) -> (w2530:dbl[])
              n1040 = property on="T subarray 2" class="Arr (strict)"() -> ("Value"=w2521:dbl[])  [unwired: 2 in, 2 out]
              n1041 = Replace Array Subset(array=w2521, new element=w2511, index=w2512) -> (w2518:dbl[])
              n1042 = call-poly <vilib>:"Array To Matrix.vi"("Real 1D Array"=w2530) -> ("Real Matrix (Column Vector)"=w2537:T5)
              n1043 = Matrix Size(0:w2537) -> (1:w2536:i32, 2:w2535:i32)
              n1044 = call-poly <vilib>:"Array To Matrix.vi"("Real 1D Array"=w2518) -> ("Real Matrix (Column Vector)"=w2524:T5)
              n1045 = Matrix Size(0:w2524) -> (1:w2523:i32, 2:w2522:i32)
              n1046 = Increment(x=w2536) -> (x+1=w2525:i32)
              n1047 = Subtract(x=w2525, y=w2510) -> (x-y=w2526:i32)
              n1048 = Resize Matrix(1:w2535, 2:w2525, 4:w2537) -> (0:w2533:T5)
              n1049 = Increment(x=w2523) -> (x+1=w2513:i32)
              n1050 = Subtract(x=w2513, y=w2510) -> (x-y=w2514:i32)
              n1051 = Resize Matrix(1:w2522, 2:w2513, 4:w2524) -> (0:w2520:T5)
              n1052 = call-poly <vilib>:"Matrix To Array.vi"("Real Matrix"=w2533) -> ("Real 2D Array"=w2528:dbl[][])
              n1053 = call-poly <vilib>:"Matrix To Array.vi"("Real Matrix"=w2520) -> ("Real 2D Array"=w2516:dbl[][])
              n1054 = Reshape Array(w2528, w2525) -> (w2527:dbl[])
              n1055 = Reshape Array(w2516, w2513) -> (w2515:dbl[])
              n1056 = local write "P subarray"(w2527) -> ()
              n1057 = Reshape Array(w2527, w2526) -> (w2529:dbl[])
              n1058 = local write "T subarray 2"(w2515) -> ()
              n1059 = call <vilib>:"Mean.vi"("X"=w2529) -> ("mean"=→"P cinetica mean":dbl)  [unwired: 1 out]
              n1060 = Reshape Array(w2515, w2514) -> (w2517:dbl[])
              n1061 = call <vilib>:"Mean.vi"("X"=w2517) -> ("mean"=→"T cinetica mean 2":dbl)  [unwired: 1 out]
            }
            frame #1 {
              n1062 = property on="P T  index" class="DigNum (strict)"() -> ("Value"=w2539:i32)  [unwired: 2 in, 2 out]
              n1063 = Increment(x=w2539) -> (x+1=w2538:i32)
              n1064 = local write "P T  index"(w2538) -> ()
            }
          }
          n1065 = Merge Signals(w2457, w2450, w2451, w2447) -> (→"P-manual":dynamicdata)
          "N" <- w2462
        }
        n1066 = case shown="True" "Save manual" {
          selector: "Save manual" -> [_ w2386]
          frame False {
          }
          frame True {
            n1067 = feedback #3() -> (w2382:dbl)  [unwired: 1 in]
            n1068 = Equal To 0?(x=w2382) -> (x = 0?=w2388:bool)
            n1069 = stacked-sequence {
              tunnel: w2388 -> [_ w2404 _]
              tunnel: [_ w2403 _] -> w2384
              frame #0 {
                w2397 = i16 3 ("precision (6)")
                n1070 = property on="T fit" class="DigNum (strict)"() -> ("Value"=w2399:dbl)  [unwired: 2 in, 2 out]
                n1071 = property on="p fit" class="DigNum (strict)"() -> ("Value"=w2400:dbl)  [unwired: 2 in, 2 out]
                n1072 = property on="termopar K" class="DigNum (strict)"() -> ("Value"=w2398:dbl)  [unwired: 2 in, 2 out]
                n1073 = Number To Fractional String(number=w2399, precision (6)=w2397) -> (F-format string=→"T string":string)  [unwired: 2 in]
                n1074 = Number To Fractional String(number=w2400, precision (6)=w2397) -> (F-format string=→"P string":string)  [unwired: 2 in]
                n1075 = Number To Fractional String(number=w2398, precision (6)=w2397) -> (F-format string=→"termopar K":string)  [unwired: 2 in]
              }
              frame #1 {
                n1076 = case shown="True" w2404 {
                  tunnel: [TRUE ("y") FALSE ("y")] -> w2403
                  frame False {
                    n1077 = property on="path" class="Path"() -> ("Value"=w2408:path)  [unwired: 2 in, 2 out]
                    n1078 = property on="P string" class="Str"() -> ("Value"=w2407:string)  [unwired: 2 in, 2 out]
                    n1079 = Concatenate Strings(w2407, "\t") -> (w2405:string)
                    n1080 = Open/Create/Replace File(file path (use dialog)=w2408, operation (0:open)=T3."open") -> (refnum out=w2412:refnum<file>, error out=w2411:errorcluster)  [unwired: 2 in, 3 out]
                    n1081 = Set File Position(refnum=w2412, from (0:start)=enum16{"start", "end", "current"}."end", error in=w2411) -> (refnum out=w2414:refnum<file>, error out=w2415:errorcluster)  [unwired: 1 in]
                    n1082 = Write to Text File(file (use dialog)=w2414, text=w2405, error in=w2415) -> (refnum out=w2410:refnum<file>, error out=w2409:errorcluster)  [unwired: 2 out]
                    n1083 = Close File(refnum=w2410, error in=w2409) -> (error out=w2417:errorcluster)  [unwired: 1 out]
                    n1084 = call <vilib>:"Simple Error Handler.vi"("error in (no error)"=w2417) -> ()  [unwired: 1 in, 8 out]
                  }
                  frame True {
                    w2420 = "\t"
                    n1085 = property on="path" class="Path"() -> ("Value"=w2427:path)  [unwired: 2 in, 2 out]
                    n1086 = property on="Count SET" class="DigNum (strict)"() -> ("Value"=w2423:i32)  [unwired: 2 in, 2 out]
                    n1087 = Open/Create/Replace File(file path (use dialog)=w2427, operation (0:open)=T3."open") -> (refnum out=w2426:refnum<file>, error out=w2425:errorcluster)  [unwired: 2 in, 3 out]
                    n1088 = Increment(x=w2423) -> (x+1=w2424:i32)
                    "Set atual" <- w2424
                    n1089 = Set File Position(refnum=w2426, from (0:start)=enum16{"start", "end", "current"}."end", error in=w2425) -> (refnum out=w2435:refnum<file>, error out=w2436:errorcluster)  [unwired: 1 in]
                    n1090 = Number To Decimal String(number=w2424) -> (decimal integer string=w2428:string)  [unwired: 1 in]
                    n1091 = property on="termopar K" class="Str"() -> ("Value"=w2419:string)  [unwired: 2 in, 2 out]
                    n1092 = property on="T string" class="Str"() -> ("Value"=w2421:string)  [unwired: 2 in, 2 out]
                    n1093 = Concatenate Strings(w2421, w2420, w2419, "\r\n", w2428, w2420) -> (w2430:string)
                    n1094 = Write to Text File(file (use dialog)=w2435, text=w2430, error in=w2436) -> (refnum out=w2433:refnum<file>, error out=w2432:errorcluster)  [unwired: 2 out]
                    n1095 = Close File(refnum=w2433, error in=w2432) -> (error out=w2438:errorcluster)  [unwired: 1 out]
                    n1096 = call <vilib>:"Simple Error Handler.vi"("error in (no error)"=w2438) -> ()  [unwired: 1 in, 8 out]
                    "T" <- TRUE ("T")
                  }
                }
              }
              frame #2 {
                n1097 = property on="path" class="Path"() -> ("Value"=w2440:path)  [unwired: 2 in, 2 out]
                n1098 = property on="Set atual" class="DigNum (strict)"() -> ("Value"=w2439:i32)  [unwired: 2 in, 2 out]
                n1099 = local write "Count SET"(w2439) -> ()
                n1100 = Read from Text File(file (use dialog)=w2440, count=-1 ("Count  3")) -> (refnum out=w2442:refnum<file>, text=w2441:string, error out=w2443:errorcluster)  [unwired: 2 in, 1 out]
                n1101 = property on="String 2" class="Str"("Value"=w2441) -> ()  [unwired: 2 in, 2 out]
                n1102 = Close File(refnum=w2442, error in=w2443) -> (error out=w2445:errorcluster)  [unwired: 1 out]
                n1103 = call <vilib>:"Simple Error Handler.vi"("error in (no error)"=w2445) -> ()  [unwired: 1 in, 8 out]
              }
            }
            n1104 = Implies(1:w2384, 2:w2386) -> (0:w2385:bool)
            n1105 = Select(t=w2382, s=w2385, f=5.0 ("t")) -> (s? t:f=w2383:dbl)
            n1106 = case shown="1" w2383 {
              frame 0, Default {
              }
              frame 1 {
                "ZPf2" <- TRUE ("ZPf2")
              }
              frame 2 {
                "Pf2" <- TRUE ("Pf2")
              }
              frame 3 {
                "Pit" <- TRUE ("Pit")
              }
              frame 4 {
                n1107 = local write "T"(FALSE ("T")) -> ()
                "ZPit" <- TRUE ("ZPit")
              }
              frame 5 {
                w2395 = FALSE
                n1108 = local write "Pit"(w2395) -> ()
                n1109 = local write "ZPf2"(w2395) -> ()
                n1110 = local write "ZPit"(w2395) -> ()
                n1111 = local write "Pf2"(w2395) -> ()
              }
            }
            n1112 = Decrement(x=w2383) -> (x-1=w2389:dbl)
            n1113 = feedback-in #3(w2389) -> ()
          }
        }
        n1114 = case shown="True" w1769 {
          tunnel: [FALSE ("Save manual") w2381] -> w1771
          tunnel: "Save manual" -> [_ w2381]
          frame False {
          }
          frame True {
          }
        }
        n1115 = case shown="True" w1769 {
          tunnel: [FALSE w1789] -> w1772
          tunnel: w1771 -> [_ w1788]
          tunnel: w1770 -> [_ w1787]
          frame False {
          }
          frame True {
            n1116 = flat-sequence {
              tunnel: w1787 -> [w1810]
              tunnel: w1788 -> [w1811]
              tunnel: [w1811] -> w1808
              tunnel: [w1810] -> w1807
              tunnel: [w1818] -> w1806
              tunnel: [w1819] -> w1805
              tunnel: [w1820] -> w1804
              tunnel: [w1821] -> w1803
              tunnel: [w1822] -> w1802
              tunnel: [w1823] -> w1801
              tunnel: [w1824] -> w1800
              tunnel: [w1826] -> w1799
              tunnel: [w1827] -> w1798
              tunnel: [w1828] -> w1797
              tunnel: [w1829] -> w1796
              tunnel: [w1830] -> w1795
              tunnel: [w1825] -> w1794
              tunnel: [w1817] -> w1793
              tunnel: [w1816] -> w1792
              tunnel: [w1815] -> w1791
              tunnel: [w1814] -> w1790
              tunnel: w1808 -> [w1813]
              tunnel: w1807 -> [w1812]
              tunnel: w1806 -> [w2328]
              tunnel: w1805 -> [w2327]
              tunnel: w1804 -> [w2326]
              tunnel: w1803 -> [w2325]
              tunnel: w1802 -> [w2324]
              tunnel: w1801 -> [w2323]
              tunnel: w1800 -> [w2322]
              tunnel: w1799 -> [w2321]
              tunnel: w1798 -> [w2320]
              tunnel: w1797 -> [w2319]
              tunnel: w1796 -> [w2318]
              tunnel: w1795 -> [w2317]
              tunnel: w1794 -> [w2316]
              tunnel: w1793 -> [w2329]
              tunnel: w1792 -> [w2330]
              tunnel: w1791 -> [w2331]
              tunnel: [w2314] -> w1789
              tunnel: w1790 -> [w2314]
              tunnel: [TRUE] -> w1786
              frame #0 {
                n1117 = local write "graph RLC"(FALSE) -> ()
              }
              frame #1 {
                n1118 = case shown="True" w1813 {
                  tunnel: [_ w1865] -> w1814
                  tunnel: w1812 -> [_ w1847]
                  tunnel: [_ w1846] -> w1815
                  tunnel: [_ w1845] -> w1816
                  tunnel: [_ w1844] -> w1817
                  tunnel: [_ w1843] -> w1818
                  tunnel: [_ w1842] -> w1819
                  tunnel: [_ w1841] -> w1820
                  tunnel: [_ w1840] -> w1821
                  tunnel: [_ w1839] -> w1822
                  tunnel: [_ w1838] -> w1823
                  tunnel: [_ w1837] -> w1824
                  tunnel: [_ w1836] -> w1825
                  tunnel: [_ w1835] -> w1826
                  tunnel: [_ w1834] -> w1827
                  tunnel: [_ w1833] -> w1828
                  tunnel: [_ w1832] -> w1829
                  tunnel: [_ w1831] -> w1830
                  frame False {
                  }
                  frame True {
                    n1119 = for {
                      N: 5 -> [_]
                      tunnel: TRUE -> [w1888]
                      tunnel: FALSE -> [w1887]
                      tunnel: [w1886] -> w1865
                      tunnel: [w1885] -> w1863 mode=indexing
                      tunnel: [w1884] -> w1862 mode=indexing
                      tunnel: [w1883] -> w1861 mode=indexing
                      tunnel: [w1882] -> w1860 mode=indexing
                      tunnel: [w1881] -> w1859 mode=indexing
                      tunnel: [w1880] -> w1858 mode=indexing
                      tunnel: [w1879] -> w1857 mode=indexing
                      tunnel: [w1878] -> w1856 mode=indexing
                      tunnel: [w1877] -> w1855 mode=indexing
                      tunnel: [w1876] -> w1854 mode=indexing
                      tunnel: [w1875] -> w1853 mode=indexing
                      tunnel: [w1874] -> w1852 mode=indexing
                      tunnel: [w1873] -> w1851 mode=indexing
                      tunnel: [w1872] -> w1850 mode=indexing
                      tunnel: [w1871] -> w1849 mode=indexing
                      tunnel: [w1870] -> w1848 mode=indexing
                      tunnel: w1847 -> [w1869]
                      n1120 = property on="path RLC_completo" class="Path"() -> ("Value"=w1868:path)  [unwired: 2 in, 2 out]
                      n1121 = stacked-sequence {
                        tunnel: w1888 -> [_ w1913 w1938 w1963 w1988 w2013 w2038 w2063 w2086 w2111 w2138 w2161 w2188 w2213 w2238 w2261 w2288 _]
                        tunnel: w1887 -> [w1889 _ _ _ _ _ _ _ _ _ _ _ _ _ _ _ _ w2312]
                        tunnel: [_ _ _ _ _ _ _ _ _ _ _ _ _ _ _ _ _ TRUE] -> w1886
                        tunnel: [_ w1912 _ _ _ _ _ _ _ _ _ _ _ _ _ _ _ _] -> w1885
                        tunnel: [_ _ w1937 _ _ _ _ _ _ _ _ _ _ _ _ _ _ _] -> w1884
                        tunnel: [_ _ _ w1962 _ _ _ _ _ _ _ _ _ _ _ _ _ _] -> w1883
                        tunnel: [_ _ _ _ w1987 _ _ _ _ _ _ _ _ _ _ _ _ _] -> w1882
                        tunnel: [_ _ _ _ _ w2012 _ _ _ _ _ _ _ _ _ _ _ _] -> w1881
                        tunnel: [_ _ _ _ _ _ w2037 _ _ _ _ _ _ _ _ _ _ _] -> w1880
                        tunnel: [_ _ _ _ _ _ _ w2062 _ _ _ _ _ _ _ _ _ _] -> w1879
                        tunnel: [_ _ _ _ _ _ _ _ w2088 _ _ _ _ _ _ _ _ _] -> w1878
                        tunnel: [_ _ _ _ _ _ _ _ _ w2113 _ _ _ _ _ _ _ _] -> w1877
                        tunnel: [_ _ _ _ _ _ _ _ _ _ w2137 _ _ _ _ _ _ _] -> w1876
                        tunnel: [_ _ _ _ _ _ _ _ _ _ _ w2163 _ _ _ _ _ _] -> w1875
                        tunnel: [_ _ _ _ _ _ _ _ _ _ _ _ w2187 _ _ _ _ _] -> w1874
                        tunnel: [_ _ _ _ _ _ _ _ _ _ _ _ _ w2212 _ _ _ _] -> w1873
                        tunnel: [_ _ _ _ _ _ _ _ _ _ _ _ _ _ w2237 _ _ _] -> w1872
                        tunnel: [_ _ _ _ _ _ _ _ _ _ _ _ _ _ _ w2263 _ _] -> w1871
                        tunnel: [_ _ _ _ _ _ _ _ _ _ _ _ _ _ _ _ w2287 _] -> w1870
                        tunnel: w1869 -> [_ w1915 w1941 w1965 w1990 w2015 w2040 w2065 w2090 w2115 w2140 w2165 w2190 w2215 w2240 w2265 w2290 _]
                        tunnel: w1868 -> [w1891 w1914 w1940 w1964 w1989 w2014 w2039 w2064 w2089 w2114 w2139 w2164 w2189 w2214 w2239 w2264 w2289 _]
                        frame #0 {
                          w1892 = "\t"
                          n1122 = local write "C-50-L"(w1889) -> ()
                          n1123 = local write "C-50-N"(w1889) -> ()
                          n1124 = local write "Z-50-L"(w1889) -> ()
                          n1125 = local write "Z-50-N"(w1889) -> ()
                          n1126 = local write "C-1K-L"(w1889) -> ()
                          n1127 = local write "C-1K-N"(w1889) -> ()
                          n1128 = local write "Z-1K-N"(w1889) -> ()
                          n1129 = local write "Z-1K-L"(w1889) -> ()
                          n1130 = local write "Z-100-L"(w1889) -> ()
                          n1131 = local write "C-10K-L"(w1889) -> ()
                          n1132 = local write "C-100-N"(w1889) -> ()
                          n1133 = local write "C-10K-N"(w1889) -> ()
                          n1134 = local write "Z-10K-N"(w1889) -> ()
                          n1135 = local write "Z-10K-L"(w1889) -> ()
                          n1136 = local write "Z-100-N"(w1889) -> ()
                          n1137 = local write "C-100-L"(w1889) -> ()
                          n1138 = Open/Create/Replace File(file path (use dialog)=w1891, operation (0:open)=T3."open") -> (refnum out=w1905:refnum<file>, error out=w1904:errorcluster)  [unwired: 2 in, 3 out]
                          n1139 = Get Date/Time String(date format (0)=enum16{"short", "long", "abbreviated"}."short", want seconds? (F)=TRUE) -> (date string=w1897:string, time string=w1896:string)  [unwired: 1 in]
                          n1140 = feedback #4() -> (w1890:dbl)  [unwired: 1 in]
                          n1141 = local write "SET 2"(w1890) -> ()
                          n1142 = Set File Position(refnum=w1905, from (0:start)=enum16{"start", "end", "current"}."end", error in=w1904) -> (refnum out=w1907:refnum<file>, error out=w1908:errorcluster)  [unwired: 1 in]
                          n1143 = Number To Fractional String(number=w1890, precision (6)=i16 2) -> (F-format string=w1895:string)  [unwired: 2 in]
                          n1144 = Add(x=w1890, y=0.2) -> (x+y=w1901:dbl)
                          n1145 = feedback-in #4(w1901) -> ()
                          n1146 = Concatenate Strings(w1895, w1892, w1897, w1892, w1896, w1892) -> (w1894:string)
                          n1147 = Write to Text File(file (use dialog)=w1907, text=w1894, error in=w1908) -> (refnum out=w1903:refnum<file>, error out=w1902:errorcluster)  [unwired: 1 in, 1 out]
                          n1148 = Close File(refnum=w1903, error in=w1902) -> (error out=w1910:errorcluster)  [unwired: 1 out]
                          n1149 = call <vilib>:"Simple Error Handler.vi"("error in (no error)"=w1910) -> ()  [unwired: 1 in, 8 out]
                        }
                        frame #1 {
                          w1916 = "\t"
                          w1933 = i16 4 ("width (-)")
                          n1150 = local write "C-50-L"(w1913) -> ()
                          n1151 = Wait (ms)(milliseconds to wait=u32 5000) -> ()  [unwired: 1 out]
                          n1152 = Open/Create/Replace File(file path (use dialog)=w1914, operation (0:open)=T3."open") -> (refnum out=w1925:refnum<file>, error out=w1924:errorcluster)  [unwired: 2 in, 3 out]
                          n1153 = Set File Position(refnum=w1925, from (0:start)=enum16{"start", "end", "current"}."end", error in=w1924) -> (refnum out=w1927:refnum<file>, error out=w1928:errorcluster)  [unwired: 1 in]
                          n1154 = call "RLC_read.vi"("Path"=w1915, "String"="cmd /c rlc_read_cAL.py") -> ("MEASURE A"=w1912:dbl, "MEASURE V [V]"=w1932:dbl, "MEASURE B"=w1911:dbl, "MEASURE I [A]"=w1931:dbl)  [unwired: 2 out]
                          n1155 = Number To Engineering String(2:w1933, 4:w1931) -> (0:w1917:string)  [unwired: 2 in]
                          n1156 = local write "MEASURE A"(w1912) -> ()
                          n1157 = local write "MEASURE B"(w1911) -> ()
                          n1158 = Number To Engineering String(2:w1933, 4:w1932) -> (0:w1918:string)  [unwired: 2 in]
                          n1159 = Number To Engineering String(2:w1933, 4:w1912) -> (0:w1920:string)  [unwired: 2 in]
                          n1160 = Number To Engineering String(2:w1933, 4:w1911) -> (0:w1919:string)  [unwired: 2 in]
                          n1161 = Concatenate Strings(w1920, w1916, w1919, w1916, w1918, w1916, w1917, w1916) -> (w1921:string)
                          n1162 = Write to Text File(file (use dialog)=w1927, text=w1921, error in=w1928) -> (refnum out=w1923:refnum<file>, error out=w1922:errorcluster)  [unwired: 1 in, 1 out]
                          n1163 = Close File(refnum=w1923, error in=w1922) -> (error out=w1930:errorcluster)  [unwired: 1 out]
                          n1164 = call <vilib>:"Simple Error Handler.vi"("error in (no error)"=w1930) -> ()  [unwired: 1 in, 8 out]
                        }
                        frame #2 {
                          w1944 = "\t"
                          w1958 = i16 4 ("width (-)")
                          n1165 = local write "C-50-N"(w1938) -> ()
                          n1166 = Wait (ms)(milliseconds to wait=u32 5000) -> ()  [unwired: 1 out]
                          n1167 = Open/Create/Replace File(file path (use dialog)=w1940, operation (0:open)=T3."open") -> (refnum out=w1952:refnum<file>, error out=w1951:errorcluster)  [unwired: 2 in, 3 out]
                          n1168 = Set File Position(refnum=w1952, from (0:start)=enum16{"start", "end", "current"}."end", error in=w1951) -> (refnum out=w1954:refnum<file>, error out=w1955:errorcluster)  [unwired: 1 in]
                          n1169 = call "RLC_read.vi"("Path"=w1941, "String"="cmd /c rlc_read_cAN.py") -> ("MEASURE A"=w1937:dbl, "MEASURE V [V]"=w1943:dbl, "MEASURE B"=w1936:dbl, "MEASURE I [A]"=w1942:dbl)  [unwired: 2 out]
                          n1170 = Number To Engineering String(2:w1958, 4:w1942) -> (0:w1945:string)  [unwired: 2 in]
                          n1171 = local write "MEASURE A 2"(w1937) -> ()
                          n1172 = local write "MEASURE B 2"(w1936) -> ()
                          n1173 = Number To Engineering String(2:w1958, 4:w1943) -> (0:w1946:string)  [unwired: 2 in]
                          n1174 = Number To Engineering String(2:w1958, 4:w1937) -> (0:w1948:string)  [unwired: 2 in]
                          n1175 = Number To Engineering String(2:w1958, 4:w1936) -> (0:w1947:string)  [unwired: 2 in]
                          n1176 = Concatenate Strings(w1948, w1944, w1947, w1944, w1946, w1944, w1945, w1944) -> (w1939:string)
                          n1177 = Write to Text File(file (use dialog)=w1954, text=w1939, error in=w1955) -> (refnum out=w1950:refnum<file>, error out=w1949:errorcluster)  [unwired: 1 in, 1 out]
                          n1178 = Close File(refnum=w1950, error in=w1949) -> (error out=w1957:errorcluster)  [unwired: 1 out]
                          n1179 = call <vilib>:"Simple Error Handler.vi"("error in (no error)"=w1957) -> ()  [unwired: 1 in, 8 out]
                        }
                        frame #3 {
                          w1968 = "\t"
                          w1983 = i16 4 ("width (-)")
                          n1180 = Wait (ms)(milliseconds to wait=u32 5000) -> ()  [unwired: 1 out]
                          n1181 = local write "C-100-L"(w1963) -> ()
                          n1182 = Open/Create/Replace File(file path (use dialog)=w1964, operation (0:open)=T3."open") -> (refnum out=w1977:refnum<file>, error out=w1976:errorcluster)  [unwired: 2 in, 3 out]
                          n1183 = Set File Position(refnum=w1977, from (0:start)=enum16{"start", "end", "current"}."end", error in=w1976) -> (refnum out=w1979:refnum<file>, error out=w1980:errorcluster)  [unwired: 1 in]
                          n1184 = call "RLC_read.vi"("Path"=w1965, "String"="cmd /c rlc_read_cBL.py") -> ("MEASURE A"=w1962:dbl, "MEASURE V [V]"=w1967:dbl, "MEASURE B"=w1961:dbl, "MEASURE I [A]"=w1966:dbl)  [unwired: 2 out]
                          n1185 = Number To Engineering String(2:w1983, 4:w1966) -> (0:w1969:string)  [unwired: 2 in]
                          n1186 = local write "MEASURE A 3"(w1962) -> ()
                          n1187 = local write "MEASURE B 3"(w1961) -> ()
                          n1188 = Number To Engineering String(2:w1983, 4:w1967) -> (0:w1970:string)  [unwired: 2 in]
                          n1189 = Number To Engineering String(2:w1983, 4:w1962) -> (0:w1972:string)  [unwired: 2 in]
                          n1190 = Number To Engineering String(2:w1983, 4:w1961) -> (0:w1971:string)  [unwired: 2 in]
                          n1191 = Concatenate Strings(w1972, w1968, w1971, w1968, w1970, w1968, w1969, w1968) -> (w1973:string)
                          n1192 = Write to Text File(file (use dialog)=w1979, text=w1973, error in=w1980) -> (refnum out=w1975:refnum<file>, error out=w1974:errorcluster)  [unwired: 1 in, 1 out]
                          n1193 = Close File(refnum=w1975, error in=w1974) -> (error out=w1982:errorcluster)  [unwired: 1 out]
                          n1194 = call <vilib>:"Simple Error Handler.vi"("error in (no error)"=w1982) -> ()  [unwired: 1 in, 8 out]
                        }
                        frame #4 {
                          w1993 = "\t"
                          w2008 = i16 4 ("width (-)")
                          n1195 = Wait (ms)(milliseconds to wait=u32 5000) -> ()  [unwired: 1 out]
                          n1196 = local write "C-100-N"(w1988) -> ()
                          n1197 = Open/Create/Replace File(file path (use dialog)=w1989, operation (0:open)=T3."open") -> (refnum out=w2002:refnum<file>, error out=w2001:errorcluster)  [unwired: 2 in, 3 out]
                          n1198 = Set File Position(refnum=w2002, from (0:start)=enum16{"start", "end", "current"}."end", error in=w2001) -> (refnum out=w2004:refnum<file>, error out=w2005:errorcluster)  [unwired: 1 in]
                          n1199 = call "RLC_read.vi"("Path"=w1990, "String"="cmd /c rlc_read_cBN.py") -> ("MEASURE A"=w1987:dbl, "MEASURE V [V]"=w1992:dbl, "MEASURE B"=w1986:dbl, "MEASURE I [A]"=w1991:dbl)  [unwired: 2 out]
                          n1200 = Number To Engineering String(2:w2008, 4:w1991) -> (0:w1994:string)  [unwired: 2 in]
                          n1201 = local write "MEASURE A 4"(w1987) -> ()
                          n1202 = local write "MEASURE B 4"(w1986) -> ()
                          n1203 = Number To Engineering String(2:w2008, 4:w1992) -> (0:w1995:string)  [unwired: 2 in]
                          n1204 = Number To Engineering String(2:w2008, 4:w1987) -> (0:w1997:string)  [unwired: 2 in]
                          n1205 = Number To Engineering String(2:w2008, 4:w1986) -> (0:w1996:string)  [unwired: 2 in]
                          n1206 = Concatenate Strings(w1997, w1993, w1996, w1993, w1995, w1993, w1994, w1993) -> (w1998:string)
                          n1207 = Write to Text File(file (use dialog)=w2004, text=w1998, error in=w2005) -> (refnum out=w2000:refnum<file>, error out=w1999:errorcluster)  [unwired: 1 in, 1 out]
                          n1208 = Close File(refnum=w2000, error in=w1999) -> (error out=w2007:errorcluster)  [unwired: 1 out]
                          n1209 = call <vilib>:"Simple Error Handler.vi"("error in (no error)"=w2007) -> ()  [unwired: 1 in, 8 out]
                        }
                        frame #5 {
                          w2033 = "\t"
                          w2018 = i16 4 ("width (-)")
                          n1210 = local write "C-1K-L"(w2013) -> ()
                          n1211 = Wait (ms)(milliseconds to wait=u32 5000) -> ()  [unwired: 1 out]
                          n1212 = Open/Create/Replace File(file path (use dialog)=w2014, operation (0:open)=T3."open") -> (refnum out=w2024:refnum<file>, error out=w2025:errorcluster)  [unwired: 2 in, 3 out]
                          n1213 = Set File Position(refnum=w2024, from (0:start)=enum16{"start", "end", "current"}."end", error in=w2025) -> (refnum out=w2022:refnum<file>, error out=w2021:errorcluster)  [unwired: 1 in]
                          n1214 = call "RLC_read.vi"("Path"=w2015, "String"="cmd /c rlc_read_cCL.py") -> ("MEASURE A"=w2012:dbl, "MEASURE V [V]"=w2017:dbl, "MEASURE B"=w2011:dbl, "MEASURE I [A]"=w2016:dbl)  [unwired: 2 out]
                          n1215 = Number To Engineering String(2:w2018, 4:w2016) -> (0:w2032:string)  [unwired: 2 in]
                          n1216 = local write "MEASURE A 5"(w2012) -> ()
                          n1217 = local write "MEASURE B 5"(w2011) -> ()
                          n1218 = Number To Engineering String(2:w2018, 4:w2017) -> (0:w2031:string)  [unwired: 2 in]
                          n1219 = Number To Engineering String(2:w2018, 4:w2012) -> (0:w2029:string)  [unwired: 2 in]
                          n1220 = Number To Engineering String(2:w2018, 4:w2011) -> (0:w2030:string)  [unwired: 2 in]
                          n1221 = Concatenate Strings(w2029, w2033, w2030, w2033, w2031, w2033, w2032, w2033) -> (w2028:string)
                          n1222 = Write to Text File(file (use dialog)=w2022, text=w2028, error in=w2021) -> (refnum out=w2026:refnum<file>, error out=w2027:errorcluster)  [unwired: 1 in, 1 out]
                          n1223 = Close File(refnum=w2026, error in=w2027) -> (error out=w2019:errorcluster)  [unwired: 1 out]
                          n1224 = call <vilib>:"Simple Error Handler.vi"("error in (no error)"=w2019) -> ()  [unwired: 1 in, 8 out]
                        }
                        frame #6 {
                          w2058 = "\t"
                          w2043 = i16 4 ("width (-)")
                          n1225 = local write "C-1K-N"(w2038) -> ()
                          n1226 = Wait (ms)(milliseconds to wait=u32 5000) -> ()  [unwired: 1 out]
                          n1227 = Open/Create/Replace File(file path (use dialog)=w2039, operation (0:open)=T3."open") -> (refnum out=w2049:refnum<file>, error out=w2050:errorcluster)  [unwired: 2 in, 3 out]
                          n1228 = Set File Position(refnum=w2049, from (0:start)=enum16{"start", "end", "current"}."end", error in=w2050) -> (refnum out=w2047:refnum<file>, error out=w2046:errorcluster)  [unwired: 1 in]
                          n1229 = call "RLC_read.vi"("Path"=w2040, "String"="cmd /c rlc_read_cCN.py") -> ("MEASURE A"=w2037:dbl, "MEASURE V [V]"=w2042:dbl, "MEASURE B"=w2036:dbl, "MEASURE I [A]"=w2041:dbl)  [unwired: 2 out]
                          n1230 = Number To Engineering String(2:w2043, 4:w2041) -> (0:w2057:string)  [unwired: 2 in]
                          n1231 = local write "MEASURE A 6"(w2037) -> ()
                          n1232 = local write "MEASURE B 6"(w2036) -> ()
                          n1233 = Number To Engineering String(2:w2043, 4:w2042) -> (0:w2056:string)  [unwired: 2 in]
                          n1234 = Number To Engineering String(2:w2043, 4:w2037) -> (0:w2054:string)  [unwired: 2 in]
                          n1235 = Number To Engineering String(2:w2043, 4:w2036) -> (0:w2055:string)  [unwired: 2 in]
                          n1236 = Concatenate Strings(w2054, w2058, w2055, w2058, w2056, w2058, w2057, w2058) -> (w2053:string)
                          n1237 = Write to Text File(file (use dialog)=w2047, text=w2053, error in=w2046) -> (refnum out=w2051:refnum<file>, error out=w2052:errorcluster)  [unwired: 1 in, 1 out]
                          n1238 = Close File(refnum=w2051, error in=w2052) -> (error out=w2044:errorcluster)  [unwired: 1 out]
                          n1239 = call <vilib>:"Simple Error Handler.vi"("error in (no error)"=w2044) -> ()  [unwired: 1 in, 8 out]
                        }
                        frame #7 {
                          w2068 = "\t"
                          w2083 = i16 4 ("width (-)")
                          n1240 = Wait (ms)(milliseconds to wait=u32 5000) -> ()  [unwired: 1 out]
                          n1241 = local write "C-10K-L"(w2063) -> ()
                          n1242 = Open/Create/Replace File(file path (use dialog)=w2064, operation (0:open)=T3."open") -> (refnum out=w2077:refnum<file>, error out=w2076:errorcluster)  [unwired: 2 in, 3 out]
                          n1243 = Set File Position(refnum=w2077, from (0:start)=enum16{"start", "end", "current"}."end", error in=w2076) -> (refnum out=w2079:refnum<file>, error out=w2080:errorcluster)  [unwired: 1 in]
                          n1244 = call "RLC_read.vi"("Path"=w2065, "String"="cmd /c rlc_read_cDL.py") -> ("MEASURE A"=w2062:dbl, "MEASURE V [V]"=w2067:dbl, "MEASURE B"=w2061:dbl, "MEASURE I [A]"=w2066:dbl)  [unwired: 2 out]
                          n1245 = Number To Engineering String(2:w2083, 4:w2066) -> (0:w2069:string)  [unwired: 2 in]
                          n1246 = local write "MEASURE A 7"(w2062) -> ()
                          n1247 = local write "MEASURE B 7"(w2061) -> ()
                          n1248 = Number To Engineering String(2:w2083, 4:w2067) -> (0:w2070:string)  [unwired: 2 in]
                          n1249 = Number To Engineering String(2:w2083, 4:w2062) -> (0:w2072:string)  [unwired: 2 in]
                          n1250 = Number To Engineering String(2:w2083, 4:w2061) -> (0:w2071:string)  [unwired: 2 in]
                          n1251 = Concatenate Strings(w2072, w2068, w2071, w2068, w2070, w2068, w2069, w2068) -> (w2073:string)
                          n1252 = Write to Text File(file (use dialog)=w2079, text=w2073, error in=w2080) -> (refnum out=w2075:refnum<file>, error out=w2074:errorcluster)  [unwired: 1 in, 1 out]
                          n1253 = Close File(refnum=w2075, error in=w2074) -> (error out=w2082:errorcluster)  [unwired: 1 out]
                          n1254 = call <vilib>:"Simple Error Handler.vi"("error in (no error)"=w2082) -> ()  [unwired: 1 in, 8 out]
                        }
                        frame #8 {
                          w2093 = "\t"
                          w2108 = i16 4 ("width (-)")
                          n1255 = Wait (ms)(milliseconds to wait=u32 5000) -> ()  [unwired: 1 out]
                          n1256 = local write "C-10K-N"(w2086) -> ()
                          n1257 = Open/Create/Replace File(file path (use dialog)=w2089, operation (0:open)=T3."open") -> (refnum out=w2102:refnum<file>, error out=w2101:errorcluster)  [unwired: 2 in, 3 out]
                          n1258 = Set File Position(refnum=w2102, from (0:start)=enum16{"start", "end", "current"}."end", error in=w2101) -> (refnum out=w2104:refnum<file>, error out=w2105:errorcluster)  [unwired: 1 in]
                          n1259 = call "RLC_read.vi"("Path"=w2090, "String"="cmd /c rlc_read_cDN.py") -> ("MEASURE A"=w2088:dbl, "MEASURE V [V]"=w2092:dbl, "MEASURE B"=w2087:dbl, "MEASURE I [A]"=w2091:dbl)  [unwired: 2 out]
                          n1260 = Number To Engineering String(2:w2108, 4:w2091) -> (0:w2094:string)  [unwired: 2 in]
                          n1261 = local write "MEASURE A 8"(w2088) -> ()
                          n1262 = local write "MEASURE B 8"(w2087) -> ()
                          n1263 = Number To Engineering String(2:w2108, 4:w2092) -> (0:w2095:string)  [unwired: 2 in]
                          n1264 = Number To Engineering String(2:w2108, 4:w2088) -> (0:w2097:string)  [unwired: 2 in]
                          n1265 = Number To Engineering String(2:w2108, 4:w2087) -> (0:w2096:string)  [unwired: 2 in]
                          n1266 = Concatenate Strings(w2097, w2093, w2096, w2093, w2095, w2093, w2094, w2093) -> (w2098:string)
                          n1267 = Write to Text File(file (use dialog)=w2104, text=w2098, error in=w2105) -> (refnum out=w2100:refnum<file>, error out=w2099:errorcluster)  [unwired: 1 in, 1 out]
                          n1268 = Close File(refnum=w2100, error in=w2099) -> (error out=w2107:errorcluster)  [unwired: 1 out]
                          n1269 = call <vilib>:"Simple Error Handler.vi"("error in (no error)"=w2107) -> ()  [unwired: 1 in, 8 out]
                        }
                        frame #9 {
                          w2118 = "\t"
                          w2133 = i16 4 ("width (-)")
                          n1270 = local write "Z-50-L"(w2111) -> ()
                          n1271 = Wait (ms)(milliseconds to wait=u32 5000) -> ()  [unwired: 1 out]
                          n1272 = Open/Create/Replace File(file path (use dialog)=w2114, operation (0:open)=T3."open") -> (refnum out=w2127:refnum<file>, error out=w2126:errorcluster)  [unwired: 2 in, 3 out]
                          n1273 = Set File Position(refnum=w2127, from (0:start)=enum16{"start", "end", "current"}."end", error in=w2126) -> (refnum out=w2129:refnum<file>, error out=w2130:errorcluster)  [unwired: 1 in]
                          n1274 = call "RLC_read.vi"("Path"=w2115, "String"="cmd /c rlc_read_ZAL.py") -> ("MEASURE A"=w2113:dbl, "MEASURE V [V]"=w2117:dbl, "MEASURE B"=w2112:dbl, "MEASURE I [A]"=w2116:dbl)  [unwired: 2 out]
                          n1275 = Number To Engineering String(2:w2133, 4:w2116) -> (0:w2119:string)  [unwired: 2 in]
                          n1276 = local write "MEASURE A 9"(w2113) -> ()
                          n1277 = local write "MEASURE B 9"(w2112) -> ()
                          n1278 = Number To Engineering String(2:w2133, 4:w2117) -> (0:w2120:string)  [unwired: 2 in]
                          n1279 = Number To Engineering String(2:w2133, 4:w2113) -> (0:w2122:string)  [unwired: 2 in]
                          n1280 = Number To Engineering String(2:w2133, 4:w2112) -> (0:w2121:string)  [unwired: 2 in]
                          n1281 = Concatenate Strings(w2122, w2118, w2121, w2118, w2120, w2118, w2119, w2118) -> (w2123:string)
                          n1282 = Write to Text File(file (use dialog)=w2129, text=w2123, error in=w2130) -> (refnum out=w2125:refnum<file>, error out=w2124:errorcluster)  [unwired: 1 in, 1 out]
                          n1283 = Close File(refnum=w2125, error in=w2124) -> (error out=w2132:errorcluster)  [unwired: 1 out]
                          n1284 = call <vilib>:"Simple Error Handler.vi"("error in (no error)"=w2132) -> ()  [unwired: 1 in, 8 out]
                        }
                        frame #10 {
                          w2143 = "\t"
                          w2158 = i16 4 ("width (-)")
                          n1285 = local write "Z-50-N"(w2138) -> ()
                          n1286 = Wait (ms)(milliseconds to wait=u32 5000) -> ()  [unwired: 1 out]
                          n1287 = Open/Create/Replace File(file path (use dialog)=w2139, operation (0:open)=T3."open") -> (refnum out=w2152:refnum<file>, error out=w2151:errorcluster)  [unwired: 2 in, 3 out]
                          n1288 = Set File Position(refnum=w2152, from (0:start)=enum16{"start", "end", "current"}."end", error in=w2151) -> (refnum out=w2154:refnum<file>, error out=w2155:errorcluster)  [unwired: 1 in]
                          n1289 = call "RLC_read.vi"("Path"=w2140, "String"="cmd /c rlc_read_ZAN.py") -> ("MEASURE A"=w2137:dbl, "MEASURE V [V]"=w2142:dbl, "MEASURE B"=w2136:dbl, "MEASURE I [A]"=w2141:dbl)  [unwired: 2 out]
                          n1290 = Number To Engineering String(2:w2158, 4:w2141) -> (0:w2144:string)  [unwired: 2 in]
                          n1291 = local write "MEASURE A 10"(w2137) -> ()
                          n1292 = local write "MEASURE B 10"(w2136) -> ()
                          n1293 = Number To Engineering String(2:w2158, 4:w2142) -> (0:w2145:string)  [unwired: 2 in]
                          n1294 = Number To Engineering String(2:w2158, 4:w2137) -> (0:w2147:string)  [unwired: 2 in]
                          n1295 = Number To Engineering String(2:w2158, 4:w2136) -> (0:w2146:string)  [unwired: 2 in]
                          n1296 = Concatenate Strings(w2147, w2143, w2146, w2143, w2145, w2143, w2144, w2143) -> (w2148:string)
                          n1297 = Write to Text File(file (use dialog)=w2154, text=w2148, error in=w2155) -> (refnum out=w2150:refnum<file>, error out=w2149:errorcluster)  [unwired: 1 in, 1 out]
                          n1298 = Close File(refnum=w2150, error in=w2149) -> (error out=w2157:errorcluster)  [unwired: 1 out]
                          n1299 = call <vilib>:"Simple Error Handler.vi"("error in (no error)"=w2157) -> ()  [unwired: 1 in, 8 out]
                        }
                        frame #11 {
                          w2168 = "\t"
                          w2183 = i16 4 ("width (-)")
                          n1300 = Wait (ms)(milliseconds to wait=u32 5000) -> ()  [unwired: 1 out]
                          n1301 = local write "Z-100-L"(w2161) -> ()
                          n1302 = Open/Create/Replace File(file path (use dialog)=w2164, operation (0:open)=T3."open") -> (refnum out=w2177:refnum<file>, error out=w2176:errorcluster)  [unwired: 2 in, 3 out]
                          n1303 = Set File Position(refnum=w2177, from (0:start)=enum16{"start", "end", "current"}."end", error in=w2176) -> (refnum out=w2179:refnum<file>, error out=w2180:errorcluster)  [unwired: 1 in]
                          n1304 = call "RLC_read.vi"("Path"=w2165, "String"="cmd /c rlc_read_ZBL.py") -> ("MEASURE A"=w2163:dbl, "MEASURE V [V]"=w2167:dbl, "MEASURE B"=w2162:dbl, "MEASURE I [A]"=w2166:dbl)  [unwired: 2 out]
                          n1305 = Number To Engineering String(2:w2183, 4:w2166) -> (0:w2169:string)  [unwired: 2 in]
                          n1306 = local write "MEASURE A 11"(w2163) -> ()
                          n1307 = local write "MEASURE B 11"(w2162) -> ()
                          n1308 = Number To Engineering String(2:w2183, 4:w2167) -> (0:w2170:string)  [unwired: 2 in]
                          n1309 = Number To Engineering String(2:w2183, 4:w2163) -> (0:w2172:string)  [unwired: 2 in]
                          n1310 = Number To Engineering String(2:w2183, 4:w2162) -> (0:w2171:string)  [unwired: 2 in]
                          n1311 = Concatenate Strings(w2172, w2168, w2171, w2168, w2170, w2168, w2169, w2168) -> (w2173:string)
                          n1312 = Write to Text File(file (use dialog)=w2179, text=w2173, error in=w2180) -> (refnum out=w2175:refnum<file>, error out=w2174:errorcluster)  [unwired: 1 in, 1 out]
                          n1313 = Close File(refnum=w2175, error in=w2174) -> (error out=w2182:errorcluster)  [unwired: 1 out]
                          n1314 = call <vilib>:"Simple Error Handler.vi"("error in (no error)"=w2182) -> ()  [unwired: 1 in, 8 out]
                        }
                        frame #12 {
                          w2193 = "\t"
                          w2208 = i16 4 ("width (-)")
                          n1315 = Wait (ms)(milliseconds to wait=u32 5000) -> ()  [unwired: 1 out]
                          n1316 = local write "Z-100-N"(w2188) -> ()
                          n1317 = Open/Create/Replace File(file path (use dialog)=w2189, operation (0:open)=T3."open") -> (refnum out=w2202:refnum<file>, error out=w2201:errorcluster)  [unwired: 2 in, 3 out]
                          n1318 = Set File Position(refnum=w2202, from (0:start)=enum16{"start", "end", "current"}."end", error in=w2201) -> (refnum out=w2204:refnum<file>, error out=w2205:errorcluster)  [unwired: 1 in]
                          n1319 = call "RLC_read.vi"("Path"=w2190, "String"="cmd /c rlc_read_ZBN.py") -> ("MEASURE A"=w2187:dbl, "MEASURE V [V]"=w2192:dbl, "MEASURE B"=w2186:dbl, "MEASURE I [A]"=w2191:dbl)  [unwired: 2 out]
                          n1320 = Number To Engineering String(2:w2208, 4:w2191) -> (0:w2194:string)  [unwired: 2 in]
                          n1321 = local write "MEASURE A 12"(w2187) -> ()
                          n1322 = local write "MEASURE B 12"(w2186) -> ()
                          n1323 = Number To Engineering String(2:w2208, 4:w2192) -> (0:w2195:string)  [unwired: 2 in]
                          n1324 = Number To Engineering String(2:w2208, 4:w2187) -> (0:w2197:string)  [unwired: 2 in]
                          n1325 = Number To Engineering String(2:w2208, 4:w2186) -> (0:w2196:string)  [unwired: 2 in]
                          n1326 = Concatenate Strings(w2197, w2193, w2196, w2193, w2195, w2193, w2194, w2193) -> (w2198:string)
                          n1327 = Write to Text File(file (use dialog)=w2204, text=w2198, error in=w2205) -> (refnum out=w2200:refnum<file>, error out=w2199:errorcluster)  [unwired: 1 in, 1 out]
                          n1328 = Close File(refnum=w2200, error in=w2199) -> (error out=w2207:errorcluster)  [unwired: 1 out]
                          n1329 = call <vilib>:"Simple Error Handler.vi"("error in (no error)"=w2207) -> ()  [unwired: 1 in, 8 out]
                        }
                        frame #13 {
                          w2218 = "\t"
                          w2233 = i16 4 ("width (-)")
                          n1330 = local write "Z-1K-L"(w2213) -> ()
                          n1331 = Wait (ms)(milliseconds to wait=u32 5000) -> ()  [unwired: 1 out]
                          n1332 = Open/Create/Replace File(file path (use dialog)=w2214, operation (0:open)=T3."open") -> (refnum out=w2227:refnum<file>, error out=w2226:errorcluster)  [unwired: 2 in, 3 out]
                          n1333 = Set File Position(refnum=w2227, from (0:start)=enum16{"start", "end", "current"}."end", error in=w2226) -> (refnum out=w2229:refnum<file>, error out=w2230:errorcluster)  [unwired: 1 in]
                          n1334 = call "RLC_read.vi"("Path"=w2215, "String"="cmd /c rlc_read_ZCL.py") -> ("MEASURE A"=w2212:dbl, "MEASURE V [V]"=w2217:dbl, "MEASURE B"=w2211:dbl, "MEASURE I [A]"=w2216:dbl)  [unwired: 2 out]
                          n1335 = Number To Engineering String(2:w2233, 4:w2216) -> (0:w2219:string)  [unwired: 2 in]
                          n1336 = local write "MEASURE A 13"(w2212) -> ()
                          n1337 = local write "MEASURE B 13"(w2211) -> ()
                          n1338 = Number To Engineering String(2:w2233, 4:w2217) -> (0:w2220:string)  [unwired: 2 in]
                          n1339 = Number To Engineering String(2:w2233, 4:w2212) -> (0:w2222:string)  [unwired: 2 in]
                          n1340 = Number To Engineering String(2:w2233, 4:w2211) -> (0:w2221:string)  [unwired: 2 in]
                          n1341 = Concatenate Strings(w2222, w2218, w2221, w2218, w2220, w2218, w2219, w2218) -> (w2223:string)
                          n1342 = Write to Text File(file (use dialog)=w2229, text=w2223, error in=w2230) -> (refnum out=w2225:refnum<file>, error out=w2224:errorcluster)  [unwired: 1 in, 1 out]
                          n1343 = Close File(refnum=w2225, error in=w2224) -> (error out=w2232:errorcluster)  [unwired: 1 out]
                          n1344 = call <vilib>:"Simple Error Handler.vi"("error in (no error)"=w2232) -> ()  [unwired: 1 in, 8 out]
                        }
                        frame #14 {
                          w2243 = "\t"
                          w2258 = i16 4 ("width (-)")
                          n1345 = local write "Z-1K-N"(w2238) -> ()
                          n1346 = Wait (ms)(milliseconds to wait=u32 5000) -> ()  [unwired: 1 out]
                          n1347 = Open/Create/Replace File(file path (use dialog)=w2239, operation (0:open)=T3."open") -> (refnum out=w2252:refnum<file>, error out=w2251:errorcluster)  [unwired: 2 in, 3 out]
                          n1348 = Set File Position(refnum=w2252, from (0:start)=enum16{"start", "end", "current"}."end", error in=w2251) -> (refnum out=w2254:refnum<file>, error out=w2255:errorcluster)  [unwired: 1 in]
                          n1349 = call "RLC_read.vi"("Path"=w2240, "String"="cmd /c rlc_read_ZCN.py") -> ("MEASURE A"=w2237:dbl, "MEASURE V [V]"=w2242:dbl, "MEASURE B"=w2236:dbl, "MEASURE I [A]"=w2241:dbl)  [unwired: 2 out]
                          n1350 = Number To Engineering String(2:w2258, 4:w2241) -> (0:w2244:string)  [unwired: 2 in]
                          n1351 = local write "MEASURE A 14"(w2237) -> ()
                          n1352 = local write "MEASURE B 14"(w2236) -> ()
                          n1353 = Number To Engineering String(2:w2258, 4:w2242) -> (0:w2245:string)  [unwired: 2 in]
                          n1354 = Number To Engineering String(2:w2258, 4:w2237) -> (0:w2247:string)  [unwired: 2 in]
                          n1355 = Number To Engineering String(2:w2258, 4:w2236) -> (0:w2246:string)  [unwired: 2 in]
                          n1356 = Concatenate Strings(w2247, w2243, w2246, w2243, w2245, w2243, w2244, w2243) -> (w2248:string)
                          n1357 = Write to Text File(file (use dialog)=w2254, text=w2248, error in=w2255) -> (refnum out=w2250:refnum<file>, error out=w2249:errorcluster)  [unwired: 1 in, 1 out]
                          n1358 = Close File(refnum=w2250, error in=w2249) -> (error out=w2257:errorcluster)  [unwired: 1 out]
                          n1359 = call <vilib>:"Simple Error Handler.vi"("error in (no error)"=w2257) -> ()  [unwired: 1 in, 8 out]
                        }
                        frame #15 {
                          w2268 = "\t"
                          w2283 = i16 4 ("width (-)")
                          n1360 = Wait (ms)(milliseconds to wait=u32 5000) -> ()  [unwired: 1 out]
                          n1361 = local write "Z-10K-L"(w2261) -> ()
                          n1362 = Open/Create/Replace File(file path (use dialog)=w2264, operation (0:open)=T3."open") -> (refnum out=w2277:refnum<file>, error out=w2276:errorcluster)  [unwired: 2 in, 3 out]
                          n1363 = Set File Position(refnum=w2277, from (0:start)=enum16{"start", "end", "current"}."end", error in=w2276) -> (refnum out=w2279:refnum<file>, error out=w2280:errorcluster)  [unwired: 1 in]
                          n1364 = call "RLC_read.vi"("Path"=w2265, "String"="cmd /c rlc_read_ZDL.py") -> ("MEASURE A"=w2263:dbl, "MEASURE V [V]"=w2267:dbl, "MEASURE B"=w2262:dbl, "MEASURE I [A]"=w2266:dbl)  [unwired: 2 out]
                          n1365 = Number To Engineering String(2:w2283, 4:w2266) -> (0:w2269:string)  [unwired: 2 in]
                          n1366 = local write "MEASURE A 15"(w2263) -> ()
                          n1367 = local write "MEASURE B 15"(w2262) -> ()
                          n1368 = Number To Engineering String(2:w2283, 4:w2267) -> (0:w2270:string)  [unwired: 2 in]
                          n1369 = Number To Engineering String(2:w2283, 4:w2263) -> (0:w2272:string)  [unwired: 2 in]
                          n1370 = Number To Engineering String(2:w2283, 4:w2262) -> (0:w2271:string)  [unwired: 2 in]
                          n1371 = Concatenate Strings(w2272, w2268, w2271, w2268, w2270, w2268, w2269, w2268) -> (w2273:string)
                          n1372 = Write to Text File(file (use dialog)=w2279, text=w2273, error in=w2280) -> (refnum out=w2275:refnum<file>, error out=w2274:errorcluster)  [unwired: 1 in, 1 out]
                          n1373 = Close File(refnum=w2275, error in=w2274) -> (error out=w2282:errorcluster)  [unwired: 1 out]
                          n1374 = call <vilib>:"Simple Error Handler.vi"("error in (no error)"=w2282) -> ()  [unwired: 1 in, 8 out]
                        }
                        frame #16 {
                          w2294 = "\t"
                          w2309 = i16 4 ("width (-)")
                          n1375 = Wait (ms)(milliseconds to wait=u32 5000) -> ()  [unwired: 1 out]
                          n1376 = local write "Z-10K-N"(w2288) -> ()
                          n1377 = Open/Create/Replace File(file path (use dialog)=w2289, operation (0:open)=T3."open") -> (refnum out=w2303:refnum<file>, error out=w2302:errorcluster)  [unwired: 2 in, 3 out]
                          n1378 = Set File Position(refnum=w2303, from (0:start)=enum16{"start", "end", "current"}."end", error in=w2302) -> (refnum out=w2305:refnum<file>, error out=w2306:errorcluster)  [unwired: 1 in]
                          n1379 = call "RLC_read.vi"("Path"=w2290, "String"="cmd /c rlc_read_ZDN.py") -> ("MEASURE A"=w2287:dbl, "MEASURE V [V]"=w2293:dbl, "MEASURE B"=w2286:dbl, "MEASURE I [A]"=w2292:dbl)  [unwired: 2 out]
                          n1380 = Number To Engineering String(2:w2309, 4:w2292) -> (0:w2295:string)  [unwired: 2 in]
                          n1381 = local write "MEASURE A 16"(w2287) -> ()
                          n1382 = local write "MEASURE B 16"(w2286) -> ()
                          n1383 = Number To Engineering String(2:w2309, 4:w2293) -> (0:w2296:string)  [unwired: 2 in]
                          n1384 = Number To Engineering String(2:w2309, 4:w2287) -> (0:w2298:string)  [unwired: 2 in]
                          n1385 = Number To Engineering String(2:w2309, 4:w2286) -> (0:w2297:string)  [unwired: 2 in]
                          n1386 = Concatenate Strings(w2298, w2294, w2297, w2294, w2296, w2294, w2295, w2294, "\r\n") -> (w2299:string)
                          n1387 = Write to Text File(file (use dialog)=w2305, text=w2299, error in=w2306) -> (refnum out=w2301:refnum<file>, error out=w2300:errorcluster)  [unwired: 1 in, 1 out]
                          n1388 = Close File(refnum=w2301, error in=w2300) -> (error out=w2308:errorcluster)  [unwired: 1 out]
                          n1389 = call <vilib>:"Simple Error Handler.vi"("error in (no error)"=w2308) -> ()  [unwired: 1 in, 8 out]
                        }
                        frame #17 {
                          n1390 = local write "Z-50-N"(w2312) -> ()
                          n1391 = local write "Z-50-L"(w2312) -> ()
                          n1392 = local write "C-1K-N"(w2312) -> ()
                          n1393 = local write "C-50-N"(w2312) -> ()
                          n1394 = local write "C-50-L"(w2312) -> ()
                          n1395 = local write "Z-1K-N"(w2312) -> ()
                          n1396 = local write "C-1K-L"(w2312) -> ()
                          n1397 = local write "Z-1K-L"(w2312) -> ()
                          n1398 = local write "Z-100-L"(w2312) -> ()
                          n1399 = local write "C-10K-L"(w2312) -> ()
                          n1400 = local write "Z-10K-L"(w2312) -> ()
                          n1401 = local write "C-10K-N"(w2312) -> ()
                          n1402 = local write "Z-10K-N"(w2312) -> ()
                          n1403 = local write "C-100-N"(w2312) -> ()
                          n1404 = local write "C-100-L"(w2312) -> ()
                          n1405 = local write "Z-100-N"(w2312) -> ()
                        }
                      }
                    }
                    n1406 = call <vilib>:"Mean.vi"("X"=w1863) -> ("mean"=w1846:dbl)  [unwired: 1 out]
                    n1407 = call <vilib>:"Mean.vi"("X"=w1862) -> ("mean"=w1845:dbl)  [unwired: 1 out]
                    n1408 = call <vilib>:"Mean.vi"("X"=w1861) -> ("mean"=w1844:dbl)  [unwired: 1 out]
                    n1409 = call <vilib>:"Mean.vi"("X"=w1860) -> ("mean"=w1843:dbl)  [unwired: 1 out]
                    n1410 = call <vilib>:"Mean.vi"("X"=w1859) -> ("mean"=w1842:dbl)  [unwired: 1 out]
                    n1411 = call <vilib>:"Mean.vi"("X"=w1858) -> ("mean"=w1841:dbl)  [unwired: 1 out]
                    n1412 = call <vilib>:"Mean.vi"("X"=w1857) -> ("mean"=w1840:dbl)  [unwired: 1 out]
                    n1413 = call <vilib>:"Mean.vi"("X"=w1856) -> ("mean"=w1839:dbl)  [unwired: 1 out]
                    n1414 = call <vilib>:"Mean.vi"("X"=w1855) -> ("mean"=w1838:dbl)  [unwired: 1 out]
                    n1415 = call <vilib>:"Mean.vi"("X"=w1854) -> ("mean"=w1837:dbl)  [unwired: 1 out]
                    n1416 = call <vilib>:"Mean.vi"("X"=w1853) -> ("mean"=w1836:dbl)  [unwired: 1 out]
                    n1417 = call <vilib>:"Mean.vi"("X"=w1852) -> ("mean"=w1835:dbl)  [unwired: 1 out]
                    n1418 = call <vilib>:"Mean.vi"("X"=w1851) -> ("mean"=w1834:dbl)  [unwired: 1 out]
                    n1419 = call <vilib>:"Mean.vi"("X"=w1850) -> ("mean"=w1833:dbl)  [unwired: 1 out]
                    n1420 = call <vilib>:"Mean.vi"("X"=w1849) -> ("mean"=w1832:dbl)  [unwired: 1 out]
                    n1421 = call <vilib>:"Mean.vi"("X"=w1848) -> ("mean"=w1831:dbl)  [unwired: 1 out]
                    n1422 = local write "mean"(w1846) -> ()
                    n1423 = local write "mean 2"(w1845) -> ()
                    n1424 = local write "mean 3"(w1844) -> ()
                    n1425 = local write "mean 4"(w1843) -> ()
                    n1426 = local write "mean 5"(w1842) -> ()
                    n1427 = local write "mean 6"(w1841) -> ()
                    n1428 = local write "mean 7"(w1840) -> ()
                    n1429 = local write "mean 8"(w1839) -> ()
                    n1430 = local write "mean 9"(w1838) -> ()
                    n1431 = local write "mean 10"(w1837) -> ()
                    n1432 = local write "mean 11"(w1836) -> ()
                    n1433 = local write "mean 12"(w1835) -> ()
                    n1434 = local write "mean 13"(w1834) -> ()
                    n1435 = local write "mean 14"(w1833) -> ()
                    n1436 = local write "mean 15"(w1832) -> ()
                    n1437 = local write "mean 16"(w1831) -> ()
                  }
                }
              }
              frame #2 {
                n1438 = case shown="True" w2314 {
                  tunnel: w2331 -> [_ w2347]
                  tunnel: w2330 -> [_ w2346]
                  tunnel: w2329 -> [_ w2345]
                  tunnel: w2328 -> [_ w2344]
                  tunnel: w2327 -> [_ w2343]
                  tunnel: w2326 -> [_ w2342]
                  tunnel: w2325 -> [_ w2341]
                  tunnel: w2324 -> [_ w2340]
                  tunnel: w2323 -> [_ w2339]
                  tunnel: w2322 -> [_ w2338]
                  tunnel: w2321 -> [_ w2337]
                  tunnel: w2320 -> [_ w2336]
                  tunnel: w2319 -> [_ w2335]
                  tunnel: w2318 -> [_ w2334]
                  tunnel: w2317 -> [_ w2333]
                  tunnel: w2316 -> [_ w2332]
                  frame False {
                  }
                  frame True {
                    w2362 = "\t"
                    w2379 = i16 4 ("precision (6)")
                    n1439 = property on="SET" class="DigNum (strict)"() -> ("Value"=w2348:i32)  [unwired: 2 in, 2 out]
                    n1440 = Number To Engineering String(2:w2379, 4:w2347) -> (0:w2377:string)  [unwired: 2 in]
                    n1441 = Number To Engineering String(2:w2379, 4:w2346) -> (0:w2376:string)  [unwired: 2 in]
                    n1442 = Number To Engineering String(2:w2379, 4:w2345) -> (0:w2375:string)  [unwired: 2 in]
                    n1443 = Number To Engineering String(2:w2379, 4:w2344) -> (0:w2374:string)  [unwired: 2 in]
                    n1444 = Number To Engineering String(2:w2379, 4:w2343) -> (0:w2373:string)  [unwired: 2 in]
                    n1445 = Number To Engineering String(2:w2379, 4:w2342) -> (0:w2372:string)  [unwired: 2 in]
                    n1446 = Number To Engineering String(2:w2379, 4:w2341) -> (0:w2371:string)  [unwired: 2 in]
                    n1447 = Number To Engineering String(2:w2379, 4:w2340) -> (0:w2370:string)  [unwired: 2 in]
                    n1448 = Number To Engineering String(2:w2379, 4:w2339) -> (0:w2369:string)  [unwired: 2 in]
                    n1449 = Number To Engineering String(2:w2379, 4:w2338) -> (0:w2368:string)  [unwired: 2 in]
                    n1450 = Number To Engineering String(2:w2379, 4:w2332) -> (0:w2367:string)  [unwired: 2 in]
                    n1451 = Number To Engineering String(2:w2379, 4:w2337) -> (0:w2366:string)  [unwired: 2 in]
                    n1452 = Number To Engineering String(2:w2379, 4:w2336) -> (0:w2365:string)  [unwired: 2 in]
                    n1453 = Number To Engineering String(2:w2379, 4:w2335) -> (0:w2364:string)  [unwired: 2 in]
                    n1454 = Number To Engineering String(2:w2379, 4:w2334) -> (0:w2363:string)  [unwired: 2 in]
                    n1455 = Number To Engineering String(2:w2379, 4:w2333) -> (0:w2361:string)  [unwired: 2 in]
                    n1456 = Number To Decimal String(number=w2348) -> (decimal integer string=w2378:string)  [unwired: 1 in]
                    n1457 = property on="path RLC_mean" class="Path"() -> ("Value"=w2349:path)  [unwired: 2 in, 2 out]
                    n1458 = Open/Create/Replace File(file path (use dialog)=w2349, operation (0:open)=T3."open") -> (refnum out=w2354:refnum<file>, error out=w2353:errorcluster)  [unwired: 2 in, 3 out]
                    n1459 = Concatenate Strings(w2378, w2362, w2377, w2362, w2376, w2362, w2375, w2362, w2374, w2362, w2373, w2362, w2372, w2362, w2371, w2362, w2370, w2362, w2369, w2362, w2368, w2362, w2367, w2362, w2366, w2362, w2365, w2362, w2364, w2362, w2363, w2362, w2361, "\r\n") -> (w2350:string)
                    n1460 = Set File Position(refnum=w2354, from (0:start)=enum16{"start", "end", "current"}."end", error in=w2353) -> (refnum out=w2356:refnum<file>, error out=w2357:errorcluster)  [unwired: 1 in]
                    n1461 = Write to Text File(file (use dialog)=w2356, text=w2350, error in=w2357) -> (refnum out=w2352:refnum<file>, error out=w2351:errorcluster)  [unwired: 1 in, 1 out]
                    n1462 = Close File(refnum=w2352, error in=w2351) -> (error out=w2359:errorcluster)  [unwired: 1 out]
                    n1463 = call <vilib>:"Simple Error Handler.vi"("error in (no error)"=w2359) -> ()  [unwired: 1 in, 8 out]
                  }
                }
              }
            }
            n1464 = local write "graph RLC"(w1786) -> ()
          }
        }
        n1465 = call <vilib>:"Linear Fit.vi"("Y"=w1759, "X"=w1763) -> ("Best Linear Fit"=w1761:dbl[], "slope"=→"bar/N":dbl)  [unwired: 9 in, 3 out]
        n1466 = Bundle(w1763, w1759) -> (w1766:cluster{i32[], dbl[]})  [unwired: 1 in]
        n1467 = call <vilib>:"General Polynomial Fit.vi"("Y"=w1768, "polynomial order"=w1784, "X"=w1763) -> ("Best Polynomial Fit"=w1780:dbl[], "Polynomial Coefficients"=w1781:dbl[])  [unwired: 9 in, 2 out]
        "Polynomial Coefficients 2" <- w1781
        n1468 = call <vilib>:"General Polynomial Fit.vi"("Y"=w1759, "polynomial order"=w1784, "X"=w1777) -> ("Best Polynomial Fit"=w1762:dbl[], "Polynomial Coefficients"=w1775:dbl[])  [unwired: 9 in, 2 out]
        "Polynomial Coefficients" <- w1775
        n1469 = Bundle(w1763, "Best Polynomial Fit"=w1762) -> (w1765:cluster{i32[], "Best Polynomial Fit":dbl[]})  [unwired: 1 in]
        n1470 = Build Array(w1768, w1780) -> (→"Linear Model Graph 2":dbl[][])
        n1471 = Index Array(array=w1775, index=0) -> (element=→"p fit":dbl)
        n1472 = Index Array(array=w1781, index=0) -> (element=→"T fit":dbl)
        n1473 = Build Array(w1759, w1762, w1761) -> (→"Linear Model Graph":dbl[][])
        n1474 = Bundle(w1763, "Best Linear Fit"=w1761) -> (w1764:cluster{i32[], "Best Linear Fit":dbl[]})  [unwired: 1 in]
        n1475 = Build Array(w1766, w1765, w1764) -> ()  [unwired: 1 out]
      }
    }
    n1476 = case shown="True" "Close RLC 2" {
      tunnel: w36 -> [_ w166]
      frame False {
      }
      frame True {
        n1477 = call "RLC_close.vi"("Path"=w166) -> ("String"=w167:string)  [unwired: 10 in]
        n1478 = local write "RLC300 - digimess"(w167) -> ()
      }
    }
    n1479 = case shown="True" "Open Button 2" {
      frame False {
      }
      frame True {
        n1480 = property on="Sample name" class="Str"() -> ("Value"=w1738:string)  [unwired: 2 in, 2 out]
        n1481 = property on="File name" class="Str"() -> ("Value"=w1739:string)  [unwired: 2 in, 2 out]
        n1482 = property on="Nota" class="Str"() -> ("Value"=w1737:string)  [unwired: 2 in, 2 out]
        n1483 = call "Open file.vi"("Nota 01"=w1737, "Sample name"=w1738, "File name"=w1739) -> ("path open old"=w1736:path)  [unwired: 8 in]
        n1484 = local write "path"(w1736) -> ()
      }
    }
    n1485 = case shown="True" "Refresh Button 2" {
      frame False {
      }
      frame True {
        n1486 = property on="Waveform Chart" class="WFChart (strict)"("History Data"=dynamicdata[] []) -> ()  [unwired: 2 in, 2 out]
      }
    }
    n1487 = case shown="True" "Open Button" {
      frame False {
      }
      frame True {
        n1488 = flat-sequence {
          tunnel: ["Sample name"] -> w1742
          tunnel: ["Nota"] -> w1741
          tunnel: [w1744] -> w1740
          tunnel: w1742 -> [w1757]
          tunnel: w1741 -> [w1756]
          tunnel: w1740 -> [w1751]
          frame #0 {
            n1489 = local write "Count SET"(0 ("Count SET")) -> ()
            n1490 = local write "Set atual"(0 ("Count  3")) -> ()
            n1491 = call "File_data_new.vi"("Nota 01"="Nota", "Sample name"="Sample name", "File name"="File name") -> ("path"=w1744:path)  [unwired: 8 in]
            "path" <- w1744
          }
          frame #1 {
            w1752 = FALSE
            n1492 = Strip Path(path=w1751) -> (stripped path=w1750:path, name=w1749:string)
            n1493 = local write "Pf2"(w1752) -> ()
            n1494 = local write "ZPit"(w1752) -> ()
            n1495 = local write "Pit"(w1752) -> ()
            n1496 = local write "ZPf2"(w1752) -> ()
            n1497 = local write "T"(w1752) -> ()
            n1498 = Concatenate Strings(w1749, "_cinetica" ("string")) -> (w1754:string)
            n1499 = call "File_data_cinetica.vi"("path in"=w1750, "Nota 01"=w1756, "Sample name"=w1757, "File name"=w1754) -> ("path"=→"path 2_cinetica":path)  [unwired: 7 in]
          }
        }
      }
    }
    n1500 = local write "Manual Ctrl"(w49) -> ()
    n1501 = Or(x=w39, y=w38) -> (x .or. y?=w40:bool)
    n1502 = Or(x=w40, y="Refresh Button") -> (x .or. y?=w42:bool)
    n1503 = case shown="True" w42 {
      frame False {
      }
      frame True {
        n1504 = stacked-sequence {
          frame #0 {
            n1505 = property on="Waveform Chart P 2" class="WFChart (strict)"("History Data"=dbl[][] []) -> ()  [unwired: 2 in, 2 out]
          }
          frame #1 {
            n1506 = property on="path RLC_mean" class="Path"() -> ("Value"=w72:path)  [unwired: 2 in, 2 out]
            n1507 = Open/Create/Replace File(file path (use dialog)=w72, operation (0:open)=T3."open", access (0:read/write)=enum16{"read/write", "read-only", "write-only"}."read-only") -> (refnum out=w76:refnum<file>, error out=w75:errorcluster)  [unwired: 3 in, 1 out]
            n1508 = Read from Text File(file (use dialog)=w76, error in=w75) -> (refnum out=w81:refnum<file>, text=w77:string, error out=w80:errorcluster)  [unwired: 2 in, 1 out]
            n1509 = Close File(refnum=w81, error in=w80) -> ()  [unwired: 2 out]
            n1510 = Search/Split String(string=w77, search string/char (-)="SET\tDATE\tTIME\t\tP (BAR)\tT (ºC)\tC-50-L\tC-50-N\tC-100-L\tC-100-N\tC-1K-L\tC-1K-N\tC-10K-L\tC-10K-N\tZ-50-L\tZ-50-N\tZ-100-L\tZ-100-N\tZ-1K-L\tZ-1K-N\tZ-10K-L\tZ-10K-N") -> (match + rest of string=w82:string)  [unwired: 1 in, 2 out]
            n1511 = String Subset(string=w82, offset (0)=150) -> (substring=w89:string)  [unwired: 1 in]
            n1512 = Spreadsheet String To Array(format string="%#g", spreadsheet string=w89) -> (array=w88:dbl[][])  [unwired: 2 in]
            n1513 = Transpose Matrix(1:w88) -> (0:w102:dbl[][])
            n1514 = Index Array(array=w102, index (row)=1 ("index (row) 4")) -> (element=w103:dbl[])  [unwired: 1 in]
            n1515 = Index Array(array=w102, index (row)=2 ("index (row) 5")) -> (element=w104:dbl[])  [unwired: 1 in]
            n1516 = Index Array(array=w102, index (row)=3 ("index (row) 2")) -> (element=w105:dbl[])  [unwired: 1 in]
            n1517 = Index Array(array=w102, index (row)=4 ("index (row) 3")) -> (element=w106:dbl[])  [unwired: 1 in]
            n1518 = Index Array(array=w102, index (row)=5 ("index (row) 4")) -> (element=w107:dbl[])  [unwired: 1 in]
            n1519 = Index Array(array=w102, index (row)=6 ("index (row) 5")) -> (element=w108:dbl[])  [unwired: 1 in]
            n1520 = Index Array(array=w102, index (row)=7 ("index (row) 2")) -> (element=w109:dbl[])  [unwired: 1 in]
            n1521 = Index Array(array=w102, index (row)=8 ("index (row) 3")) -> (element=w110:dbl[])  [unwired: 1 in]
            n1522 = Index Array(array=w102, index (row)=9 ("index (row) 4")) -> (element=w71:dbl[])  [unwired: 1 in]
            n1523 = Index Array(array=w102, index (row)=10 ("index (row) 5")) -> (element=w70:dbl[])  [unwired: 1 in]
            n1524 = Index Array(array=w102, index (row)=11 ("index (row) 2")) -> (element=w69:dbl[])  [unwired: 1 in]
            n1525 = Index Array(array=w102, index (row)=12 ("index (row) 3")) -> (element=w68:dbl[])  [unwired: 1 in]
            n1526 = Index Array(array=w102, index (row)=13 ("index (row) 4")) -> (element=w67:dbl[])  [unwired: 1 in]
            n1527 = Index Array(array=w102, index (row)=14 ("index (row) 5")) -> (element=w66:dbl[])  [unwired: 1 in]
            n1528 = Index Array(array=w102, index (row)=15 ("index (row) 2")) -> (element=w65:dbl[])  [unwired: 1 in]
            n1529 = Index Array(array=w102, index (row)=16 ("index (row) 3")) -> (element=w64:dbl[])  [unwired: 1 in]
            n1530 = Build Array(w103, w104, w105, w106, w107, w108, w109, w110, w71, w70, w69, w68, w67, w66, w65, w64) -> (w63:dbl[][])
            n1531 = Transpose Matrix(1:w63) -> (0:→"Waveform Chart P 2":dbl[][])
          }
        }
      }
    }
  }
  n1532 = local write "path 2_cinetica"(path "C:/H2_Painel/painel_auto/cinetica.txt" ("path")) -> ()
  n1533 = local write "path RLC_completo"(path "C:/H2_Painel/painel_auto/RLC_full.txt" ("path RLC_mean")) -> ()
  n1534 = local write "path RLC_mean"(path "C:/H2_Painel/painel_auto/RLC_mean.txt" ("path RLC_mean")) -> ()
  n1535 = local write "path"(path "C:/H2_Painel/painel_auto/Arquivo_Padrao.txt" ("path")) -> ()
  n1536 = local write "Array"(dbl[] [0.5, 1.0, 2.0, 3.0, 4.0, 4.0, 4.0, 4.0, 4.0, 4.0, 4.0, 5.0, 5.0, 5.0, 7.0, 10.0, 15.0, 20.0, 25.0, 25.0, 25.0, 30.0, 40.0, 50.0, 60.0, 70.0] ("Array")) -> ()
